vi "main_control_YJtoy_V3.vi"() -> ()   [LabVIEW 2021]
uses:
  Addons/DAQ_Pulse_Gen/DAQ_Control_2.ctl
  Addons/DAQ_Pulse_Gen/DAQ_Control_1.ctl
  Ver_2/Config_File_Paths_v2.ctl
  Ver_2/ZI_Data_v2.ctl
  Addons/DAQ_Pulse_Gen/DAQ_Control_3 .ctl
  <vilib>/Utility/file.llb/Write Delimited Spreadsheet (DBL).vi
  <vilib>/gmath/NumericalOptimization/Nonlinear Curve Fit LM formula string.vi
  <vilib>/Utility/error.llb/Error Cluster From Error Code.vi
  <vilib>/ErrorRing/Error Ring.xnode
  <vilib>/Utility/Data Type/NI_Data Type.lvlib
  <vilib>/Analysis/NI_AALPro.lvlib
  <vilib>/gmath/NI_Gmath.lvlib
panel:
  out "appended array":dbl[][](array[numeric])
  out "Initial State Numbers":i32
  out "Process name":string
  out "Initial_state_name":string
  out "tomography rotation memory (priv) 2":cluster{"Time":dbl[], dbl[]}[](array[cluster])
  out "MaxTime":dbl
  out "Process Array":cluster{"Timing 0":dbl[]}[](array[cluster])
  out "tomography rotation memory (priv)":cluster{"Time":dbl[], dbl[]}[](array[cluster])
  in  "pulses type (priv)":string[](array[string])=["None", "Y pi/2", "X pi/2"]
  in  "stop":bool
  in  "Tab Control":T1(tab)=enum."Design QPT"
  out "Config folder":string
  out "Chennel names\nare correct (?)":bool
  out "Channel map":map{string, i32}(c390)
  out "Pulses map [us]":map{string, dbl}(c390)
  out "Sampling data":T2={"Sample Numbers"=20000000, "Sample  Frequency (Hz)"=20000000}
  out "Resource Address":T3={"ZI Address"="DEV714", "VISA Keithley"="KEITHLEY"}
  in  "Save multi-process":bool
  in  "Period number":u32
  in  "Period [us]":dbl
  in  "Name of state (initial_state_)":string
  in  "Name of initial_state":u16(ring) items=["initial_state_01", "initial_state_02", "initial_state_03", "initial_state_04", "initial_state_05", "initial_state_06", "initial_state_07", "initial_state_08", "initial_state_09", "initial_state_10"]
  in  "Run tomography":bool
  in  "Run single FID":bool
  in  "Save for tomography":bool
  in  "Save single sequence":bool
  out "Pulses chart":cluster{dbl[], dbl[]}[](graph)
  in  "Reset sequence":bool
  in  "Channel":u16(ring) items=["LD pump", "LD repump", "LD probe", "pulse X", "pulse Y", "pulse Z", "Keithley ARM", "Keithley TRIG", "Accqusition TRIG", "Nonlinear coil", "None", "Tensor light shift", "pulse ZG", "AI_NI TRIG"]
  in  "Add pulse advanced":bool
  in  "Physical channels":string[](array[string])
  in  "Add pulse":bool
  in  "Time [us]":dbl
  in  "Z pi/2":bool
  in  "Z pi":bool
  in  "Y pi/2":bool
  in  "Y pi":bool
  in  "X pi/2":bool
  in  "X pi":bool
  in  "Add pumping":bool
  in  "Pumping":T4(ring)
  in  "AOC":bool
  in  "X pi/4":bool
  in  "Save initial state":bool
  in  "Save  process":bool
  in  "Name of process (process_)":string
  in  "Name of process":u16(ring) items=["process_01", "process_02", "process_03", "process_04", "process_05", "process_06", "process_07", "process_08", "process_09", "process_10"]
  in  "Y pi/4":bool
  in  "Z pi/4":bool
  in  "Save multi Sequence":bool
  in  "Clear All processes":bool
  in  "Show Process_List":bool
  in  "Delete the Process":bool
  in  "Run QPT":bool
  in  "initial_state_show":u16(ring) items=["initial_state_01.ini", "initial_state_02.ini", "initial_state_03.ini", "initial_state_04.ini", "initial_state_05.ini", "initial_state_06.ini", "initial_state_07.ini", "initial_state_08.ini", "initial_state_09.ini", "initial_state_10.ini", "initial_state_11.ini"]
  in  "Choose init states":bool
  in  "State_update":bool
  out "State_List":string[](array[string]) caption="The Choosen States"
  in  "Delete init states":bool
  in  "Show init state":bool
  in  "Process_update":bool
  in  "Process_show":u16(ring) caption="initial_state_show" items=["process_01.ini", "process_02.ini", "process_03.ini"]
  out "Pulses chart 2":cluster{dbl[], dbl[]}[](graph)
  out "Pulses chart 3":cluster{dbl[], dbl[]}[](graph)
  in  "Save QPT":bool
  in  "Clear All states":bool
  out "Process_List":string[](array[string]) caption="The Choosen Process"
  in  "Choose the Process":bool
  in  "Multi-FID":bool
  in  "save":bool
  out "Rotation signal 3":cluster{"Time":dbl[], "Array":dbl[]}[](graph)
  out "w":dbl format="%#_3f"
  out "q":dbl format="%#_3f"
  out "g2":dbl format="%#_3f"
  out "g1":dbl format="%#_3f"
  out "C":dbl format="%#_3f"
  out "B":dbl format="%#_3f"
  out "A":dbl format="%#_3f"
  in  "Enum":T5(ring)
  in  "Fit model":bool
  out "Rotation signal":cluster{"Time":dbl[], dbl[]}(graph)
  out "Rotation spectrum":waveform(dbl)[](graph)
  out "Differential signal":cluster{"Time":dbl[], "X":dbl[]}[](graph)
  out "Intensity signal":cluster{"Time":dbl[], dbl[]}(graph)
  out "Polarimeter":dbl(knob) scale=-10.0..10.0
  in  "Run single FID 2":bool
  out "Progress":dbl(slide) scale=0.0..100.0
  in  "Number of repetition":u32=1 min=1 step=1
  in  "Signal in X or Y (?)":bool
  in  "Plot type":u16(ring) items=["None + [ None ]", "None + [ Y pi ]", "None + [ Z(pi/2)+Y(pi) ]", "Y pi/2 + [ None ]", "Y pi/2 + [ Y pi ]", "Y pi/2 + [ Z(pi/2)+Y(pi) ]", "X pi/2 + [ None ]", "X pi/2 + [ Y pi ]", "X pi/2 + [ Z(pi/2)+Y(pi) ]"]
  in  "Save raw data (?)":bool
  in  "Save CYCLOPS data (?)":bool
  out "Rotation signal":cluster{"Time":dbl[], dbl[]}(graph)
  in  "Run tomography 2":bool
  in  "Averaging":u8=1 min=1 step=1
  out "Differential signal":cluster{"Time":dbl[], "X":dbl[]}[](graph)
  out "Intensity signal":cluster{"Time":dbl[], dbl[]}(graph)
  out "Progress":dbl(slide) scale=0.0..100.0
  out "Rotation spectrum":waveform(dbl)[](graph)
  out "Rotation":cluster{"Time":dbl[], dbl[]}(graph)
  in  "Save raw data  2":bool
  in  "Save CYCLOPS data 2":bool
  out "Rotation spectrum 2":waveform(dbl)[](graph)
  out "Rotation signal 2":cluster{"Time":dbl[], dbl[]}(graph)
  out "Differential signal 2":cluster{"Time":dbl[], "X":dbl[]}[](graph)
  out "Intensity signal 2":cluster{"Time":dbl[], dbl[]}(graph)
  out "Single Tomography Progress":dbl(slide) scale=0.0..100.0
  out "Rotation 2":cluster{"Time":dbl[], dbl[]}(graph)
  in  "Averaging 2":u8=1 min=1 step=1
  in  "Run QPT 2":bool
  out "Current_QPT_order":i32
  out "QPT Progress":dbl(slide) scale=0.0..100.0
  # "To change that tab you need to go to block diagram"
  # "Probing will be added during saving"
  # "X"
  # "Y"
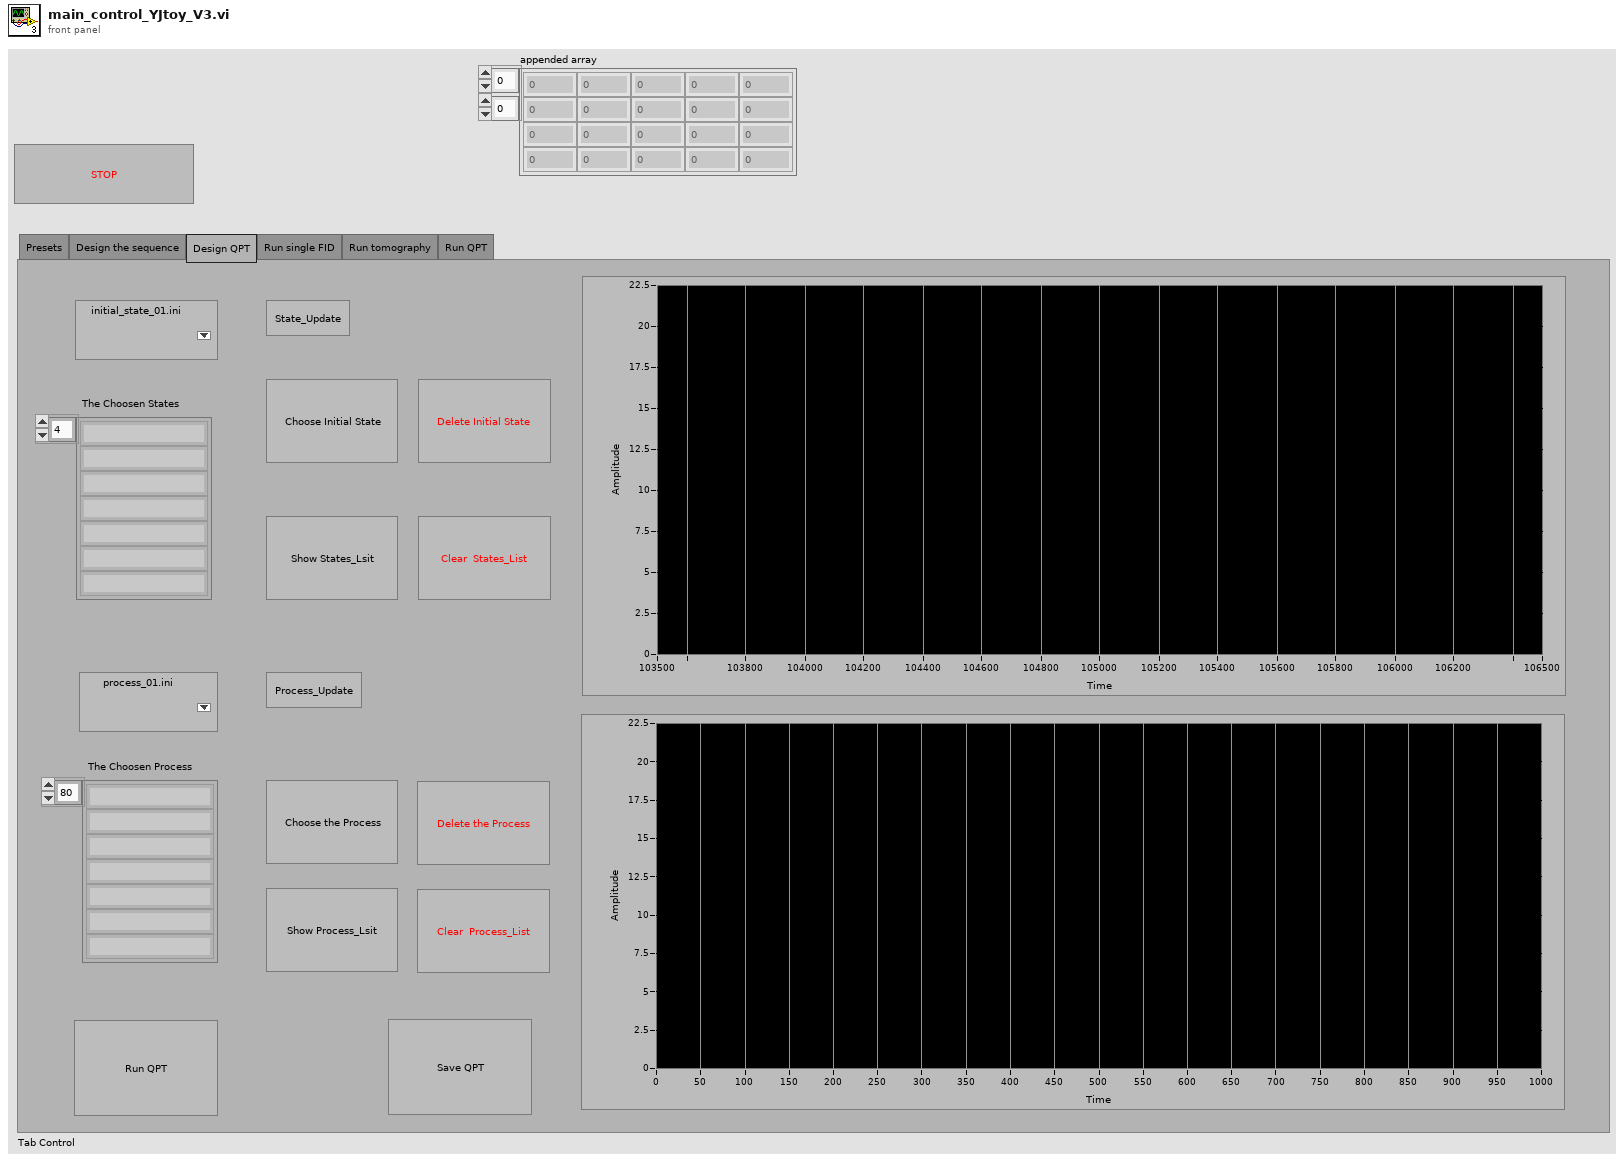
[diagram p1: front panel]
types:
  T1 = enum32{"Presets", "Design the sequence", "Design QPT", "Run single FID", "Run tomography", "Run QPT"}
  T2 = typedef "DAQ_Control_2.ctl" = cluster{"Sample Numbers":u32, "Sample  Frequency (Hz)":u32}
  T3 = cluster{"ZI Address":string, "VISA Keithley":refnum<visa-resource-name>}
  T4 = enum16{"Circular along X", "Linear in Y", "Linear in Z"}
  T5 = enum16{"Full", "A*Sin(w*t+q)*Exp(-g1*t)+C", "B*Exp(-q2*t)+C"}
  T6 = typedef "DAQ_Control_1.ctl" = cluster{"Port 2/line 6":cluster{"Timing 22":dbl[]}, "Port 2/line 5":cluster{"Timing 21":dbl[]}, "Port 2/line 4":cluster{"Timing 20":dbl[]}, "Port 2/line 3":cluster{"Timing 19":dbl[]}, "Port 2/line 2":cluster{"Timing 18":dbl[]}, "Port 2/line 1":cluster{"Timing 17":dbl[]}, "Port 2/line 0":cluster{"Timing 16":dbl[]}, "Port 1/line 7":cluster{"Timing 15":dbl[]}, "Port 1/line 6":cluster{"Timing 14":dbl[]}, "Port 1/line 5":cluster{"Timing 13":dbl[]}, "Port 1/line 4":cluster{"Timing 12":dbl[]}, "Port 1/line 3":cluster{"Timing 11":dbl[]}, "Port 1/line 2":cluster{"Timing 10":dbl[]}, "Port 1/line 1":cluster{"Timing 9":dbl[]}, "Port 1/line 0":cluster{"Timing 8":dbl[]}, "Port 0/line 7":cluster{"Timing 7\n":dbl[]}, "Port 0/line 6":cluster{"Timing 6\n":dbl[]}, "Port 0/line 5":cluster{"Timing 5\n":dbl[]}, "Port 0/line 4":cluster{"Timing 4\n":dbl[]}, "Port 0/line 3":cluster{"Timing 3\n":dbl[]}, "Port 0/line 2":cluster{"Timing 2":dbl[]}, "Port 0/line 1":cluster{"Timing 1\n":dbl[]}, "Port 0/line 0":cluster{"Timing 0":dbl[]}}
  T7 = typedef "Config_File_Paths_v2.ctl" = cluster{"ZI config file (.ini)":string, "Keithley config file (.ini)":string, "DAQ config file (.ini)":string}
  T8 = enum32{"Presets", "Design the sequence", "Design QPT", "Run single FID"}
  T9 = enum8{"Enabled", "Disabled", "Disabled and Grayed Out"}
  T10 = enum32{"Presets", "Design the sequence", "Design QPT", "Run single FID", "Run tomography"}
  T11 = cluster{"model":string, "Parameters":string[], "x":string}
  T12 = typedef "DAQ_Control_3 .ctl" = cluster{"Time Unit":enum16{"NanoSecond", "MicroSecond", "MilliSecond"}}
  T13 = typedef "ZI_Data_v2.ctl" = cluster{"R":dbl[], "Theta":dbl[], "X":dbl[], "Y":dbl[], "AuxIn0":dbl[], "AuxIn1":dbl[], "Frequency":dbl[], "DIO":dbl[], "Time":dbl[]}
  T14 = typedef "Resources_v2.ctl" = cluster{"ZI Handle":T15, "ZI ModHandle":T16, "VISA Keithley":refnum<visa-resource-name>}
  T15 = typedef "Zurich Instruments LabOne.lvlib/ziTypeHandle.ctl" = cluster{"handleValid":bool, "Conn":u64, "Path Prefix":string, "Handle":u64, "Clockbase(s)":dbl, "Connected":bool}
  T16 = typedef "Zurich Instruments LabOne.lvlib/ziTypeModHandle.ctl" = cluster{"handleValid":bool, "Conn":u64, "ModHandle":u64, "moduleID":string, "Path Prefix":string}
  T17 = typedef "Cutted_Data_v2.ctl" = cluster{"X":dbl[], "Y":dbl[], "Time":dbl[]}
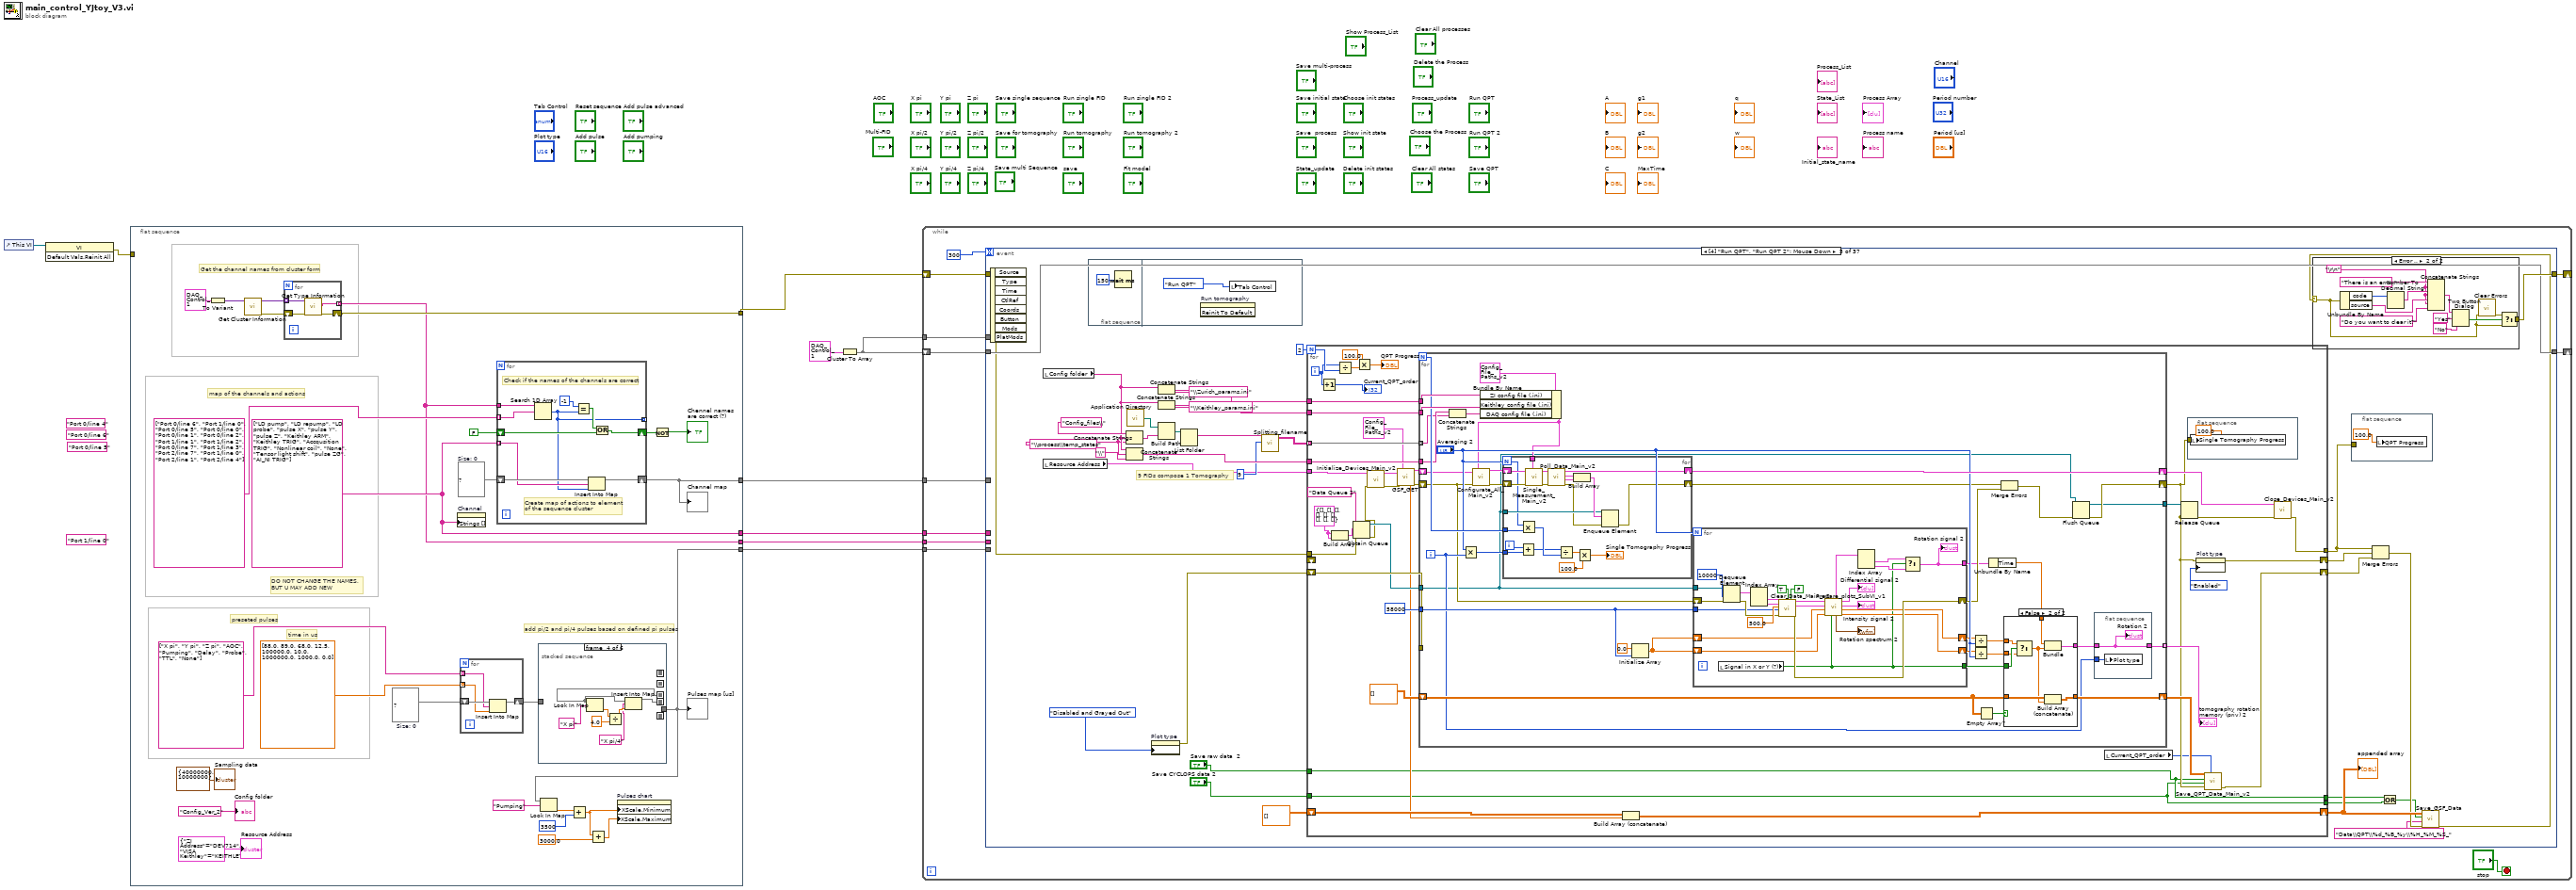
[diagram p0: block diagram]
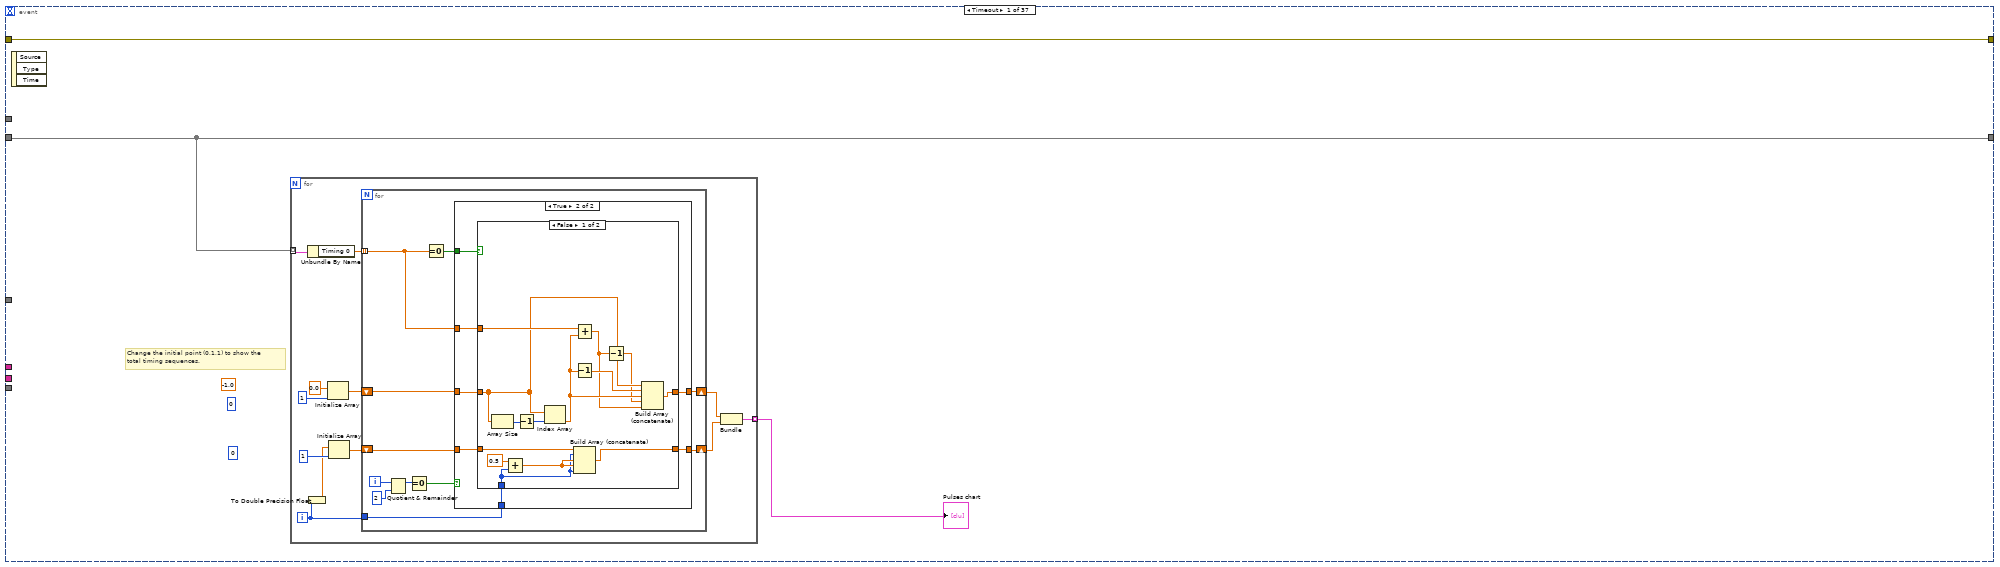
[diagram p2: hidden frame]
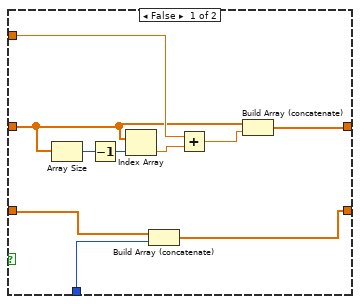
[diagram p3: hidden frame]
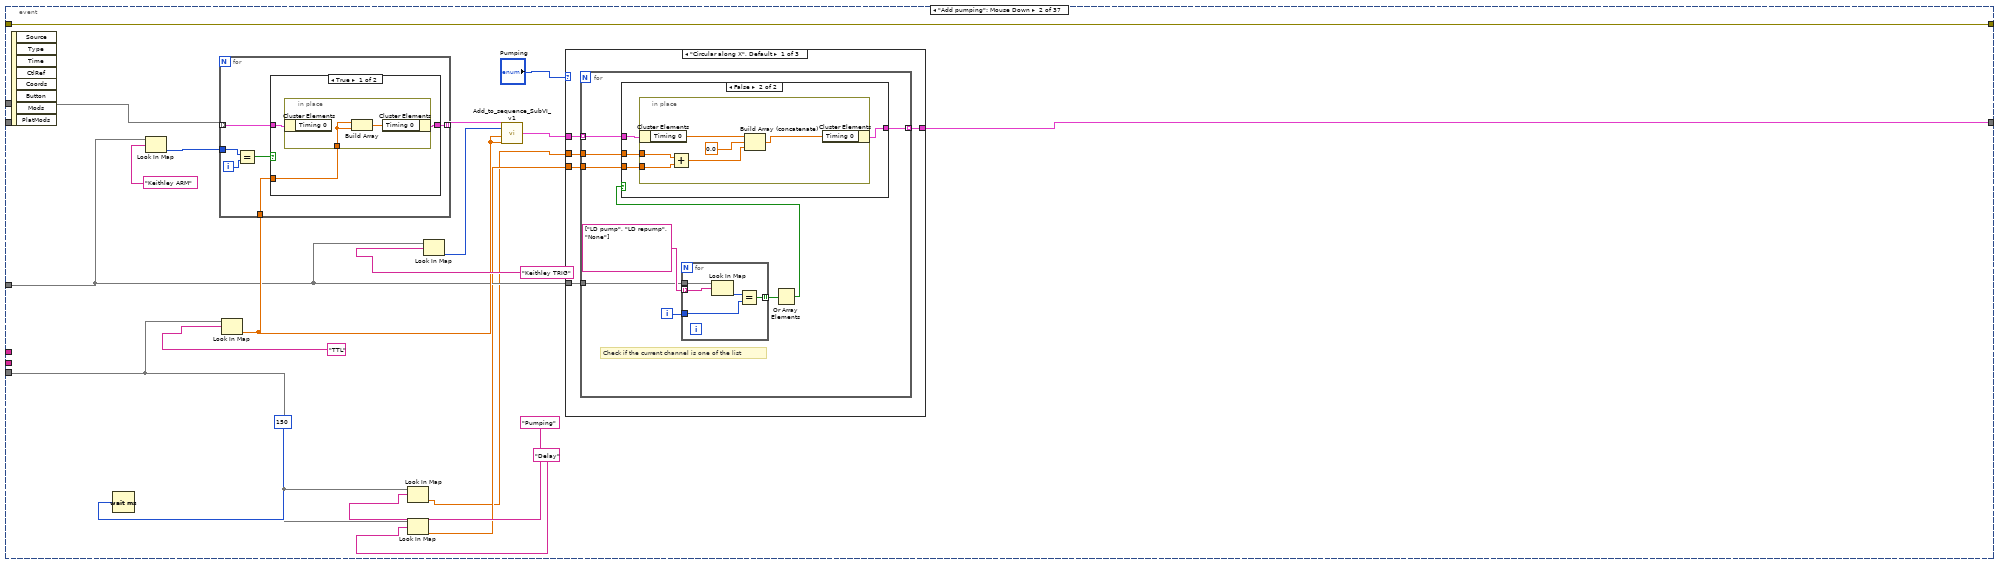
[diagram p5: hidden frame]
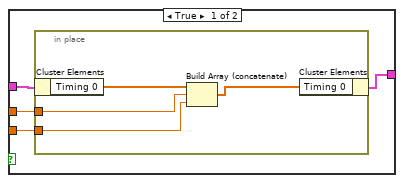
[diagram p6: hidden frame]
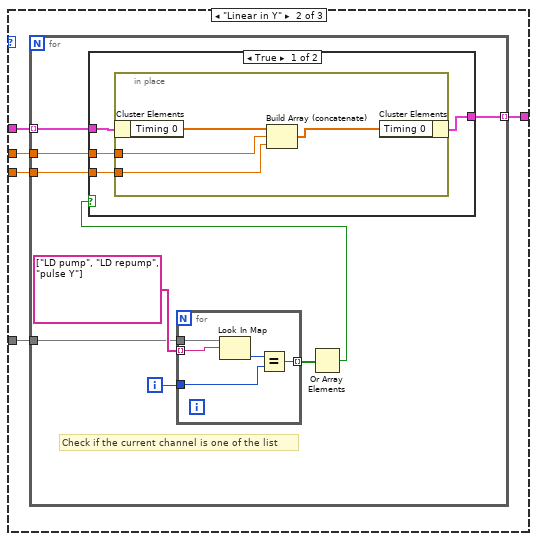
[diagram p7: hidden frame]
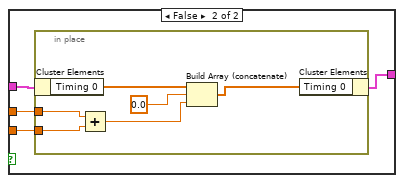
[diagram p8: hidden frame]
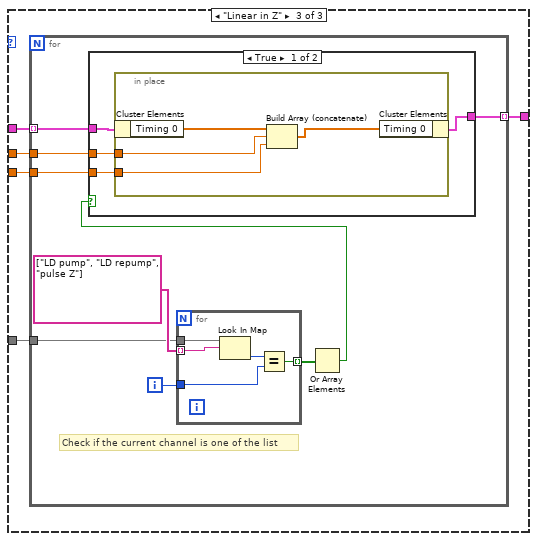
[diagram p9: hidden frame]
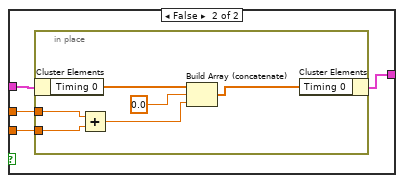
[diagram p10: hidden frame]
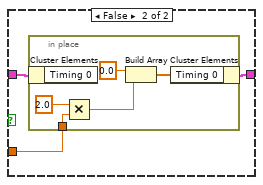
[diagram p11: hidden frame]
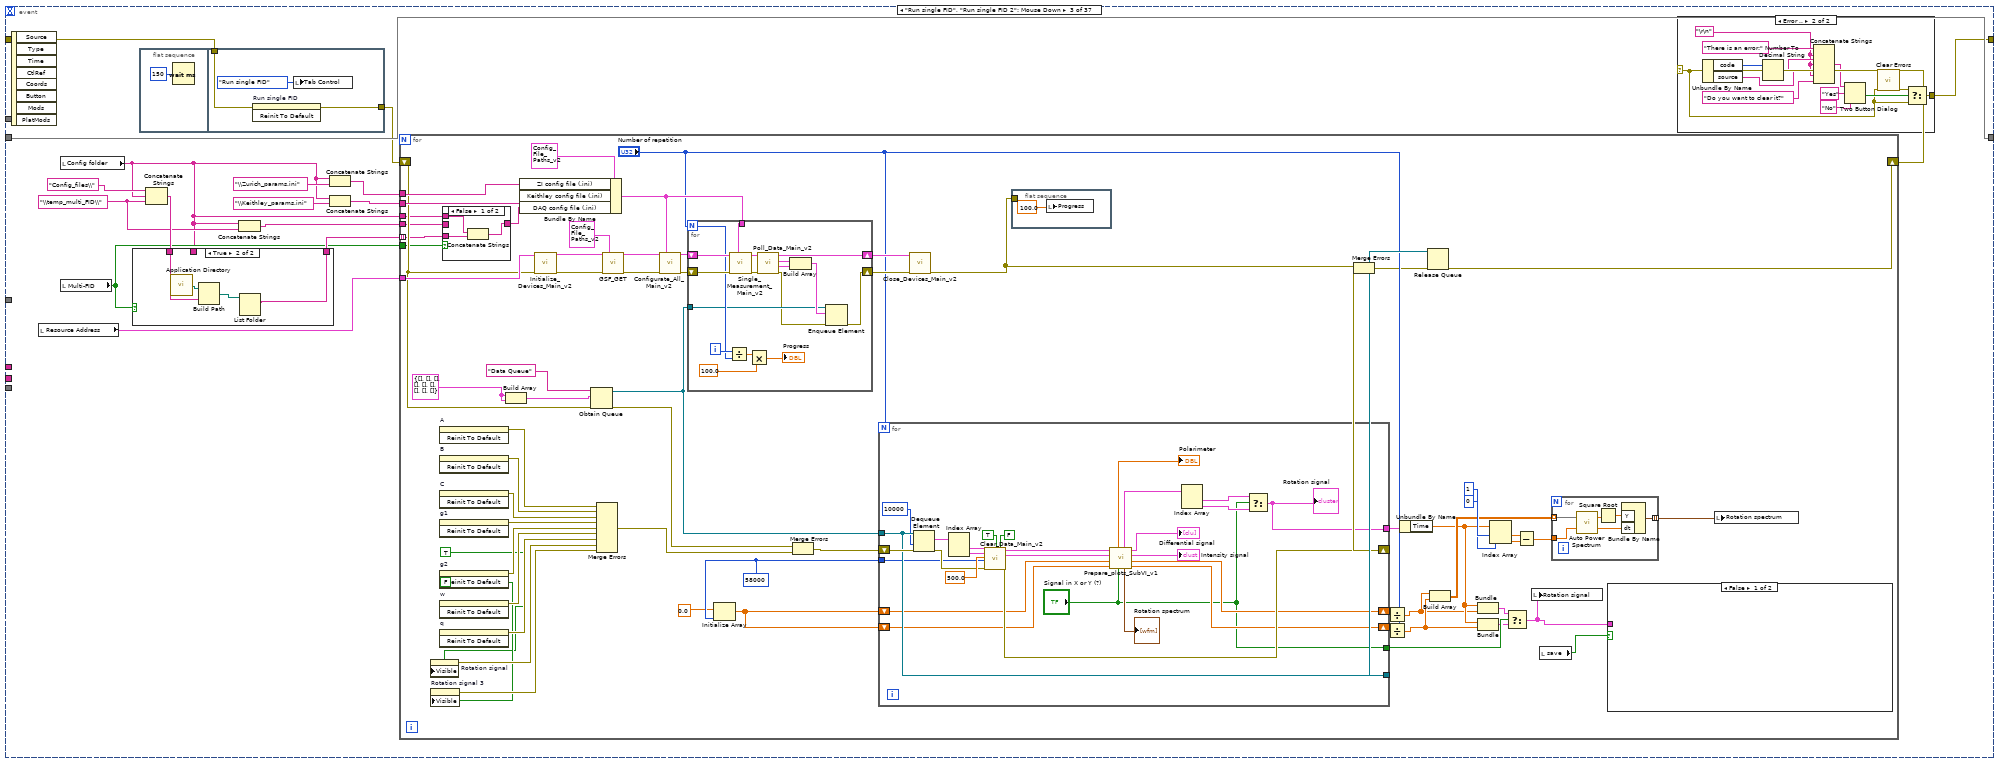
[diagram p12: hidden frame]
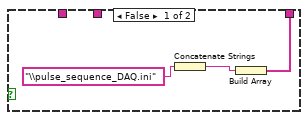
[diagram p13: hidden frame]
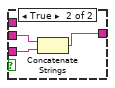
[diagram p14: hidden frame]
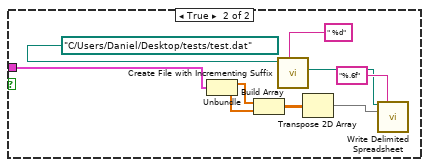
[diagram p15: hidden frame]
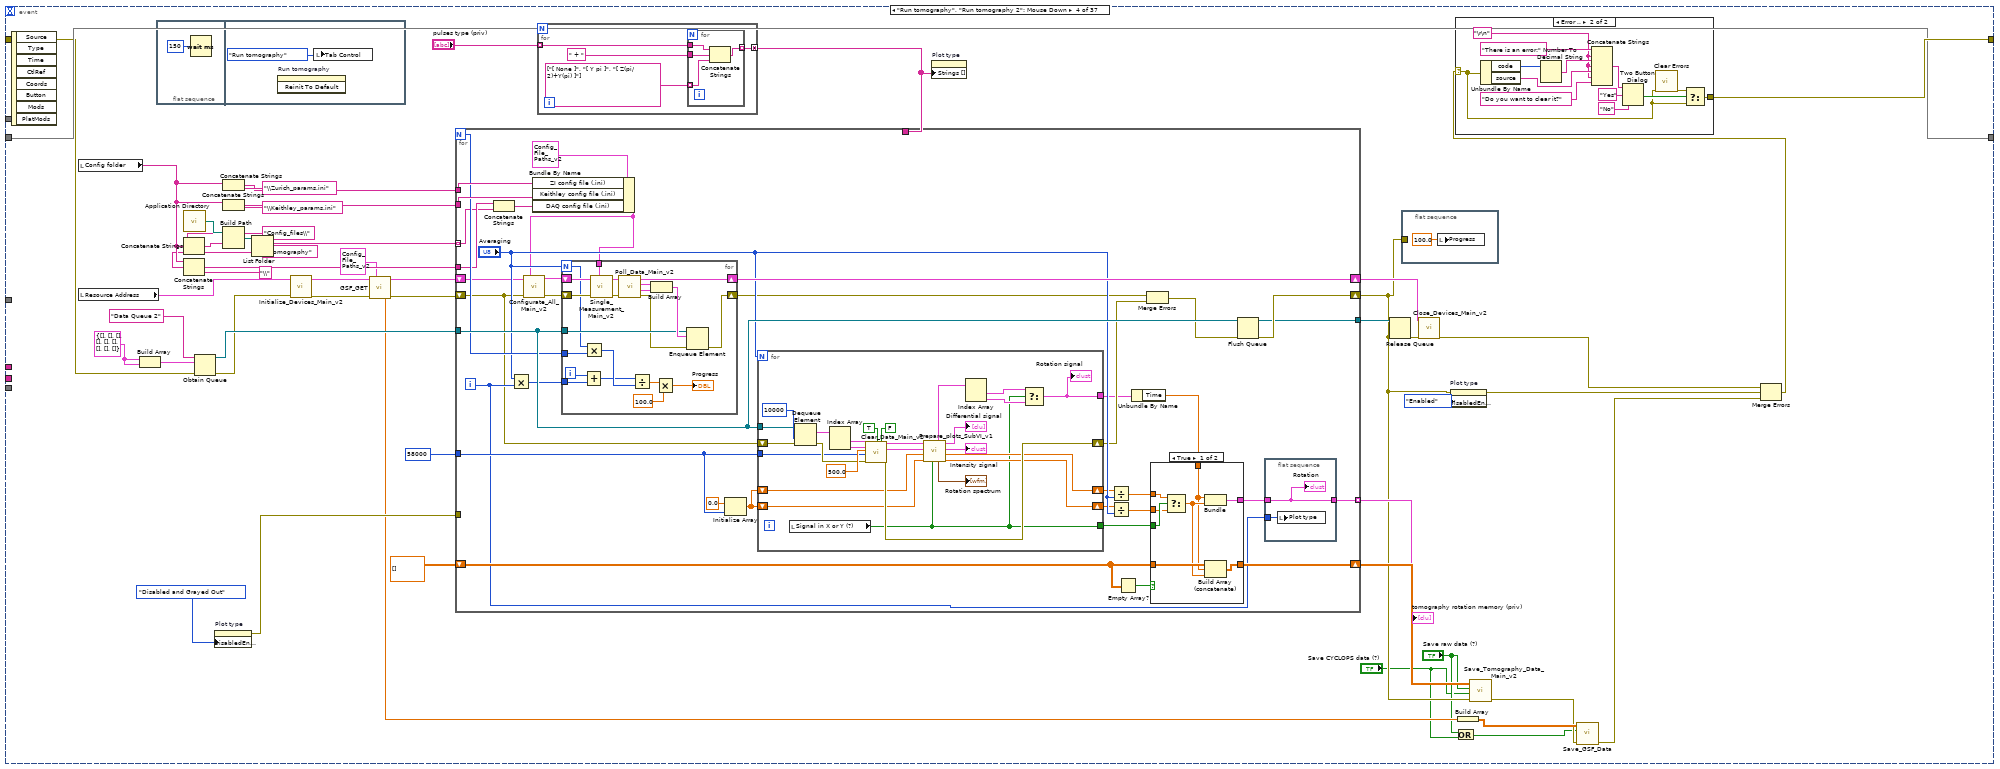
[diagram p17: hidden frame]
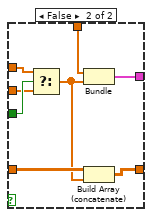
[diagram p18: hidden frame]
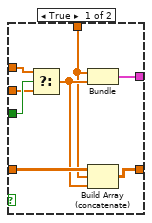
[diagram p20: hidden frame]
diagram:
  (unwired) "Port 0/line 5"
  (unwired) "Port 0/line 4"
  (unwired) "Port 1/line 0"
  (unwired) "Port 0/line 6"
  n1 = control-ref of="This VI"() -> (w2:refnum<vi>)
  n2 = invoke class="VI" method="Default Vals.Reinit All"(reference=w2) -> (error out=w1:errorcluster)  [unwired: 2 in, 2 out]
  n3 = flat-sequence {
    tunnel: [w23] -> w8
    tunnel: [w17] -> w7
    tunnel: [w22] -> w6
    tunnel: [w21] -> w5
    tunnel: [w20] -> w4
    tunnel: w1 -> [_]
    frame #0 {
      w27 = map{string, dbl} {}  # Size: 0
      w29 = map{string, i32} {}  # Size: 0
      w21 = string[] ["LD pump", "LD repump", "LD probe", "pulse X", "pulse Y", "pulse Z", "Keithley ARM", "Keithley TRIG", "Accqusition TRIG", "Nonlinear coil", "None", "Tensor light shift", "pulse ZG", "AI_NI TRIG"]
      # "DO NOT CHANGE THE NAMES,\nBUT U MAY ADD NEW"
      # "add pi/2 and pi/4 pulses based on defined pi pulses"
      # "preseted pulses"
      # "time in us"
      # "map of the channels and actions"
      # "Get the channel names from cluster form"
      n4 = To Variant(anything=T6 {"Port 2/line 6"={"Timing 22"=[]}, "Port 2/line 5"={"Timing 21"=[]}, "Port 2/line 4"={"Timing 20"=[]}, "Port 2/line 3"={"Timing 19"=[]}, "Port 2/line 2"={"Timing 18"=[]}, "Port 2/line 1"={"Timing 17"=[]}, "Port 2/line 0"={"Timing 16"=[]}, "Port 1/line 7"={"Timing 15"=[]}, "Port 1/line 6"={"Timing 14"=[]}, "Port 1/line 5"={"Timing 13"=[]}, "Port 1/line 4"={"Timing 12"=[]}, "Port 1/line 3"={"Timing 11"=[]}, "Port 1/line 2"={"Timing 10"=[]}, "Port 1/line 1"={"Timing 9"=[]}, "Port 1/line 0"={"Timing 8"=[]}, "Port 0/line 7"={"Timing 7\n"=[]}, "Port 0/line 6"={"Timing 6\n"=[]}, "Port 0/line 5"={"Timing 5\n"=[]}, "Port 0/line 4"={"Timing 4\n"=[]}, "Port 0/line 3"={"Timing 3\n"=[]}, "Port 0/line 2"={"Timing 2"=[]}, "Port 0/line 1"={"Timing 1\n"=[]}, "Port 0/line 0"={"Timing 0"=[]}} ("Sequence")) -> (Variant=w35:variant)
      n5 = call <vilib>:"Get Cluster Information.vi"("variant"=w35) -> ("error out"=w34:errorcluster, "cluster elements"=w33:variant[])  [unwired: 9 in]
      n6 = for {
        tunnel: w33 -> [w96] mode=indexing
        shift-right: [w94] -> w22
        shift-left: w34 -> [w95]
        tunnel: [w93] -> w20 mode=indexing
        n7 = call <vilib>:"Get Type Information.vi"("error in (no error)"=w95, "variant"=w96) -> ("error out"=w94:errorcluster, "name"=w93:string)  [unwired: 5 in, 3 out]
      }
      n8 = property on="Channel" class="Ring (strict)"("Strings []"=w21) -> ()  [unwired: 2 in, 2 out]
      n9 = for {
        shift-right: [w79] -> w24
        shift-left: w27 -> [w82]
        tunnel: string[] ["X pi", "Y pi", "Z pi", "AOC", "Pumping", "Delay", "Probe", "TTL", "None"] -> [w81] mode=indexing
        tunnel: dbl[] [88.0, 89.0, 68.0, 12.5, 100000.0, 10.0, 1000000.0, 1000.0, 0.0] -> [w80] mode=indexing
        n10 = Insert Into Map(map in=w82, key=w81, value=w80) -> (map out=w79:map{string, dbl})  [unwired: 2 out]
      }
      n11 = for {
        tunnel: w20 -> [w92]
        tunnel: string[] ["Port 0/line 6", "Port 1/line 0", "Port 0/line 5", "Port 0/line 0", "Port 0/line 1", "Port 0/line 2", "Port 1/line 1", "Port 1/line 2", "Port 0/line 7", "Port 1/line 3", "Port 2/line 7", "Port 1/line 0", "Port 2/line 1", "Port 2/line 4"] -> [w83] mode=indexing
        shift-right: [w88] -> w31
        shift-left: FALSE -> [w89]
        tunnel: [w85] -> _ mode=indexing
        shift-right: [w84] -> w23
        shift-left: w29 -> [w87]
        tunnel: w21 -> [w86] mode=indexing
        # "Create map of actions to element\nof the sequence cluster"
        # "Check if the names of the channels are correct"
        n12 = Search 1D Array(1D array=w92, element=w83) -> (index of element=w85:i32)  [unwired: 1 in]
        n13 = Equal?(x=-1, y=w85) -> (x = y?=w90:bool)
        n14 = Insert Into Map(map in=w87, key=w86, value=w85) -> (map out=w84:map{string, i32})  [unwired: 2 out]
        n15 = Or(x=w90, y=w89) -> (x .or. y?=w88:bool)
      }
      "Channel map" <- w23
      n16 = stacked-sequence {
        seq-local: [w37 _ _ _ _ _] -> [_ w44 _ _ _ _]
        seq-local: [_ w45 _ _ _ _] -> [_ _ w52 _ _ _]
        seq-local: [_ _ w51 _ _ _] -> [_ _ _ w63 _ _]
        seq-local: [_ _ _ w59 _ _] -> [_ _ _ _ w71 _]
        seq-local: [_ _ _ _ w70 _] -> [_ _ _ _ _ w78]
        tunnel: w24 -> [w41 _ _ _ _ _]
        tunnel: [_ _ _ _ _ w77] -> w17
        frame #0 {
          n17 = Look In Map(map=w41, key="X pi") -> (value=w39:dbl)  [unwired: 1 in, 1 out]
          n18 = Divide(x=w39, y=2.0) -> (x/y=w40:dbl)
          n19 = Insert Into Map(map in=w41, key="X pi/2", value=w40) -> (map out=w37:map{string, dbl})  [unwired: 2 out]
        }
        frame #1 {
          n20 = Look In Map(map=w44, key="Y pi") -> (value=w50:dbl)  [unwired: 1 in, 1 out]
          n21 = Divide(x=w50, y=2.0) -> (x/y=w49:dbl)
          n22 = Insert Into Map(map in=w44, key="Y pi/2", value=w49) -> (map out=w45:map{string, dbl})  [unwired: 2 out]
        }
        frame #2 {
          n23 = Look In Map(map=w52, key="Z pi") -> (value=w54:dbl)  [unwired: 1 in, 1 out]
          n24 = Divide(x=w54, y=2.0) -> (x/y=w55:dbl)
          n25 = Insert Into Map(map in=w52, key="Z pi/2", value=w55) -> (map out=w51:map{string, dbl})  [unwired: 2 out]
        }
        frame #3 {
          n26 = Look In Map(map=w63, key="X pi") -> (value=w62:dbl)  [unwired: 1 in, 1 out]
          n27 = Divide(x=w62, y=4.0) -> (x/y=w60:dbl)
          n28 = Insert Into Map(map in=w63, key="X pi/4", value=w60) -> (map out=w59:map{string, dbl})  [unwired: 2 out]
        }
        frame #4 {
          n29 = Look In Map(map=w71, key="Y pi") -> (value=w68:dbl)  [unwired: 1 in, 1 out]
          n30 = Divide(x=w68, y=4.0) -> (x/y=w66:dbl)
          n31 = Insert Into Map(map in=w71, key="Y pi/4", value=w66) -> (map out=w70:map{string, dbl})  [unwired: 2 out]
        }
        frame #5 {
          n32 = Look In Map(map=w78, key="Z pi") -> (value=w75:dbl)  [unwired: 1 in, 1 out]
          n33 = Divide(x=w75, y=4.0) -> (x/y=w73:dbl)
          n34 = Insert Into Map(map in=w78, key="Z pi/4", value=w73) -> (map out=w77:map{string, dbl})  [unwired: 2 out]
        }
      }
      "Pulses map [us]" <- w17
      n35 = Look In Map(map=w17, key="Pumping") -> (value=w19:dbl)  [unwired: 1 in, 1 out]
      n36 = Add(x=w19, y=3500) -> (x+y=w16:dbl)
      n37 = Add(x=w16, y=3000.0) -> (x+y=w14:dbl)
      n38 = property on="Pulses chart" class="XYGraph (strict)"("XScale.Minimum"=w16, "XScale.Maximum"=w14) -> ()  [unwired: 2 in, 2 out]
      n39 = Not(x=w31) -> (.not. x?=→"Chennel names\nare correct (?)":bool)
      "Sampling data" <- T2 {"Sample Numbers"=40000000, "Sample  Frequency (Hz)"=10000000} ("Sampling data")
      "Config folder" <- "Config_Ver_2" ("Filename (ini)")
      "Resource Address" <- T3 {"ZI Address"="DEV714", "VISA Keithley"="KEITHLEY"} ("Resource Address")
    }
  }
  n40 = Cluster To Array(cluster=T6 {"Port 2/line 6"={"Timing 22"=[]}, "Port 2/line 5"={"Timing 21"=[]}, "Port 2/line 4"={"Timing 20"=[]}, "Port 2/line 3"={"Timing 19"=[]}, "Port 2/line 2"={"Timing 18"=[]}, "Port 2/line 1"={"Timing 17"=[]}, "Port 2/line 0"={"Timing 16"=[]}, "Port 1/line 7"={"Timing 15"=[]}, "Port 1/line 6"={"Timing 14"=[]}, "Port 1/line 5"={"Timing 13"=[]}, "Port 1/line 4"={"Timing 12"=[]}, "Port 1/line 3"={"Timing 11"=[]}, "Port 1/line 2"={"Timing 10"=[]}, "Port 1/line 1"={"Timing 9"=[]}, "Port 1/line 0"={"Timing 8"=[]}, "Port 0/line 7"={"Timing 7\n"=[]}, "Port 0/line 6"={"Timing 6\n"=[]}, "Port 0/line 5"={"Timing 5\n"=[]}, "Port 0/line 4"={"Timing 4\n"=[]}, "Port 0/line 3"={"Timing 3\n"=[]}, "Port 0/line 2"={"Timing 2"=[]}, "Port 0/line 1"={"Timing 1\n"=[]}, "Port 0/line 0"={"Timing 0"=[]}} ("Sequence")) -> (array=w3:cluster{"Timing 0":dbl[]}[])
  n41 = while {
    shift-right: [w98] -> _
    shift-left: w3 -> [w107]
    tunnel: w8 -> [w106]
    tunnel: w7 -> [w97]
    shift-right: [w102] -> _
    shift-left: w6 -> [w103]
    tunnel: w5 -> [w101]
    tunnel: w4 -> [w100]
    tunnel: w3 -> [w99]
    stop <- "stop" stop-if-true
    n42 = event shown="[4] \"Run QPT\", \"Run QPT 2\": Mouse Down" {
      selector: _ -> [_ _ _ _ _ _ _ _ _ _ _ _ _ _ _ _ _ _ _ _ _ _ _ _ _ _ _ _ _ _ _ _ _ _ _ _ _]
      dyn-events: _ -> [_ _ _ _ _ _ _ _ _ _ _ _ _ _ _ _ _ _ _ _ _ _ _ _ _ _ _ _ _ _ _ _ _ _ _ _ _]
      timeout: 300 -> [_ _ _ _ _ _ _ _ _ _ _ _ _ _ _ _ _ _ _ _ _ _ _ _ _ _ _ _ _ _ _ _ _ _ _ _ _]
      tunnel: w107 -> [w110 _ w327 w530 w693 w862 _ w1025 w1030 w1042 w1053 w1065 w1077 w1089 w1101 w1113 w1125 w1142 w1170 w1209 w1290 w1421 w1475 w1617 w1664 _ _ _ _ _ _ _ _ _ _ _ _]
      tunnel: w106 -> [_ w172 _ _ _ _ _ w1009 w1037 w1049 w1060 w1072 w1084 w1096 w1108 w1120 w1132 w1147 _ w1222 w1292 w1423 w1480 _ _ w1737 _ _ _ _ _ _ _ _ _ _ _]
      tunnel: w97 -> [_ w171 _ _ _ _ _ w1007 w1031 w1043 w1058 w1066 w1078 w1090 w1102 w1114 w1126 w1143 w1162 w1219 w1291 w1422 w1479 _ _ w1736 _ _ _ _ _ _ _ _ _ _ _]
      tunnel: [w110 w169 w327 w530 w693 w862 _ w1002 w1029 w1041 w1052 w1064 w1076 w1088 w1100 w1112 w1124 w1141 w1159 w1209 _ _ w1475 w1617 w1664 _ _ _ _ _ _ _ _ _ _ _ w2190] -> w98
      tunnel: w103 -> [w109 w185 w326 w526 w678 w863 w905 w1013 w1033 w1045 _ w1068 w1080 w1092 w1104 w1116 w1128 w1145 w1166 w1204 w1282 w1413 w1473 w1618 w1665 w1720 w1852 w1947 w2045 w2068 w2083 w2104 w2125 w2153 w2181 w2187 w2191]
      tunnel: [w109 w185 w324 w534 w696 w863 _ w1013 w1033 w1045 _ w1068 w1080 w1092 w1104 w1116 w1128 w1145 w1166 w1203 w1289 w1420 w1472 w1619 w1666 w1743 w1851 w1940 w2040 w2063 w2090 w2111 w2122 w2150 w2180 w2186 w2191] -> w102
      tunnel: w101 -> [_ _ _ _ _ _ _ _ _ _ _ _ _ _ _ _ _ w1138 _ _ _ _ _ _ _ _ _ _ _ _ _ _ _ _ _ _ _]
      tunnel: w100 -> [_ _ _ _ _ _ _ _ _ _ _ _ _ _ _ _ _ _ w1168 _ _ _ _ _ _ _ _ _ _ _ _ _ _ _ _ _ _]
      tunnel: w99 -> [_ w168 _ _ _ _ _ _ _ _ _ _ _ _ _ _ _ _ _ _ _ _ _ _ _ _ _ _ _ _ _ _ _ _ _ _ w2190]
      event Timeout {
        (unwired) 0 ("dimension size")
        (unwired) 0 ("dimension size")
        (unwired) -1.0 ("element")
        # "Change the initial point (0,1,1) to show the \ntotal timing sequences."
        n43 = event-data() -> ()  [unwired: 1 in, 3 out]
        n44 = for {
          tunnel: w110 -> [w122] mode=indexing
          tunnel: [w111] -> w108 mode=indexing
          i -> [w114]
          n45 = To Double Precision Float(number=w114) -> (double precision float=w118:dbl)
          n46 = Unbundle By Name(w122) -> ("Timing 0"=w121:dbl[])
          n47 = Initialize Array(0.0 ("element"), 1 ("dimension size")) -> (w115:dbl[])
          n48 = Initialize Array(w118, 1 ("dimension size")) -> (w119:dbl[])
          n49 = for {
            tunnel: w121 -> [w124] mode=indexing
            shift-right: [w126] -> w112
            shift-left: w119 -> [w125]
            shift-right: [w128] -> w113
            shift-left: w115 -> [w127]
            tunnel: w114 -> [w123]
            i -> [w133]
            n50 = Quotient & Remainder(x=w133, y=2) -> (x-y*floor(x/y)=w131:i32)  [unwired: 1 out]
            n51 = Equal To 0?(x=w131) -> (x = 0?=w130:bool)
            n52 = Equal To 0?(x=w124) -> (x = 0?=w129:bool)
            n53 = case shown="True" w130 {
              tunnel: w129 -> [_ w150]
              tunnel: [w134 w149] -> w128
              tunnel: w127 -> [w136 w148]
              tunnel: [w141 w147] -> w126
              tunnel: w125 -> [w142 w146]
              tunnel: w124 -> [w137 w145]
              tunnel: w123 -> [w143 w144]
              frame False {
                n54 = Array Size(array=w136) -> (size(s)=w140:i32)
                n55 = Decrement(x=w140) -> (x-1=w139:i32)
                n56 = Index Array(array=w136, index=w139) -> (element=w138:dbl)
                n57 = Build Array (concatenate)(w142, w143) -> (w141:dbl[])
                n58 = Add(x=w137, y=w138) -> (x+y=w135:dbl)
                n59 = Build Array (concatenate)(w136, w135) -> (w134:dbl[])
              }
              frame True {
                n60 = case shown="False" w150 {
                  tunnel: [w161 w166] -> w149
                  tunnel: w148 -> [w155 w166]
                  tunnel: [w157 w165] -> w147
                  tunnel: w146 -> [w164 w165]
                  tunnel: w145 -> [w162 _]
                  tunnel: w144 -> [w158 _]
                  frame False {
                    n61 = Array Size(array=w155) -> (size(s)=w163:i32)
                    n62 = Add(x=0.5, y=w158) -> (x+y=w159:dbl)
                    n63 = Decrement(x=w163) -> (x-1=w156:i32)
                    n64 = Index Array(array=w155, index=w156) -> (element=w153:dbl)
                    n65 = Add(x=w162, y=w153) -> (x+y=w152:dbl)
                    n66 = Decrement(x=w153) -> (x-1=w154:dbl)
                    n67 = Build Array (concatenate)(w164, w158, w159, w159, w158) -> (w157:dbl[])
                    n68 = Decrement(x=w152) -> (x-1=w151:dbl)
                    n69 = Build Array (concatenate)(w155, w154, w153, w151, w152) -> (w161:dbl[])
                  }
                  frame True {
                  }
                }
              }
            }
          }
          n70 = Bundle(w113, w112) -> (w111:cluster{dbl[], dbl[]})  [unwired: 1 in]
        }
        "Pulses chart" <- w108
      }
      event "Add pumping": Mouse Down {
        n71 = event-data() -> ()  [unwired: 1 in, 8 out]
        n72 = Wait (ms)(milliseconds to wait=u32 150) -> ()  [unwired: 1 out]
        n73 = Look In Map(map=w172, key="Keithley ARM") -> (value=w182:i32)  [unwired: 1 in, 1 out]
        n74 = Look In Map(map=w171, key="TTL") -> (value=w177:dbl)  [unwired: 1 in, 1 out]
        n75 = for {
          tunnel: w168 -> [w299] mode=indexing
          tunnel: w182 -> [w301]
          tunnel: w177 -> [w298]
          tunnel: [w297] -> w180 mode=indexing
          i -> [w302]
          n76 = Equal?(x=w301, y=w302) -> (x = y?=w300:bool)
          n77 = case shown="True" w300 {
            tunnel: w299 -> [w305 w310]
            tunnel: w298 -> [w304 w309]
            tunnel: [w303 w308] -> w297
            frame True {
              n78 = in-place {
                in-place-border: w304 -> [w307]
                n79 = in-place-cluster #1(w305) -> ()  [unwired: 1 out]
                n80 = Build Array(w307, w307) -> (w306:dbl[])
                n81 = in-place-cluster #1("Timing 0"=w306) -> (w303:cluster{"Timing 0":dbl[]})
              }
            }
            frame False {
              n82 = in-place {
                in-place-border: w309 -> [w313]
                n83 = in-place-cluster #2(w310) -> ()  [unwired: 1 out]
                n84 = Multiply(x=2.0, y=w313) -> (x*y=w311:dbl)
                n85 = Build Array(0.0 ("element"), w311) -> (w315:dbl[])
                n86 = in-place-cluster #2("Timing 0"=w315) -> (w308:cluster{"Timing 0":dbl[]})
              }
            }
          }
        }
        n87 = Look In Map(map=w171, key="Pumping") -> (value=w167:dbl)  [unwired: 1 in, 1 out]
        n88 = Look In Map(map=w171, key="Delay") -> (value=w170:dbl)  [unwired: 1 in, 1 out]
        n89 = Look In Map(map=w172, key="Keithley TRIG") -> (value=w178:i32)  [unwired: 1 in, 1 out]
        n90 = call "Add_to_sequence_SubVI_v1.vi"("Delay [us]"=w177, "Pulse length [us]"=w177, "Channel number"=w178, "Array sequence in"=w180) -> ("Array sequence out"=w175:cluster{"Timing 0":dbl[]}[])
        n91 = case shown="\"Circular along X\", Default" "Pumping" {
          tunnel: w175 -> [w190 w227 w264]
          tunnel: w172 -> [w189 w226 w263]
          tunnel: w167 -> [w188 w225 w262]
          tunnel: w170 -> [w187 w224 w261]
          tunnel: [w186 w223 w260] -> w169
          frame "Circular along X", Default {
            n92 = for {
              tunnel: w190 -> [w194] mode=indexing
              tunnel: w189 -> [w196]
              tunnel: w188 -> [w193]
              tunnel: w187 -> [w192]
              tunnel: [w191] -> w186 mode=indexing
              i -> [w197]
              # "Check if the current channel is one of the list"
              n93 = for {
                tunnel: w196 -> [w221]
                tunnel: w197 -> [w220]
                tunnel: [w219] -> w199 mode=indexing
                tunnel: string[] ["LD pump", "LD repump", "None"] -> [w218] mode=indexing
                n94 = Look In Map(map=w221, key=w218) -> (value=w222:i32)  [unwired: 1 in, 1 out]
                n95 = Equal?(x=w222, y=w220) -> (x = y?=w219:bool)
              }
              n96 = Or Array Elements(Boolean array=w199) -> (logical OR=w195:bool)
              n97 = case shown="False" w195 {
                tunnel: w194 -> [w203 w211]
                tunnel: w193 -> [w202 w210]
                tunnel: w192 -> [w201 w209]
                tunnel: [w200 w208] -> w191
                frame True {
                  n98 = in-place {
                    in-place-border: w202 -> [w206]
                    in-place-border: w201 -> [w205]
                    n99 = in-place-cluster #3(w203) -> ("Timing 0"=w207:dbl[])
                    n100 = Build Array (concatenate)(w207, w206, w205) -> (w204:dbl[])
                    n101 = in-place-cluster #3("Timing 0"=w204) -> (w200:cluster{"Timing 0":dbl[]})
                  }
                }
                frame False {
                  n102 = in-place {
                    in-place-border: w210 -> [w215]
                    in-place-border: w209 -> [w214]
                    n103 = in-place-cluster #4(w211) -> ("Timing 0"=w217:dbl[])
                    n104 = Add(x=w215, y=w214) -> (x+y=w213:dbl)
                    n105 = Build Array (concatenate)(w217, 0.0 ("element"), w213) -> (w216:dbl[])
                    n106 = in-place-cluster #4("Timing 0"=w216) -> (w208:cluster{"Timing 0":dbl[]})
                  }
                }
              }
            }
          }
          frame "Linear in Y" {
            n107 = for {
              tunnel: w227 -> [w231] mode=indexing
              tunnel: w226 -> [w233]
              tunnel: w225 -> [w230]
              tunnel: w224 -> [w229]
              tunnel: [w228] -> w223 mode=indexing
              i -> [w234]
              # "Check if the current channel is one of the list"
              n108 = for {
                tunnel: w233 -> [w258]
                tunnel: w234 -> [w257]
                tunnel: [w256] -> w236 mode=indexing
                tunnel: string[] ["LD pump", "LD repump", "pulse Y"] -> [w255] mode=indexing
                n109 = Look In Map(map=w258, key=w255) -> (value=w259:i32)  [unwired: 1 in, 1 out]
                n110 = Equal?(x=w259, y=w257) -> (x = y?=w256:bool)
              }
              n111 = Or Array Elements(Boolean array=w236) -> (logical OR=w232:bool)
              n112 = case shown="True" w232 {
                tunnel: w231 -> [w240 w248]
                tunnel: w230 -> [w239 w247]
                tunnel: w229 -> [w238 w246]
                tunnel: [w237 w245] -> w228
                frame True {
                  n113 = in-place {
                    in-place-border: w239 -> [w243]
                    in-place-border: w238 -> [w242]
                    n114 = in-place-cluster #5(w240) -> ("Timing 0"=w244:dbl[])
                    n115 = Build Array (concatenate)(w244, w243, w242) -> (w241:dbl[])
                    n116 = in-place-cluster #5("Timing 0"=w241) -> (w237:cluster{"Timing 0":dbl[]})
                  }
                }
                frame False {
                  n117 = in-place {
                    in-place-border: w247 -> [w252]
                    in-place-border: w246 -> [w251]
                    n118 = in-place-cluster #6(w248) -> ("Timing 0"=w254:dbl[])
                    n119 = Add(x=w252, y=w251) -> (x+y=w250:dbl)
                    n120 = Build Array (concatenate)(w254, 0.0 ("element"), w250) -> (w253:dbl[])
                    n121 = in-place-cluster #6("Timing 0"=w253) -> (w245:cluster{"Timing 0":dbl[]})
                  }
                }
              }
            }
          }
          frame "Linear in Z" {
            n122 = for {
              tunnel: w264 -> [w268] mode=indexing
              tunnel: w263 -> [w270]
              tunnel: w262 -> [w267]
              tunnel: w261 -> [w266]
              tunnel: [w265] -> w260 mode=indexing
              i -> [w271]
              # "Check if the current channel is one of the list"
              n123 = for {
                tunnel: w270 -> [w295]
                tunnel: w271 -> [w294]
                tunnel: [w293] -> w273 mode=indexing
                tunnel: string[] ["LD pump", "LD repump", "pulse Z"] -> [w292] mode=indexing
                n124 = Look In Map(map=w295, key=w292) -> (value=w296:i32)  [unwired: 1 in, 1 out]
                n125 = Equal?(x=w296, y=w294) -> (x = y?=w293:bool)
              }
              n126 = Or Array Elements(Boolean array=w273) -> (logical OR=w269:bool)
              n127 = case shown="True" w269 {
                tunnel: w268 -> [w277 w285]
                tunnel: w267 -> [w276 w284]
                tunnel: w266 -> [w275 w283]
                tunnel: [w274 w282] -> w265
                frame True {
                  n128 = in-place {
                    in-place-border: w276 -> [w280]
                    in-place-border: w275 -> [w279]
                    n129 = in-place-cluster #7(w277) -> ("Timing 0"=w281:dbl[])
                    n130 = Build Array (concatenate)(w281, w280, w279) -> (w278:dbl[])
                    n131 = in-place-cluster #7("Timing 0"=w278) -> (w274:cluster{"Timing 0":dbl[]})
                  }
                }
                frame False {
                  n132 = in-place {
                    in-place-border: w284 -> [w289]
                    in-place-border: w283 -> [w288]
                    n133 = in-place-cluster #8(w285) -> ("Timing 0"=w291:dbl[])
                    n134 = Add(x=w289, y=w288) -> (x+y=w287:dbl)
                    n135 = Build Array (concatenate)(w291, 0.0 ("element"), w287) -> (w290:dbl[])
                    n136 = in-place-cluster #8("Timing 0"=w290) -> (w282:cluster{"Timing 0":dbl[]})
                  }
                }
              }
            }
          }
        }
      }
      event "Run single FID", "Run single FID 2": Mouse Down {
        w319 = "\\temp_multi_FID\\" ("string")
        n137 = event-data() -> ()  [unwired: 1 in, 8 out]
        n138 = local read "Resource Address"() -> (w332:T3)
        n139 = local read "Config folder"() -> (w316:string)
        n140 = local read "Multi-FID"() -> (w317:bool)
        n141 = flat-sequence {
          tunnel: w326 -> [w487]
          tunnel: [w486] -> w325
          frame #0 {
            n142 = Wait (ms)(milliseconds to wait=u32 150) -> ()  [unwired: 1 out]
          }
          frame #1 {
            n143 = invoke on="Run single FID" class="Bool (strict)" method="Reinit To Default"(error in=w487) -> (error out=w486:errorcluster)  [unwired: 2 in, 2 out]
            n144 = local write "Tab Control"(T8."Run single FID" ("Tab Control")) -> ()
          }
        }
        n145 = Concatenate Strings("Config_files\\" ("string"), w316, w319) -> (w320:string)
        n146 = case shown="True" w317 {
          tunnel: w320 -> [_ w337]
          tunnel: [w333 w336] -> w322
          tunnel: w316 -> [_ _]
          frame False {
            n147 = Concatenate Strings("\\pulse_sequence_DAQ.ini" ("string")) -> (w334:string)
            n148 = Build Array(w334) -> (w333:string[])
          }
          frame True {
            n149 = call <vilib>:"Application Directory.vi"() -> ("Application Directory"=w338:path)
            n150 = Build Path(base path=w338, name or relative path=w337) -> (appended path=w339:path)
            n151 = List Folder(path=w339) -> (filenames=w336:string[])  [unwired: 3 in, 3 out]
          }
        }
        n152 = Concatenate Strings(w316, w319) -> (w318:string)
        n153 = Concatenate Strings(w316, "\\Zurich_params.ini" ("string")) -> (w328:string)
        n154 = Concatenate Strings(w316, "\\Keithley_params.ini" ("string")) -> (w329:string)
        n155 = for {
          tunnel: w332 -> [w404]
          tunnel: w329 -> [w402]
          tunnel: w328 -> [w401]
          shift-right: [w364] -> w323
          shift-left: w325 -> [w394]
          tunnel: w322 -> [w349] mode=indexing
          tunnel: w318 -> [w347]
          tunnel: w317 -> [w346]
          tunnel: w316 -> [w345]
          w368 = T13 {"R"=[], "Theta"=[], "X"=[], "Y"=[], "AuxIn0"=[], "AuxIn1"=[], "Frequency"=[], "DIO"=[], "Time"=[]} ("ZI Data")
          w391 = u16 58000 ("Fixed Number Of Points")
          n156 = property on="Rotation signal" class="XYGraph (strict)"("Visible"=TRUE) -> (error out=w360:errorcluster)  [unwired: 2 in, 1 out]
          n157 = property on="Rotation signal 3" class="XYGraph (strict)"("Visible"=FALSE) -> (error out=w361:errorcluster)  [unwired: 2 in, 1 out]
          n158 = invoke on="A" class="DigNum (strict)" method="Reinit To Default"() -> (error out=w356:errorcluster)  [unwired: 3 in, 2 out]
          n159 = invoke on="B" class="DigNum (strict)" method="Reinit To Default"() -> (error out=w355:errorcluster)  [unwired: 3 in, 2 out]
          n160 = invoke on="C" class="DigNum (strict)" method="Reinit To Default"() -> (error out=w354:errorcluster)  [unwired: 3 in, 2 out]
          n161 = invoke on="g1" class="DigNum (strict)" method="Reinit To Default"() -> (error out=w353:errorcluster)  [unwired: 3 in, 2 out]
          n162 = invoke on="g2" class="DigNum (strict)" method="Reinit To Default"() -> (error out=w357:errorcluster)  [unwired: 3 in, 2 out]
          n163 = invoke on="w" class="DigNum (strict)" method="Reinit To Default"() -> (error out=w358:errorcluster)  [unwired: 3 in, 2 out]
          n164 = invoke on="q" class="DigNum (strict)" method="Reinit To Default"() -> (error out=w359:errorcluster)  [unwired: 3 in, 2 out]
          n165 = case shown="False" w346 {
            tunnel: w349 -> [w407 w410]
            tunnel: [w405 w409] -> w348
            tunnel: w347 -> [_ w408]
            tunnel: w345 -> [w406 _]
            frame False {
              n166 = Concatenate Strings(w406, w407) -> (w405:string)
            }
            frame True {
              n167 = Concatenate Strings(w408, w410) -> (w409:string)
            }
          }
          n168 = Build Array(w368, w368) -> (w367:T13[])
          n169 = Bundle By Name(cluster=T7 {"ZI config file (.ini)"="Config_Ver_2\\Zurich_params.ini", "Keithley config file (.ini)"="Config_Ver_2\\Keithley_params.ini", "DAQ config file (.ini)"="Config_Ver_2\\pulse_sequence_DAQ.ini"} ("Config files paths"), "ZI config file (.ini)"=w401, "Keithley config file (.ini)"=w402, "DAQ config file (.ini)"=w348) -> (w398:T7)
          n170 = call "Initialize_Devices_Main_v2.vi"("error in"=w394, "Resource Address"=w404) -> ("error out"=w342:errorcluster, "Resources"=w344:T14)  [unwired: 8 in]
          n171 = Obtain Queue(name (unnamed)="Data Queue", element data type=w367, error in (no error)=w394) -> (queue out=w393:refnum<queue>, error out=w370:errorcluster)  [unwired: 2 in, 1 out]
          n172 = Merge Errors(w356, w355, w354, w353, w357, w358, w359, w360, w361) -> (w350:errorcluster)
          n173 = call "GSF_GET.vi"("Resources in"=w344, "Config files paths"=T7 {"ZI config file (.ini)"="Config_Ver_2\\GSF_Zurich_params.ini", "Keithley config file (.ini)"="Config_Ver_2\\Keithley_params.ini", "DAQ config file (.ini)"="Config_Ver_2\\GSF_pulse_sequence_DAQ.ini"}, "error in"=w342) -> ("Resources out"=w343:T14, "error out"=w341:errorcluster)  [unwired: 7 in, 4 out]
          n174 = call "Configurate_All_Main_v2.vi"("Resources in"=w343, "Config files paths"=w398, "error in"=w341) -> ("Resources out"=w400:T14, "error out"=w399:errorcluster)  [unwired: 6 in, 5 out]
          n175 = for {
            N: "Number of repetition" -> [w463]
            tunnel: w398 -> [w468]
            shift-right: [w467] -> w397
            shift-left: w400 -> [w470]
            shift-right: [w455] -> w396
            shift-left: w399 -> [w469]
            tunnel: w393 -> [w458]
            i -> [w464]
            n176 = Divide(x=w464, y=w463) -> (x/y=w461:dbl)
            n177 = call "Single_Measurement_Main_v2.vi"("Config files paths"=w468, "error in"=w469, "Resources in"=w470) -> ("error out"=w465:errorcluster, "Resources out"=w466:T14)  [unwired: 6 in, 1 out]
            n178 = Multiply(x=w461, y=100.0) -> (x*y=→"Progress":dbl)
            n179 = call "Poll_Data_Main_v2.vi"("error in"=w465, "Resources in"=w466) -> ("error out"=w456:errorcluster, "ZI Data 3"=w457:T13, "ZI Data 0"=w454:T13, "Resources out"=w467:T14)  [unwired: 6 in]
            n180 = Build Array(w454, w457) -> (w459:T13[])
            n181 = Enqueue Element(queue=w458, element=w459, error in (no error)=w456) -> (error out=w455:errorcluster)  [unwired: 1 in, 2 out]
          }
          n182 = Initialize Array(0.0 ("element"), w391) -> (w389:dbl[])
          n183 = Merge Errors(w370, w350) -> (w369:errorcluster)
          n184 = for {
            N: "Number of repetition" -> [_]
            tunnel: w393 -> [w447]
            shift-right: [w444] -> w366
            shift-left: w369 -> [w449]
            tunnel: [w447] -> w392
            shift-right: [w437] -> w374
            shift-left: w389 -> [w440]
            tunnel: w391 -> [w443]
            shift-right: [w438] -> w375
            shift-left: w389 -> [w439]
            tunnel: [w426] -> w388
            tunnel: ["Signal in X or Y (?)"] -> w387
            n185 = Dequeue Element(queue=w447, timeout in ms (-1)=10000, error in (no error)=w449) -> (element=w448:T13[], error out=w445:errorcluster)  [unwired: 2 out]
            n186 = Index Array(array=w448) -> (element #1=w428:T13, element #2=w446:T13)  [unwired: 2 in]
            n187 = call "Clear_Data_Main_v2.vi"("ZI Data 0"=w428, "ZI Data 3"=w446, "Time Of Collected Data (ms)"=500.0, 3:"Fixed Number Of Points"=w443, "error in"=w445, 10:"Fixed Number Of Points"=TRUE ("Fixed Number Of Points"), "Check Phase Mismatch"=FALSE) -> ("Cutted Data 0"=w442:T17, "Cutted Data 3"=w441:T17, "error out"=w444:errorcluster)  [unwired: 7 in, 3 out]
            n188 = call "Prepare_plots_SubVI_v1.vi"("Signal in X or Y (?)"="Signal in X or Y (?)", "Y rot avg in"=w439, "X rot avg in"=w440, "Cutted Data 3"=w441, "Cutted Data 0"=w442) -> ("Y rot avg out"=w438:dbl[], "X rot avg out"=w437:dbl[], "Monitor"=→"Intensity signal":cluster{"Time":dbl[], dbl[]}, "RF out"=→"Differential signal":cluster{"Time":dbl[], "Y":dbl[]}[], "Rotation spectrum"=→"Rotation spectrum":waveform(dbl)[], "Rotation"=w433:cluster{"Time":dbl[], dbl[]}[], "Polarimeter"=→"Polarimeter":dbl)
            n189 = Index Array(array=w433) -> (element #1=w432:cluster{"Time":dbl[], dbl[]}, element #2=w431:cluster{"Time":dbl[], dbl[]})  [unwired: 2 in]
            n190 = Select(t=w432, s="Signal in X or Y (?)", f=w431) -> (s? t:f=w426:cluster{"Time":dbl[], dbl[]})
            "Rotation signal" <- w426
          }
          n191 = call "Close_Devices_Main_v2.vi"("error in"=w396, "Resources"=w397) -> ("error out"=w376:errorcluster)  [unwired: 9 in]
          n192 = flat-sequence {
            tunnel: w376 -> [_]
            frame #0 {
              n193 = local write "Progress"(100.0 ("Progress")) -> ()
            }
          }
          n194 = Merge Errors(w376, w366) -> (w365:errorcluster)
          n195 = Divide(x=w374, y="Number of repetition") -> (x/y=w372:dbl[])
          n196 = Divide(x=w375, y="Number of repetition") -> (x/y=w373:dbl[])
          n197 = Unbundle By Name(w388) -> ("Time"=w379:dbl[])
          n198 = Release Queue(queue=w392, error in (no error)=w365) -> (error out=w364:errorcluster)  [unwired: 1 in, 2 out]
          n199 = Build Array(w372, w373) -> (w380:dbl[][])
          n200 = Bundle("Time"=w379, w372) -> (w385:cluster{"Time":dbl[], dbl[]})  [unwired: 1 in]
          n201 = Bundle("Time"=w379, w373) -> (w386:cluster{"Time":dbl[], dbl[]})  [unwired: 1 in]
          n202 = Index Array(array=w379, index #1=1 ("index"), index #2=0 ("index")) -> (element #1=w383:dbl, element #2=w384:dbl)
          n203 = Select(t=w385, s=w387, f=w386) -> (s? t:f=w362:cluster{"Time":dbl[], dbl[]})
          n204 = Subtract(x=w383, y=w384) -> (x-y=w378:dbl)
          n205 = local write "Rotation signal"(w362) -> ()
          n206 = local read "save"() -> (w363:bool)
          n207 = for {
            tunnel: w380 -> [w425] mode=indexing
            tunnel: [w423] -> w377 mode=indexing
            tunnel: w378 -> [w420]
            n208 = call <vilib>:"Auto Power Spectrum.vi"("dt"=w420, "Signal (V)"=w425) -> ("df"=w424:dbl, "Power Spectrum (V^2 rms)"=w422:dbl[])
            n209 = Square Root(x=w422) -> (sqrt(x)=w421:dbl[])
            n210 = Bundle By Name("Y"=w421, "dt"=w424) -> (w423:waveform(dbl))  [unwired: 1 in]
          }
          n211 = case shown="False" w363 {
            tunnel: w362 -> [_ w419]
            frame False {
            }
            frame True {
              n212 = Unbundle(w419) -> ("Time"=w418:dbl[], w417:dbl[])
              n213 = Build Array(w418, w417) -> (w416:dbl[][])
              n214 = call <vilib>:"Create File with Incrementing Suffix.vi"("format string (\" (%d)\")"=" %d" ("format string (\" (%d)\")"), "file path"=path "C:/Users/Daniel/Desktop/tests/test.dat") -> ("actual path"=w413:path)  [unwired: 7 in, 2 out]
              n215 = Transpose 2D Array(2D array=w416) -> (transposed array=w415:dbl[][])
              n216 = call-poly <vilib>:"Write Delimited Spreadsheet.vi"("file path (dialog if empty)"=w413, "format (%.3f)"="%.6f", "2D data"=w415) -> ()  [unwired: 11 in, 2 out]
            }
          }
          n217 = local write "Rotation spectrum"(w377) -> ()
        }
        n218 = case shown="Error .." w323 {
          selector: w323 -> [w471 w472]
          tunnel: [w471 w475] -> w324
          frame No Error {
          }
          frame Error {
            w480 = "\r\n"
            n219 = Unbundle By Name(w472) -> ("code"=w483:i32, "source"=w481:string)
            n220 = Number To Decimal String(number=w483) -> (decimal integer string=w482:string)  [unwired: 1 in]
            n221 = Concatenate Strings("There is an error:" ("string"), w480, w482, w480, w481, w480, "Do you want to clear it?" ("string")) -> (w476:string)
            n222 = Two Button Dialog(message=w476, 1:"No" ("F button name (\"Cancel\")"), 2:"Yes" ("T button name (\"OK\")")) -> (T button?=w474:bool)
            n223 = call <vilib>:"Clear Errors.vi"("error in (no error)"=w472) -> ("error out"=w473:errorcluster)  [unwired: 5 in, 1 out]
            n224 = Select(t=w473, s=w474, f=w472) -> (s? t:f=w475:errorcluster)
          }
        }
      }
      event "Run tomography", "Run tomography 2": Mouse Down {
        w509 = T13 {"R"=[], "Theta"=[], "X"=[], "Y"=[], "AuxIn0"=[], "AuxIn1"=[], "Frequency"=[], "DIO"=[], "Time"=[]} ("ZI Data")
        w504 = "\\tomography" ("string")
        n225 = event-data() -> ()  [unwired: 1 in, 8 out]
        n226 = local read "Config folder"() -> (w505:string)
        n227 = local read "Resource Address"() -> (w529:T3)
        n228 = Build Array(w509, w509) -> (w508:T13[])
        n229 = flat-sequence {
          frame #0 {
            n230 = Wait (ms)(milliseconds to wait=u32 150) -> ()  [unwired: 1 out]
          }
          frame #1 {
            n231 = invoke on="Run tomography" class="Bool (strict)" method="Reinit To Default"() -> ()  [unwired: 3 in, 3 out]
            n232 = local write "Tab Control"(T10."Run tomography" ("Tab Control")) -> ()
          }
        }
        n233 = Concatenate Strings("Config_files\\" ("string"), w505, w504) -> (w507:string)
        n234 = Concatenate Strings(w505, w504, "\\" ("string")) -> (w503:string)
        n235 = call <vilib>:"Application Directory.vi"() -> ("Application Directory"=w532:path)
        n236 = Obtain Queue(name (unnamed)="Data Queue 2", element data type=w508, error in (no error)=w526) -> (queue out=w528:refnum<queue>, error out=w525:errorcluster)  [unwired: 2 in, 1 out]
        n237 = property on="Plot type" class="Ring (strict)"("DisabledEnum"=T9."Disabled and Grayed Out" ("Disabled")) -> (error out=w514:errorcluster)  [unwired: 2 in, 1 out]
        n238 = Concatenate Strings(w505, "\\Zurich_params.ini" ("string")) -> (w535:string)
        n239 = Concatenate Strings(w505, "\\Keithley_params.ini" ("string")) -> (w536:string)
        n240 = Build Path(base path=w532, name or relative path=w507) -> (appended path=w533:path)
        n241 = List Folder(path=w533) -> (filenames=w531:string[])  [unwired: 3 in, 3 out]
        n242 = call "Initialize_Devices_Main_v2.vi"("error in"=w525, "Resource Address"=w529) -> ("error out"=w499:errorcluster, "Resources"=w500:T14)  [unwired: 8 in]
        n243 = call "GSF_GET.vi"("Resources in"=w500, "Config files paths"=T7 {"ZI config file (.ini)"="Config_Ver_2\\GSF_Zurich_params.ini", "Keithley config file (.ini)"="Config_Ver_2\\Keithley_params.ini", "DAQ config file (.ini)"="Config_Ver_2\\GSF_pulse_sequence_DAQ.ini"}, "error in"=w499) -> ("Resources out"=w498:T14, "Back Front GSF (Mean B,Mean F, SD B,SD F)"=w495:dbl[], "error out"=w497:errorcluster)  [unwired: 7 in, 3 out]
        n244 = for {
          tunnel: "pulses type (priv)" -> [w542] mode=indexing
          tunnel: [w540] -> w517 mode=concatenating
          n245 = for {
            tunnel: " + " ("string") -> [w547]
            tunnel: w542 -> [w546]
            tunnel: string[] ["[ None ]", "[ Y pi ]", "[ Z(pi/2)+Y(pi) ]"] -> [w545] mode=indexing
            tunnel: [w544] -> w540 mode=indexing
            n246 = Concatenate Strings(w546, w547, w545) -> (w544:string)
          }
        }
        n247 = for {
          N -> [w576]
          tunnel: w536 -> [w584]
          tunnel: w535 -> [w583]
          tunnel: w531 -> [w548] mode=indexing
          shift-right: [w579] -> w501
          shift-left: w497 -> [w554]
          tunnel: w528 -> [w580]
          shift-right: [w581] -> w524
          shift-left: w498 -> [w553]
          tunnel: u16 58000 ("Fixed Number Of Points") -> [w577]
          tunnel: [w578] -> w522
          shift-right: [w572] -> w519
          shift-left: dbl[][] [] -> [w573]
          tunnel: w517 -> [_]
          tunnel: [w569] -> w516 mode=indexing
          tunnel: w514 -> [_]
          tunnel: w503 -> [w550]
          i -> [w570]
          n248 = Concatenate Strings(w550, w548) -> (w549:string)
          n249 = Multiply(x="Averaging", y=w570) -> (x*y=w575:i32)
          n250 = Bundle By Name(cluster=T7 {"ZI config file (.ini)"="Config_Ver_2\\Zurich_params.ini", "Keithley config file (.ini)"="Config_Ver_2\\Keithley_params.ini", "DAQ config file (.ini)"="Config_Ver_2\\pulse_sequence_DAQ.ini"} ("Config files paths"), "ZI config file (.ini)"=w583, "Keithley config file (.ini)"=w584, "DAQ config file (.ini)"=w549) -> (w551:T7)
          n251 = call "Configurate_All_Main_v2.vi"("Resources in"=w553, "Config files paths"=w551, "error in"=w554) -> ("Resources out"=w552:T14, "error out"=w555:errorcluster)  [unwired: 6 in, 5 out]
          n252 = for {
            N: "Averaging" -> [w633]
            shift-right: [w645] -> w581
            shift-left: w552 -> [w647]
            shift-right: [w636] -> w567
            shift-left: w555 -> [w646]
            tunnel: w580 -> [w638]
            tunnel: w551 -> [w635]
            tunnel: w576 -> [w634]
            tunnel: w575 -> [w630]
            i -> [w631]
            n253 = Add(x=w631, y=w630) -> (x+y=w629:i32)
            n254 = Multiply(x=w633, y=w634) -> (x*y=w632:i32)
            n255 = call "Single_Measurement_Main_v2.vi"("Config files paths"=w635, "error in"=w646, "Resources in"=w647) -> ("error out"=w643:errorcluster, "Resources out"=w644:T14)  [unwired: 6 in, 1 out]
            n256 = call "Poll_Data_Main_v2.vi"("error in"=w643, "Resources in"=w644) -> ("error out"=w637:errorcluster, "ZI Data 3"=w640:T13, "ZI Data 0"=w627:T13, "Resources out"=w645:T14)  [unwired: 6 in]
            n257 = Divide(x=w629, y=w632) -> (x/y=w641:dbl)
            n258 = Build Array(w627, w640) -> (w639:T13[])
            n259 = Multiply(x=w641, y=100.0) -> (x*y=→"Progress":dbl)
            n260 = Enqueue Element(queue=w638, element=w639, error in (no error)=w637) -> (error out=w636:errorcluster)  [unwired: 1 in, 2 out]
          }
          n261 = Initialize Array(0.0 ("element"), w577) -> (w564:dbl[])
          n262 = for {
            N: "Averaging" -> [_]
            shift-right: [w618] -> w568
            shift-left: w554 -> [w623]
            shift-right: [w612] -> w562
            shift-left: w564 -> [w615]
            shift-right: [w613] -> w563
            shift-left: w564 -> [w614]
            tunnel: [w605] -> w558
            tunnel: w580 -> [w604]
            tunnel: w577 -> [w603]
            tunnel: [w602] -> w560
            n263 = local read "Signal in X or Y (?)"() -> (w605:bool)
            n264 = Dequeue Element(queue=w604, timeout in ms (-1)=10000, error in (no error)=w623) -> (element=w622:T13[], error out=w619:errorcluster)  [unwired: 2 out]
            n265 = Index Array(array=w622) -> (element #1=w620:T13, element #2=w621:T13)  [unwired: 2 in]
            n266 = call "Clear_Data_Main_v2.vi"("ZI Data 0"=w620, "ZI Data 3"=w621, "Time Of Collected Data (ms)"=500.0, 3:"Fixed Number Of Points"=w603, "error in"=w619, 10:"Fixed Number Of Points"=TRUE ("Fixed Number Of Points"), "Check Phase Mismatch"=FALSE) -> ("Cutted Data 0"=w617:T17, "Cutted Data 3"=w616:T17, "error out"=w618:errorcluster)  [unwired: 7 in, 3 out]
            n267 = call "Prepare_plots_SubVI_v1.vi"("Signal in X or Y (?)"=w605, "Y rot avg in"=w614, "X rot avg in"=w615, "Cutted Data 3"=w616, "Cutted Data 0"=w617) -> ("Y rot avg out"=w613:dbl[], "X rot avg out"=w612:dbl[], "Monitor"=→"Intensity signal":cluster{"Time":dbl[], dbl[]}, "RF out"=→"Differential signal":cluster{"Time":dbl[], "Y":dbl[]}[], "Rotation spectrum"=→"Rotation spectrum":waveform(dbl)[], "Rotation"=w609:cluster{"Time":dbl[], dbl[]}[])  [unwired: 1 out]
            n268 = Index Array(array=w609) -> (element #1=w608:cluster{"Time":dbl[], dbl[]}, element #2=w607:cluster{"Time":dbl[], dbl[]})  [unwired: 2 in]
            n269 = Select(t=w608, s=w605, f=w607) -> (s? t:f=w602:cluster{"Time":dbl[], dbl[]})
            "Rotation signal" <- w602
          }
          n270 = Divide(x=w562, y="Averaging") -> (x/y=w556:dbl[])
          n271 = Divide(x=w563, y="Averaging") -> (x/y=w557:dbl[])
          n272 = Empty Array?(array=w573) -> (empty?=w561:bool)
          n273 = Unbundle By Name(w560) -> ("Time"=w559:dbl[])
          n274 = Merge Errors(w567, w568) -> (w566:errorcluster)
          n275 = case shown="True" w561 {
            tunnel: w559 -> [w586 w593]
            tunnel: w573 -> [w592 w600]
            tunnel: [w591 w599] -> w572
            tunnel: w558 -> [w590 w598]
            tunnel: w557 -> [w589 w597]
            tunnel: w556 -> [w588 w596]
            tunnel: [w585 w595] -> w571
            frame True {
              n276 = Select(t=w588, s=w590, f=w589) -> (s? t:f=w587:dbl[])
              n277 = Bundle("Time"=w586, w587) -> (w585:cluster{"Time":dbl[], dbl[]})  [unwired: 1 in]
              n278 = Build Array (concatenate)(w592, w586, w587) -> (w591:dbl[][])
            }
            frame False {
              n279 = Select(t=w596, s=w598, f=w597) -> (s? t:f=w594:dbl[])
              n280 = Bundle("Time"=w593, w594) -> (w595:cluster{"Time":dbl[], dbl[]})  [unwired: 1 in]
              n281 = Build Array (concatenate)(w600, w594) -> (w599:dbl[][])
            }
          }
          n282 = Flush Queue(queue=w580, error in (no error)=w566) -> (queue out=w578:refnum<queue>, error out=w579:errorcluster)  [unwired: 1 out]
          n283 = flat-sequence {
            tunnel: w571 -> [w648]
            tunnel: w570 -> [w649]
            tunnel: [w648] -> w569
            frame #0 {
              n284 = local write "Plot type"(w649) -> ()
              "Rotation" <- w648
            }
          }
        }
        "tomography rotation memory (priv)" <- w516
        n285 = property on="Plot type" class="Ring (strict)"("Strings []"=w517) -> ()  [unwired: 2 in, 2 out]
        n286 = Release Queue(queue=w522, error in (no error)=w501) -> (error out=w521:errorcluster)  [unwired: 1 in, 2 out]
        n287 = flat-sequence {
          tunnel: w501 -> [_]
          frame #0 {
            n288 = local write "Progress"(100.0 ("Progress")) -> ()
          }
        }
        n289 = call "Close_Devices_Main_v2.vi"("error in"=w521, "Resources"=w524) -> ("error out"=w512:errorcluster)  [unwired: 9 in]
        n290 = property on="Plot type" class="Ring (strict)"(error in=w501, "DisabledEnum"=T9."Enabled" ("Disabled")) -> (error out=w511:errorcluster)  [unwired: 1 in, 1 out]
        n291 = Or(x="Save raw data (?)", y="Save CYCLOPS data (?)") -> (x .or. y?=w489:bool)
        n292 = Build Array(w495) -> (w494:dbl[][])
        n293 = call "Save_Tomography_Data_Main_v2.vi"("error in"=w501, "Save CYCLOPS data (?)"="Save CYCLOPS data (?)", "Save raw data (?)"="Save raw data (?)", "Data Raw"=w519) -> ("error out"=w493:errorcluster)  [unwired: 6 in, 1 out]
        n294 = call "Save_GSF_Data.vi"("error in"=w493, "Save"=w489, "GSF_Data"=w494) -> ("error out"=w492:errorcluster)  [unwired: 8 in]
        n295 = Merge Errors(w512, w511, w492) -> (w510:errorcluster)
        n296 = case shown="Error .." w510 {
          selector: w510 -> [w650 w651]
          tunnel: [w650 w654] -> w534
          frame No Error {
          }
          frame Error {
            w659 = "\r\n"
            n297 = Unbundle By Name(w651) -> ("code"=w662:i32, "source"=w660:string)
            n298 = Number To Decimal String(number=w662) -> (decimal integer string=w661:string)  [unwired: 1 in]
            n299 = Concatenate Strings("There is an error:" ("string"), w659, w661, w659, w660, w659, "Do you want to clear it?" ("string")) -> (w655:string)
            n300 = Two Button Dialog(message=w655, 1:"No" ("F button name (\"Cancel\")"), 2:"Yes" ("T button name (\"OK\")")) -> (T button?=w653:bool)
            n301 = call <vilib>:"Clear Errors.vi"("error in (no error)"=w651) -> ("error out"=w652:errorcluster)  [unwired: 5 in, 1 out]
            n302 = Select(t=w652, s=w653, f=w651) -> (s? t:f=w654:errorcluster)
          }
        }
      }
      event "Run QPT", "Run QPT 2": Mouse Down {
        w686 = "\\process\\temp_states" ("string")
        # "9 FIDs compose 1 Tomography"
        n303 = event-data() -> ()  [unwired: 1 in, 8 out]
        n304 = local read "Config folder"() -> (w687:string)
        n305 = local read "Resource Address"() -> (w679:T3)
        n306 = flat-sequence {
          frame #0 {
            n307 = Wait (ms)(milliseconds to wait=u32 150) -> ()  [unwired: 1 out]
          }
          frame #1 {
            n308 = invoke on="Run tomography" class="Bool (strict)" method="Reinit To Default"() -> ()  [unwired: 3 in, 3 out]
            n309 = local write "Tab Control"(T1."Run QPT" ("Tab Control")) -> ()
          }
        }
        n310 = Concatenate Strings("Config_files\\" ("string"), w687, w686) -> (w689:string)
        n311 = Concatenate Strings(w687, w686, "\\" ("string")) -> (w685:string)
        n312 = call <vilib>:"Application Directory.vi"() -> ("Application Directory"=w694:path)
        n313 = property on="Plot type" class="Ring (strict)"("DisabledEnum"=T9."Disabled and Grayed Out" ("Disabled")) -> (error out=w683:errorcluster)  [unwired: 2 in, 1 out]
        n314 = Concatenate Strings(w687, "\\Zurich_params.ini" ("string")) -> (w697:string)
        n315 = Concatenate Strings(w687, "\\Keithley_params.ini" ("string")) -> (w698:string)
        n316 = Build Path(base path=w694, name or relative path=w689) -> (appended path=w695:path)
        n317 = List Folder(path=w695) -> (filenames=w682:string[])  [unwired: 3 in, 3 out]
        n318 = call "Splitting_filename.vi"("Splitting number"=u32 9, "Total filenames"=w682) -> ("Splitted filenames"=w681:string[][])  [unwired: 9 in]
        n319 = for {
          N: 2 -> [w731]
          tunnel: w698 -> [w742]
          tunnel: w697 -> [w741]
          tunnel: w685 -> [w738]
          tunnel: w681 -> [w737] mode=indexing
          shift-right: [w739] -> w691
          shift-left: _ -> [_]
          shift-right: [w716] -> w690
          shift-left: w683 -> [w736]
          tunnel: w679 -> [w727]
          tunnel: w678 -> [w726]
          tunnel: [w721] -> w677
          shift-right: [w707] -> w674
          shift-left: dbl[][] [] -> [w709]
          tunnel: [w706] -> w671
          tunnel: [w705] -> w670
          tunnel: "Save raw data  2" -> [w706]
          tunnel: "Save CYCLOPS data 2" -> [w705]
          i -> [w719]
          w702 = T13 {"R"=[], "Theta"=[], "X"=[], "Y"=[], "AuxIn0"=[], "AuxIn1"=[], "Frequency"=[], "DIO"=[], "Time"=[]} ("ZI Data")
          n320 = Increment(x=w719) -> (x+1=→"Current_QPT_order":i32)
          n321 = Build Array(w702, w702) -> (w703:T13[])
          n322 = Divide(x=w719, y=w731) -> (x/y=w730:dbl)
          n323 = Obtain Queue(name (unnamed)="Data Queue 2", element data type=w703, error in (no error)=w726) -> (queue out=w725:refnum<queue>, error out=w724:errorcluster)  [unwired: 2 in, 1 out]
          n324 = Multiply(x=100.0, y=w730) -> (x*y=→"QPT Progress":dbl)
          n325 = call "Initialize_Devices_Main_v2.vi"("error in"=w724, "Resource Address"=w727) -> ("error out"=w713:errorcluster, "Resources"=w714:T14)  [unwired: 8 in]
          n326 = call "GSF_GET.vi"("Resources in"=w714, "Config files paths"=T7 {"ZI config file (.ini)"="Config_Ver_2\\GSF_Zurich_params.ini", "Keithley config file (.ini)"="Config_Ver_2\\Keithley_params.ini", "DAQ config file (.ini)"="Config_Ver_2\\GSF_pulse_sequence_DAQ.ini"}, "error in"=w713) -> ("Resources out"=w712:T14, "Back Front GSF (Mean B,Mean F, SD B,SD F)"=w708:dbl[], "error out"=w711:errorcluster)  [unwired: 7 in, 3 out]
          n327 = for {
            N -> [w773]
            tunnel: w742 -> [w780]
            tunnel: w741 -> [w779]
            tunnel: w737 -> [w745] mode=indexing
            shift-right: [w776] -> w717
            shift-left: w711 -> [w751]
            shift-right: [w777] -> w722
            shift-left: w712 -> [w750]
            tunnel: u16 58000 ("Fixed Number Of Points") -> [w774]
            tunnel: [w775] -> w735
            shift-right: [w769] -> w718
            shift-left: dbl[][] [] -> [w770]
            tunnel: [w766] -> w732 mode=indexing
            tunnel: w738 -> [w747]
            tunnel: w736 -> [_]
            tunnel: w725 -> [w744]
            i -> [w767]
            n328 = Concatenate Strings(w747, w745) -> (w746:string)
            n329 = Multiply(x="Averaging 2", y=w767) -> (x*y=w772:i32)
            n330 = Bundle By Name(cluster=T7 {"ZI config file (.ini)"="Config_Ver_2\\Zurich_params.ini", "Keithley config file (.ini)"="Config_Ver_2\\Keithley_params.ini", "DAQ config file (.ini)"="Config_Ver_2\\pulse_sequence_DAQ.ini"} ("Config files paths"), "ZI config file (.ini)"=w779, "Keithley config file (.ini)"=w780, "DAQ config file (.ini)"=w746) -> (w748:T7)
            n331 = call "Configurate_All_Main_v2.vi"("Resources in"=w750, "Config files paths"=w748, "error in"=w751) -> ("Resources out"=w749:T14, "error out"=w752:errorcluster)  [unwired: 6 in, 5 out]
            n332 = for {
              N: "Averaging 2" -> [w829]
              shift-right: [w841] -> w777
              shift-left: w749 -> [w843]
              shift-right: [w832] -> w764
              shift-left: w752 -> [w842]
              tunnel: w744 -> [w834]
              tunnel: w748 -> [w831]
              tunnel: w773 -> [w830]
              tunnel: w772 -> [w826]
              i -> [w827]
              n333 = Add(x=w827, y=w826) -> (x+y=w825:i32)
              n334 = Multiply(x=w829, y=w830) -> (x*y=w828:i32)
              n335 = call "Single_Measurement_Main_v2.vi"("Config files paths"=w831, "error in"=w842, "Resources in"=w843) -> ("error out"=w839:errorcluster, "Resources out"=w840:T14)  [unwired: 6 in, 1 out]
              n336 = call "Poll_Data_Main_v2.vi"("error in"=w839, "Resources in"=w840) -> ("error out"=w833:errorcluster, "ZI Data 3"=w836:T13, "ZI Data 0"=w823:T13, "Resources out"=w841:T14)  [unwired: 6 in]
              n337 = Divide(x=w825, y=w828) -> (x/y=w837:dbl)
              n338 = Build Array(w823, w836) -> (w835:T13[])
              n339 = Multiply(x=w837, y=100.0) -> (x*y=→"Single Tomography Progress":dbl)
              n340 = Enqueue Element(queue=w834, element=w835, error in (no error)=w833) -> (error out=w832:errorcluster)  [unwired: 1 in, 2 out]
            }
            n341 = Initialize Array(0.0 ("element"), w774) -> (w761:dbl[])
            n342 = for {
              N: "Averaging 2" -> [_]
              shift-right: [w814] -> w765
              shift-left: w751 -> [w819]
              shift-right: [w808] -> w759
              shift-left: w761 -> [w811]
              shift-right: [w809] -> w760
              shift-left: w761 -> [w810]
              tunnel: [w801] -> w755
              tunnel: w744 -> [w800]
              tunnel: w774 -> [w799]
              tunnel: [w798] -> w757
              n343 = local read "Signal in X or Y (?)"() -> (w801:bool)
              n344 = Dequeue Element(queue=w800, timeout in ms (-1)=10000, error in (no error)=w819) -> (element=w818:T13[], error out=w815:errorcluster)  [unwired: 2 out]
              n345 = Index Array(array=w818) -> (element #1=w816:T13, element #2=w817:T13)  [unwired: 2 in]
              n346 = call "Clear_Data_Main_v2.vi"("ZI Data 0"=w816, "ZI Data 3"=w817, "Time Of Collected Data (ms)"=500.0, 3:"Fixed Number Of Points"=w799, "error in"=w815, 10:"Fixed Number Of Points"=TRUE ("Fixed Number Of Points"), "Check Phase Mismatch"=FALSE) -> ("Cutted Data 0"=w813:T17, "Cutted Data 3"=w812:T17, "error out"=w814:errorcluster)  [unwired: 7 in, 3 out]
              n347 = call "Prepare_plots_SubVI_v1.vi"("Signal in X or Y (?)"=w801, "Y rot avg in"=w810, "X rot avg in"=w811, "Cutted Data 3"=w812, "Cutted Data 0"=w813) -> ("Y rot avg out"=w809:dbl[], "X rot avg out"=w808:dbl[], "Monitor"=→"Intensity signal 2":cluster{"Time":dbl[], dbl[]}, "RF out"=→"Differential signal 2":cluster{"Time":dbl[], "Y":dbl[]}[], "Rotation spectrum"=→"Rotation spectrum 2":waveform(dbl)[], "Rotation"=w805:cluster{"Time":dbl[], dbl[]}[])  [unwired: 1 out]
              n348 = Index Array(array=w805) -> (element #1=w804:cluster{"Time":dbl[], dbl[]}, element #2=w803:cluster{"Time":dbl[], dbl[]})  [unwired: 2 in]
              n349 = Select(t=w804, s=w801, f=w803) -> (s? t:f=w798:cluster{"Time":dbl[], dbl[]})
              "Rotation signal 2" <- w798
            }
            n350 = Divide(x=w759, y="Averaging 2") -> (x/y=w753:dbl[])
            n351 = Divide(x=w760, y="Averaging 2") -> (x/y=w754:dbl[])
            n352 = Empty Array?(array=w770) -> (empty?=w758:bool)
            n353 = Unbundle By Name(w757) -> ("Time"=w756:dbl[])
            n354 = Merge Errors(w764, w765) -> (w763:errorcluster)
            n355 = case shown="False" w758 {
              tunnel: w756 -> [w782 w789]
              tunnel: w770 -> [w788 w796]
              tunnel: [w787 w795] -> w769
              tunnel: w755 -> [w786 w794]
              tunnel: w754 -> [w785 w793]
              tunnel: w753 -> [w784 w792]
              tunnel: [w781 w791] -> w768
              frame True {
                n356 = Select(t=w784, s=w786, f=w785) -> (s? t:f=w783:dbl[])
                n357 = Bundle("Time"=w782, w783) -> (w781:cluster{"Time":dbl[], dbl[]})  [unwired: 1 in]
                n358 = Build Array (concatenate)(w788, w782, w783) -> (w787:dbl[][])
              }
              frame False {
                n359 = Select(t=w792, s=w794, f=w793) -> (s? t:f=w790:dbl[])
                n360 = Bundle("Time"=w789, w790) -> (w791:cluster{"Time":dbl[], dbl[]})  [unwired: 1 in]
                n361 = Build Array (concatenate)(w796, w790) -> (w795:dbl[][])
              }
            }
            n362 = Flush Queue(queue=w744, error in (no error)=w763) -> (queue out=w775:refnum<queue>, error out=w776:errorcluster)  [unwired: 1 out]
            n363 = flat-sequence {
              tunnel: w768 -> [w844]
              tunnel: w767 -> [w845]
              tunnel: [w844] -> w766
              frame #0 {
                n364 = local write "Plot type"(w845) -> ()
                "Rotation 2" <- w844
              }
            }
          }
          "tomography rotation memory (priv) 2" <- w732
          n365 = Build Array (concatenate)(w709, w708) -> (w707:dbl[][])
          n366 = local read "Current_QPT_order"() -> (w715:i32)
          n367 = Release Queue(queue=w735, error in (no error)=w717) -> (error out=w723:errorcluster)  [unwired: 1 in, 2 out]
          n368 = flat-sequence {
            tunnel: w717 -> [_]
            frame #0 {
              n369 = local write "Single Tomography Progress"(100.0 ("Progress")) -> ()
            }
          }
          n370 = property on="Plot type" class="Ring (strict)"(error in=w717, "DisabledEnum"=T9."Enabled" ("Disabled")) -> (error out=w739:errorcluster)  [unwired: 1 in, 1 out]
          n371 = call "Save_QPT_Data_Main_v2.vi"("Numeric"=w715, "error in"=w717, "Save CYCLOPS data (?)"=w705, "Save raw data (?)"=w706, "Data Raw"=w718) -> ("error out"=w716:errorcluster)  [unwired: 5 in, 1 out]
          n372 = call "Close_Devices_Main_v2.vi"("error in"=w723, "Resources"=w722) -> ("error out"=w721:errorcluster)  [unwired: 9 in]
        }
        "appended array" <- w674
        n373 = flat-sequence {
          tunnel: w677 -> [_]
          frame #0 {
            n374 = local write "QPT Progress"(100.0 ("x")) -> ()
          }
        }
        n375 = Merge Errors(w677, w691, w690) -> (w673:errorcluster)
        n376 = Or(x=w671, y=w670) -> (x .or. y?=w669:bool)
        n377 = call "Save_GSF_Data.vi"("error in"=w673, "time format string (%c)"="Data\\QPT\\%d_%B_%y\\%H_%M_%S_", "Save"=w669, "GSF_Data"=w674) -> ("error out"=w672:errorcluster)  [unwired: 7 in]
        n378 = case shown="Error .." w672 {
          selector: w672 -> [w846 w847]
          tunnel: [w846 w850] -> w696
          frame No Error {
          }
          frame Error {
            w855 = "\r\n"
            n379 = Unbundle By Name(w847) -> ("code"=w858:i32, "source"=w856:string)
            n380 = Number To Decimal String(number=w858) -> (decimal integer string=w857:string)  [unwired: 1 in]
            n381 = Concatenate Strings("There is an error:" ("string"), w855, w857, w855, w856, w855, "Do you want to clear it?" ("string")) -> (w851:string)
            n382 = Two Button Dialog(message=w851, 1:"No" ("F button name (\"Cancel\")"), 2:"Yes" ("T button name (\"OK\")")) -> (T button?=w849:bool)
            n383 = call <vilib>:"Clear Errors.vi"("error in (no error)"=w847) -> ("error out"=w848:errorcluster)  [unwired: 5 in, 1 out]
            n384 = Select(t=w848, s=w849, f=w847) -> (s? t:f=w850:errorcluster)
          }
        }
      }
      event "Plot type": Value Change {
        n385 = event-data() -> ()  [unwired: 1 in, 6 out]
        n386 = local read "tomography rotation memory (priv)"() -> (w864:cluster{"Time":dbl[], dbl[]}[])
        n387 = local read "Plot type"() -> (w865:u16)
        n388 = Index Array(array=w864, index=w865) -> (element=w866:cluster{"Time":dbl[], dbl[]})
        n389 = local write "Rotation"(w866) -> ()
      }
      event "Fit model": Mouse Down {
        w872 = 2.0 ("x")
        w890 = 5 ("y")
        w897 = 1 ("index")
        # "q"
        # "w"
        # "g"
        # "C"
        # "B"
        # "A"
        # "initial values:"
        n390 = event-data() -> ()  [unwired: 1 in, 8 out]
        n391 = local read "Rotation signal"() -> (w891:cluster{"Time":dbl[], dbl[]})
        n392 = Decrement(x=w897) -> (x-1=w899:i32)
        n393 = Unbundle(w891) -> ("Time"=w898:dbl[], w895:dbl[])
        n394 = property on="Rotation signal" class="XYGraph (strict)"(error in=w905, "Visible"=FALSE) -> (error out=w903:errorcluster)  [unwired: 1 in, 1 out]
        n395 = property on="Rotation signal 3" class="XYGraph (strict)"(error in=w905, "Visible"=TRUE) -> (error out=w904:errorcluster)  [unwired: 1 in, 1 out]
        n396 = local read "Polarimeter"() -> (w880:dbl)
        n397 = Array Size(array=w895) -> (size(s)=w896:i32)
        n398 = Index Array(array=w898, index #1=w897, index #2=w899) -> (element #1=w900:dbl, element #2=w901:dbl)
        n399 = Multiply(x=1100.0, y=6.283185307179586) -> (x*y=w876:dbl)
        n400 = Subtract(x=w900, y=w901) -> (x-y=w889:dbl)
        n401 = Quotient & Remainder(x=w896, y=w890) -> (floor(x/y)=w894:i32)  [unwired: 1 out]
        n402 = Merge Errors(w903, w904) -> (w902:errorcluster)
        n403 = Reshape Array(w895, w894, w890) -> (w893:dbl[][])
        n404 = Multiply(x=w889, y=w890) -> (x*y=w887:dbl)
        n405 = Index Array(array=w893, index (col)=0 ("disabled index (col)")) -> (element=w869:dbl[])  [unwired: 1 in]
        n406 = Array Subset(array=w869, index=0, length=100) -> (w883:dbl[])
        n407 = Array Max & Min(array=w883) -> (max value=w882:dbl, min value=w881:dbl)  [unwired: 2 out]
        n408 = Subtract(x=w882, y=w881) -> (x-y=w873:dbl)
        n409 = Add(x=w882, y=w881) -> (x+y=w874:dbl)
        n410 = Divide(x=w874, y=w872) -> (x/y=w871:dbl)
        n411 = Divide(x=w873, y=w872) -> (x/y=w870:dbl)
        n412 = Array Size(array=w869) -> (size(s)=w888:i32)
        n413 = for {
          N: w888 -> [_]
          tunnel: w887 -> [w913]
          tunnel: [w912] -> w886 mode=indexing
          i -> [w914]
          n414 = Multiply(x=w913, y=w914) -> (x*y=w912:dbl)
        }
        n415 = Multiply(x=w869, y=1000) -> (x*y=w867:dbl[])
        n416 = case shown="\"Full\"" "Enum" {
          tunnel: [w946 w972 w999] -> w908
          tunnel: [w935 w962 w991] -> w906
          tunnel: w902 -> [w935 w962 w991]
          tunnel: w891 -> [w945 w971 w998]
          tunnel: w886 -> [w938 w965 w994]
          tunnel: w871 -> [w944 _ w977]
          tunnel: w880 -> [w943 w970 w976]
          tunnel: 20.0 -> [w942 w969 w975]
          tunnel: w876 -> [_ w956 w974]
          tunnel: 0.0 -> [_ w957 w973]
          tunnel: w870 -> [_ w958 w978]
          tunnel: w867 -> [w939 w966 w995]
          frame "B*Exp(-q2*t)+C" {
            w947 = nan
            n417 = Build Array(w944, w943, w942) -> (w936:dbl[])
            n418 = call-poly <vilib>:"Nonlinear Curve Fit.vi"("Y"=w939, "initial parameters"=w936, "X"=w938, "model description"=T11 {"model"="b*exp(-g2*t)+c", "Parameters"=["b", "c", "g2"], "x"="t"}, "error in (no error)"=w935) -> ("best nonlinear fit"=w937:dbl[], "best fit parameters"=w933:dbl[])  [unwired: 6 in, 3 out]
            n419 = Divide(x=w937, y=1000) -> (x/y=w941:dbl[])
            n420 = Index Array(array=w933) -> (element #1=w932:dbl, element #2=w931:dbl, element #3=w930:dbl)  [unwired: 3 in]
            n421 = Bundle(w938, w941) -> (w929:cluster{dbl[], dbl[]})  [unwired: 1 in]
            n422 = Build Array(w945, w929) -> (w946:cluster{"Time":dbl[], dbl[]}[])
            n423 = local write "A"(w947) -> ()
            n424 = local write "C"(w931) -> ()
            n425 = local write "g2"(w930) -> ()
            n426 = local write "q"(w947) -> ()
            n427 = local write "w"(w947) -> ()
            n428 = local write "g1"(w947) -> ()
            n429 = local write "B"(w932) -> ()
          }
          frame "A*Sin(w*t+q)*Exp(-g1*t)+C" {
            w955 = nan
            n430 = Build Array(w958, w970, w969, w957, w956) -> (w963:dbl[])
            n431 = call-poly <vilib>:"Nonlinear Curve Fit.vi"("Y"=w966, "initial parameters"=w963, "X"=w965, "model description"=T11 {"model"="a*sin(w*t+q)*exp(-g1*t)+c", "Parameters"=["a", "c", "g1", "q", "w"], "x"="t"}, "error in (no error)"=w962) -> ("best nonlinear fit"=w964:dbl[], "best fit parameters"=w960:dbl[])  [unwired: 6 in, 3 out]
            n432 = Divide(x=w964, y=1000) -> (x/y=w968:dbl[])
            n433 = Index Array(array=w960) -> (element #1=w954:dbl, element #2=w953:dbl, element #3=w952:dbl, element #4=w950:dbl, element #5=w951:dbl)  [unwired: 5 in]
            n434 = Bundle(w965, w968) -> (w959:cluster{dbl[], dbl[]})  [unwired: 1 in]
            n435 = Quotient & Remainder(x=w950, y=6.283185307179586) -> (x-y*floor(x/y)=w948:dbl)  [unwired: 1 out]
            n436 = Build Array(w971, w959) -> (w972:cluster{"Time":dbl[], dbl[]}[])
            n437 = local write "g1"(w952) -> ()
            n438 = local write "w"(w951) -> ()
            n439 = local write "A"(w954) -> ()
            n440 = local write "C"(w953) -> ()
            n441 = local write "q"(w948) -> ()
            n442 = local write "B"(w955) -> ()
            n443 = local write "g2"(w955) -> ()
          }
          frame "Full" {
            n444 = Build Array(w978, w977, w976, w975, w975, w974, w973) -> (w992:dbl[])
            n445 = call-poly <vilib>:"Nonlinear Curve Fit.vi"("Y"=w995, "initial parameters"=w992, "X"=w994, "model description"=T11 {"model"="a*sin(w*t+q)*exp(-g1*t)+b*exp(-g2*t)+c", "Parameters"=["a", "b", "c", "g1", "g2", "w", "q"], "x"="t"}, "error in (no error)"=w991) -> ("best nonlinear fit"=w993:dbl[], "best fit parameters"=w982:dbl[])  [unwired: 6 in, 3 out]
            n446 = Divide(x=w993, y=1000) -> (x/y=w997:dbl[])
            n447 = Index Array(array=w982) -> (element #1=w988:dbl, element #2=w984:dbl, element #3=w985:dbl, element #4=w986:dbl, element #5=w987:dbl, element #6=w983:dbl, element #7=w979:dbl)  [unwired: 7 in]
            n448 = Bundle(w994, w997) -> (w989:cluster{dbl[], dbl[]})  [unwired: 1 in]
            n449 = local write "w"(w983) -> ()
            n450 = local write "A"(w988) -> ()
            n451 = local write "B"(w984) -> ()
            n452 = local write "C"(w985) -> ()
            n453 = local write "g1"(w986) -> ()
            n454 = local write "g2"(w987) -> ()
            n455 = Quotient & Remainder(x=w979, y=6.283185307179586) -> (x-y*floor(x/y)=w980:dbl)  [unwired: 1 out]
            n456 = Build Array(w998, w989) -> (w999:cluster{"Time":dbl[], dbl[]}[])
            n457 = local write "q"(w980) -> ()
          }
        }
        n458 = Reverse 1D Array(array=w908) -> (reversed array=→"Rotation signal 3":cluster{"Time":dbl[], dbl[]}[])
        n459 = case shown="Error .." w906 {
          selector: w906 -> [w915 w916]
          tunnel: [w915 w919] -> _
          frame No Error {
          }
          frame Error {
            w924 = "\r\n"
            n460 = Unbundle By Name(w916) -> ("code"=w927:i32, "source"=w925:string)
            n461 = Number To Decimal String(number=w927) -> (decimal integer string=w926:string)  [unwired: 1 in]
            n462 = Concatenate Strings("There is an error:" ("string"), w924, w926, w924, w925, w924, "Do you want to clear it?" ("string")) -> (w920:string)
            n463 = Two Button Dialog(message=w920, 1:"No" ("F button name (\"Cancel\")"), 2:"Yes" ("T button name (\"OK\")")) -> (T button?=w918:bool)
            n464 = call <vilib>:"Clear Errors.vi"("error in (no error)"=w916) -> ("error out"=w917:errorcluster)  [unwired: 5 in, 1 out]
            n465 = Select(t=w917, s=w918, f=w916) -> (s? t:f=w919:errorcluster)
          }
        }
      }
      event "AOC": Mouse Down {
        n466 = event-data() -> ()  [unwired: 1 in, 8 out]
        n467 = Look In Map(map=w1009, key="pulse Y") -> (value=w1024:i32)  [unwired: 1 in, 1 out]
        n468 = Look In Map(map=w1007, key="Y pi/2") -> (value=w1022:dbl)  [unwired: 1 in, 1 out]
        n469 = Look In Map(map=w1007, key="Delay") -> (value=w1021:dbl)  [unwired: 1 in, 1 out]
        n470 = Look In Map(map=w1009, key="pulse Z") -> (value=w1018:i32)  [unwired: 1 in, 1 out]
        n471 = Look In Map(map=w1007, key="Z pi/4") -> (value=w1015:dbl)  [unwired: 1 in, 1 out]
        n472 = Look In Map(map=w1007, key="Delay") -> (value=w1016:dbl)  [unwired: 1 in, 1 out]
        n473 = call "Add_to_sequence_SubVI_v1.vi"("Delay [us]"=w1021, "Pulse length [us]"=w1022, "Channel number"=w1024, "Array sequence in"=w1025) -> ("Array sequence out"=w1020:cluster{"Timing 0":dbl[]}[])
        n474 = call "Add_to_sequence_SubVI_v1.vi"("Delay [us]"=w1016, "Pulse length [us]"=w1015, "Channel number"=w1018, "Array sequence in"=w1020) -> ("Array sequence out"=w1010:cluster{"Timing 0":dbl[]}[])
        n475 = Wait (ms)(milliseconds to wait=u32 150) -> ()  [unwired: 1 out]
        n476 = Look In Map(map=w1009, key="pulse Y") -> (value=w1005:i32)  [unwired: 1 in, 1 out]
        n477 = Look In Map(map=w1007, key="Y pi/2") -> (value=w1004:dbl)  [unwired: 1 in, 1 out]
        n478 = Look In Map(map=w1007, key="Delay") -> (value=w1003:dbl)  [unwired: 1 in, 1 out]
        n479 = call "Add_to_sequence_SubVI_v1.vi"("Delay [us]"=w1003, "Pulse length [us]"=w1004, "Channel number"=w1005, "Array sequence in"=w1010) -> ("Array sequence out"=w1002:cluster{"Timing 0":dbl[]}[])
      }
      event "X pi": Mouse Down {
        n480 = event-data() -> ()  [unwired: 1 in, 8 out]
        n481 = Look In Map(map=w1031, key="X pi") -> (value=w1027:dbl)  [unwired: 1 in, 1 out]
        n482 = Look In Map(map=w1031, key="Delay") -> (value=w1026:dbl)  [unwired: 1 in, 1 out]
        n483 = Look In Map(map=w1037, key="pulse X") -> (value=w1028:i32)  [unwired: 1 in, 1 out]
        n484 = Wait (ms)(milliseconds to wait=u32 150) -> ()  [unwired: 1 out]
        n485 = call "Add_to_sequence_SubVI_v1.vi"("Delay [us]"=w1026, "Pulse length [us]"=w1027, "Channel number"=w1028, "Array sequence in"=w1030) -> ("Array sequence out"=w1029:cluster{"Timing 0":dbl[]}[])
      }
      event "X pi/2": Mouse Down {
        n486 = event-data() -> ()  [unwired: 1 in, 8 out]
        n487 = Look In Map(map=w1043, key="X pi/2") -> (value=w1039:dbl)  [unwired: 1 in, 1 out]
        n488 = Look In Map(map=w1043, key="Delay") -> (value=w1038:dbl)  [unwired: 1 in, 1 out]
        n489 = Look In Map(map=w1049, key="pulse X") -> (value=w1040:i32)  [unwired: 1 in, 1 out]
        n490 = Wait (ms)(milliseconds to wait=u32 150) -> ()  [unwired: 1 out]
        n491 = call "Add_to_sequence_SubVI_v1.vi"("Delay [us]"=w1038, "Pulse length [us]"=w1039, "Channel number"=w1040, "Array sequence in"=w1042) -> ("Array sequence out"=w1041:cluster{"Timing 0":dbl[]}[])
      }
      event "X pi/4": Mouse Down {
        n492 = event-data() -> ()  [unwired: 1 in, 8 out]
        n493 = Look In Map(map=w1060, key="pulse X") -> (value=w1056:i32)  [unwired: 1 in, 1 out]
        n494 = Look In Map(map=w1058, key="X pi/4") -> (value=w1055:dbl)  [unwired: 1 in, 1 out]
        n495 = Look In Map(map=w1058, key="Delay") -> (value=w1054:dbl)  [unwired: 1 in, 1 out]
        n496 = Wait (ms)(milliseconds to wait=u32 150) -> ()  [unwired: 1 out]
        n497 = call "Add_to_sequence_SubVI_v1.vi"("Delay [us]"=w1054, "Pulse length [us]"=w1055, "Channel number"=w1056, "Array sequence in"=w1053) -> ("Array sequence out"=w1052:cluster{"Timing 0":dbl[]}[])
      }
      event "Y pi": Mouse Down {
        n498 = event-data() -> ()  [unwired: 1 in, 8 out]
        n499 = Look In Map(map=w1066, key="Y pi") -> (value=w1062:dbl)  [unwired: 1 in, 1 out]
        n500 = Look In Map(map=w1066, key="Delay") -> (value=w1061:dbl)  [unwired: 1 in, 1 out]
        n501 = Look In Map(map=w1072, key="pulse Y") -> (value=w1063:i32)  [unwired: 1 in, 1 out]
        n502 = Wait (ms)(milliseconds to wait=u32 150) -> ()  [unwired: 1 out]
        n503 = call "Add_to_sequence_SubVI_v1.vi"("Delay [us]"=w1061, "Pulse length [us]"=w1062, "Channel number"=w1063, "Array sequence in"=w1065) -> ("Array sequence out"=w1064:cluster{"Timing 0":dbl[]}[])
      }
      event "Y pi/2": Mouse Down {
        n504 = event-data() -> ()  [unwired: 1 in, 8 out]
        n505 = Look In Map(map=w1078, key="Y pi/2") -> (value=w1074:dbl)  [unwired: 1 in, 1 out]
        n506 = Look In Map(map=w1078, key="Delay") -> (value=w1073:dbl)  [unwired: 1 in, 1 out]
        n507 = Look In Map(map=w1084, key="pulse Y") -> (value=w1075:i32)  [unwired: 1 in, 1 out]
        n508 = Wait (ms)(milliseconds to wait=u32 150) -> ()  [unwired: 1 out]
        n509 = call "Add_to_sequence_SubVI_v1.vi"("Delay [us]"=w1073, "Pulse length [us]"=w1074, "Channel number"=w1075, "Array sequence in"=w1077) -> ("Array sequence out"=w1076:cluster{"Timing 0":dbl[]}[])
      }
      event "Y pi/4": Mouse Down {
        n510 = event-data() -> ()  [unwired: 1 in, 8 out]
        n511 = Look In Map(map=w1090, key="Y pi/4") -> (value=w1086:dbl)  [unwired: 1 in, 1 out]
        n512 = Look In Map(map=w1090, key="Delay") -> (value=w1085:dbl)  [unwired: 1 in, 1 out]
        n513 = Look In Map(map=w1096, key="pulse Y") -> (value=w1087:i32)  [unwired: 1 in, 1 out]
        n514 = Wait (ms)(milliseconds to wait=u32 150) -> ()  [unwired: 1 out]
        n515 = call "Add_to_sequence_SubVI_v1.vi"("Delay [us]"=w1085, "Pulse length [us]"=w1086, "Channel number"=w1087, "Array sequence in"=w1089) -> ("Array sequence out"=w1088:cluster{"Timing 0":dbl[]}[])
      }
      event "Z pi": Mouse Down {
        n516 = event-data() -> ()  [unwired: 1 in, 8 out]
        n517 = Look In Map(map=w1102, key="Z pi") -> (value=w1098:dbl)  [unwired: 1 in, 1 out]
        n518 = Look In Map(map=w1102, key="Delay") -> (value=w1097:dbl)  [unwired: 1 in, 1 out]
        n519 = Look In Map(map=w1108, key="pulse Z") -> (value=w1099:i32)  [unwired: 1 in, 1 out]
        n520 = Wait (ms)(milliseconds to wait=u32 150) -> ()  [unwired: 1 out]
        n521 = call "Add_to_sequence_SubVI_v1.vi"("Delay [us]"=w1097, "Pulse length [us]"=w1098, "Channel number"=w1099, "Array sequence in"=w1101) -> ("Array sequence out"=w1100:cluster{"Timing 0":dbl[]}[])
      }
      event "Z pi/2": Mouse Down {
        n522 = event-data() -> ()  [unwired: 1 in, 8 out]
        n523 = Look In Map(map=w1114, key="Z pi/2") -> (value=w1110:dbl)  [unwired: 1 in, 1 out]
        n524 = Look In Map(map=w1114, key="Delay") -> (value=w1109:dbl)  [unwired: 1 in, 1 out]
        n525 = Look In Map(map=w1120, key="pulse Z") -> (value=w1111:i32)  [unwired: 1 in, 1 out]
        n526 = Wait (ms)(milliseconds to wait=u32 150) -> ()  [unwired: 1 out]
        n527 = call "Add_to_sequence_SubVI_v1.vi"("Delay [us]"=w1109, "Pulse length [us]"=w1110, "Channel number"=w1111, "Array sequence in"=w1113) -> ("Array sequence out"=w1112:cluster{"Timing 0":dbl[]}[])
      }
      event "Z pi/4": Mouse Down {
        n528 = event-data() -> ()  [unwired: 1 in, 8 out]
        n529 = Look In Map(map=w1126, key="Z pi/4") -> (value=w1122:dbl)  [unwired: 1 in, 1 out]
        n530 = Look In Map(map=w1126, key="Delay") -> (value=w1121:dbl)  [unwired: 1 in, 1 out]
        n531 = Look In Map(map=w1132, key="pulse Z") -> (value=w1123:i32)  [unwired: 1 in, 1 out]
        n532 = Wait (ms)(milliseconds to wait=u32 150) -> ()  [unwired: 1 out]
        n533 = call "Add_to_sequence_SubVI_v1.vi"("Delay [us]"=w1121, "Pulse length [us]"=w1122, "Channel number"=w1123, "Array sequence in"=w1125) -> ("Array sequence out"=w1124:cluster{"Timing 0":dbl[]}[])
      }
      event "Add pulse": Mouse Down {
        # "If it is nonlinear coil, it should be waited for much more time.\nBecause the pulse shape of the nonlinear coil is not good. It still affects the atom  after the pulse pauses"
        # "The nonlinear coil value"
        n534 = event-data() -> ()  [unwired: 1 in, 8 out]
        n535 = local read "Channel"() -> (w1133:u16)
        n536 = property on="Channel" class="Ring (strict)"() -> ("Value"=w1135:u16)  [unwired: 2 in, 2 out]
        n537 = Equal?(x=w1135, y=u16 9) -> (x = y?=w1137:bool)
        n538 = Index Array(array=w1138, index=w1133) -> (element=w1146:string)
        n539 = Look In Map(map=w1147, key=w1146) -> (value=w1136:i32)  [unwired: 1 in, 1 out]
        n540 = case shown="True" w1137 {
          tunnel: w1143 -> [w1149 w1155]
          tunnel: [w1148 w1152] -> w1140
          frame False {
            n541 = Look In Map(map=w1149, key="Delay") -> (value=w1148:dbl)  [unwired: 1 in, 1 out]
          }
          frame True {
            n542 = Look In Map(map=w1155, key="Delay") -> (value=w1153:dbl)  [unwired: 1 in, 1 out]
            n543 = Add(x=50.0, y=w1153) -> (x+y=w1152:dbl)
          }
        }
        n544 = Wait (ms)(milliseconds to wait=u32 150) -> ()  [unwired: 1 out]
        n545 = call "Add_to_sequence_SubVI_v1.vi"("Delay [us]"=w1140, "Pulse length [us]"="Time [us]", "Channel number"=w1136, "Array sequence in"=w1142) -> ("Array sequence out"=w1141:cluster{"Timing 0":dbl[]}[])
      }
      event "Add pulse advanced": Mouse Down {
        # "Search for choosen channels"
        n546 = event-data() -> ()  [unwired: 1 in, 8 out]
        n547 = for {
          tunnel: "Physical channels" -> [w1175] mode=indexing
          tunnel: w1168 -> [w1176]
          tunnel: [w1174] -> w1167 mode=indexing
          tunnel: [w1172] -> w1164 mode=indexing
          n548 = Search 1D Array(1D array=w1176, element=w1175) -> (index of element=w1174:i32)  [unwired: 1 in]
          n549 = Equal?(x=w1174, y=-1) -> (x = y?=w1172:bool)
        }
        n550 = Or Array Elements(Boolean array=w1164) -> (logical OR=w1163:bool)
        n551 = case shown="True" w1163 {
          frame False {
          }
          frame True {
            n552 = One Button Dialog(message="Some port names are not correct!!!\nPulse sequance may not be correct!") -> ()  [unwired: 1 in, 1 out]
          }
        }
        n553 = for {
          tunnel: w1170 -> [w1178] mode=indexing
          tunnel: w1167 -> [w1182]
          tunnel: [w1177] -> w1160 mode=indexing
          i -> [w1181]
          n554 = for {
            tunnel: w1182 -> [w1198] mode=indexing
            tunnel: w1181 -> [w1199]
            tunnel: [w1197] -> w1180 mode=indexing
            n555 = Equal?(x=w1198, y=w1199) -> (x = y?=w1197:bool)
          }
          n556 = Or Array Elements(Boolean array=w1180) -> (logical OR=w1179:bool)
          n557 = case shown="True" w1179 {
            tunnel: w1178 -> [w1185 w1192]
            tunnel: [w1183 w1190] -> w1177
            frame True {
              n558 = local read "Time [us]"() -> (w1184:dbl)
              n559 = in-place {
                in-place-border: w1184 -> [w1188]
                n560 = in-place-cluster #9(w1185) -> ("Timing 0"=w1189:dbl[])
                n561 = Build Array (concatenate)(w1189, w1188, 0.0 ("element")) -> (w1186:dbl[])
                n562 = in-place-cluster #9("Timing 0"=w1186) -> (w1183:cluster{"Timing 0":dbl[]})
              }
            }
            frame False {
              n563 = local read "Time [us]"() -> (w1191:dbl)
              n564 = in-place {
                in-place-border: w1191 -> [w1194]
                n565 = in-place-cluster #10(w1192) -> ("Timing 0"=w1196:dbl[])
                n566 = Build Array (concatenate)(w1196, 0.0 ("element"), w1194) -> (w1195:dbl[])
                n567 = in-place-cluster #10("Timing 0"=w1195) -> (w1190:cluster{"Timing 0":dbl[]})
              }
            }
          }
        }
        n568 = Look In Map(map=w1162, key="Delay") -> (value=w1156:dbl)  [unwired: 1 in, 1 out]
        n569 = Wait (ms)(milliseconds to wait=u32 150) -> ()  [unwired: 1 out]
        n570 = call "Add_to_sequence_SubVI_v1.vi"("Delay [us]"=w1156, "Pulse length [us]"=0.0, "Channel number"=-1, "Array sequence in"=w1160) -> ("Array sequence out"=w1159:cluster{"Timing 0":dbl[]}[])
      }
      event "Save single sequence": Mouse Down {
        n571 = event-data() -> ()  [unwired: 1 in, 8 out]
        n572 = Look In Map(map=w1222, key="Accqusition TRIG") -> (value=w1212:i32)  [unwired: 1 in, 1 out]
        n573 = Look In Map(map=w1219, key="TTL") -> (value=w1211:dbl)  [unwired: 1 in, 1 out]
        n574 = Look In Map(map=w1219, key="Delay") -> (value=w1210:dbl)  [unwired: 1 in, 1 out]
        n575 = Look In Map(map=w1219, key="Probe") -> (value=w1214:dbl)  [unwired: 1 in, 1 out]
        n576 = for {
          tunnel: w1209 -> [w1231] mode=indexing
          tunnel: w1211 -> [w1230]
          tunnel: [w1229] -> w1213 mode=indexing
          tunnel: w1212 -> [w1228]
          i -> [w1227]
          n577 = Equal?(x=w1228, y=w1227) -> (x = y?=w1232:bool)
          n578 = case shown="True" w1232 {
            tunnel: w1231 -> [w1233 w1236]
            tunnel: w1230 -> [_ w1235]
            tunnel: [w1233 w1234] -> w1229
            frame False {
            }
            frame True {
              n579 = in-place {
                in-place-border: w1235 -> [w1237]
                n580 = in-place-cluster #11(w1236) -> ("Timing 0"=w1238:dbl[])
                n581 = Build Array (concatenate)(w1238, w1237) -> (w1239:dbl[])
                n582 = in-place-cluster #11("Timing 0"=w1239) -> (w1234:cluster{"Timing 0":dbl[]})
              }
            }
          }
        }
        n583 = Look In Map(map=w1222, key="Keithley TRIG") -> (value=w1217:i32)  [unwired: 1 in, 1 out]
        n584 = for {
          tunnel: w1213 -> [w1260] mode=indexing
          tunnel: w1217 -> [w1262]
          tunnel: w1211 -> [w1259]
          tunnel: w1210 -> [w1258]
          tunnel: [w1257] -> w1215 mode=indexing
          i -> [w1263]
          n585 = Equal?(x=w1263, y=w1262) -> (x = y?=w1261:bool)
          n586 = case shown="True" w1261 {
            tunnel: w1260 -> [w1264 w1268]
            tunnel: w1259 -> [_ w1267]
            tunnel: w1258 -> [_ w1266]
            tunnel: [w1264 w1265] -> w1257
            frame False {
            }
            frame True {
              n587 = in-place {
                in-place-border: w1267 -> [w1272]
                in-place-border: w1266 -> [w1271]
                n588 = in-place-cluster #12(w1268) -> ("Timing 0"=w1274:dbl[])
                n589 = Multiply(x=2.0, y=w1271) -> (x*y=w1269:dbl)
                n590 = Build Array (concatenate)(w1274, 0.0, w1269, w1272) -> (w1275:dbl[])
                n591 = in-place-cluster #12("Timing 0"=w1275) -> (w1265:cluster{"Timing 0":dbl[]})
              }
            }
          }
        }
        n592 = Look In Map(map=w1222, key="LD probe") -> (value=w1216:i32)  [unwired: 1 in, 1 out]
        n593 = flat-sequence {
          frame #0 {
            n594 = Wait (ms)(milliseconds to wait=u32 150) -> ()  [unwired: 1 out]
          }
          frame #1 {
            n595 = invoke on="Save single sequence" class="Bool (strict)" method="Reinit To Default"() -> ()  [unwired: 3 in, 3 out]
          }
        }
        n596 = for {
          tunnel: w1216 -> [w1245]
          tunnel: w1215 -> [w1243] mode=indexing
          tunnel: w1214 -> [w1242]
          tunnel: [w1241] -> w1208 mode=indexing
          tunnel: w1210 -> [w1240]
          i -> [w1246]
          n597 = Equal?(x=w1246, y=w1245) -> (x = y?=w1244:bool)
          n598 = case shown="True" w1244 {
            tunnel: w1243 -> [w1247 w1251]
            tunnel: [w1247 w1250] -> w1241
            tunnel: w1242 -> [_ w1249]
            tunnel: w1240 -> [_ w1248]
            frame False {
            }
            frame True {
              n599 = in-place {
                in-place-border: w1249 -> [w1252]
                in-place-border: w1248 -> [w1253]
                n600 = in-place-cluster #13(w1251) -> ("Timing 0"=w1255:dbl[])
                n601 = Build Array (concatenate)(w1255, 0.0, w1253, w1252) -> (w1256:dbl[])
                n602 = in-place-cluster #13("Timing 0"=w1256) -> (w1250:cluster{"Timing 0":dbl[]})
              }
            }
          }
        }
        n603 = call "Array_to_cluster_sequence_SubVI_v1.vi"("Array"=w1208) -> ("Sequence"=w1207:T6)
        n604 = local read "Sampling data"() -> (w1205:T2)
        n605 = local read "Config folder"() -> (w1202:string)
        n606 = Concatenate Strings(w1202, "\\pulse_sequence_DAQ.ini" ("string")) -> (w1200:string)
        n607 = call "Set_Pulse_Seq_DAQ.vi"("Time Unit"=T12 {"Time Unit"=enum."MicroSecond"}, "error in"=w1204, "Sampling data"=w1205, "Sequence"=w1207, "Filename (ini)"=w1200) -> ("error out"=w1203:errorcluster)  [unwired: 6 in]
      }
      event "Save multi Sequence": Mouse Down {
        n608 = event-data() -> ()  [unwired: 1 in, 8 out]
        n609 = local read "Config folder"() -> (w1279:string)
        n610 = call <vilib>:"Application Directory.vi"() -> ("Application Directory"=w1288:path)
        n611 = Concatenate Strings(w1279, "\\temp_multi_FID\\" ("string")) -> (w1278:string)
        n612 = Concatenate Strings("Config_Files\\" ("string"), w1278) -> (w1285:string)
        n613 = String To Path(string=w1285) -> (path=w1287:path)
        n614 = Build Path(base path=w1288, name or relative path=w1287) -> (appended path=w1286:path)
        n615 = call <userlib>:"List Directory__ogtk.vi"("directory path"=w1286) -> ("file names"=w1284:string[])  [unwired: 3 in, 3 out]
        n616 = for {
          tunnel: w1284 -> [w1294] mode=indexing
          shift-right: [w1295] -> w1283
          shift-left: w1282 -> [w1296]
          tunnel: w1278 -> [w1293]
          n617 = Concatenate Strings(w1293, w1294) -> (w1297:string)
          n618 = call "Delete_file.vi"("error in"=w1296, "Filename (ini)"=w1297) -> ("error out"=w1295:errorcluster)  [unwired: 9 in]
        }
        n619 = local read "Period number"() -> (w1277:u32)
        n620 = local read "Period [us]"() -> (w1276:dbl)
        n621 = for {
          N: w1277 -> [_]
          tunnel: w1292 -> [w1305]
          tunnel: w1291 -> [w1302]
          tunnel: w1290 -> [w1311]
          tunnel: w1276 -> [w1327]
          tunnel: w1283 -> [w1319]
          tunnel: [w1317] -> w1289
          i -> [w1313]
          # "Write the full number in the name to store the data\n 1-->001\n10-->010\n100-->100"
          n622 = Multiply(x=w1327, y=w1313) -> (x*y=w1309:dbl)
          n623 = Look In Map(map=w1302, key="Delay") -> (value=w1308:dbl)  [unwired: 1 in, 1 out]
          n624 = Look In Map(map=w1305, key="Nonlinear coil") -> (value=w1310:i32)  [unwired: 1 in, 1 out]
          n625 = Look In Map(map=w1302, key="Delay") -> (value=w1299:dbl)  [unwired: 1 in, 1 out]
          n626 = Look In Map(map=w1302, key="Probe") -> (value=w1331:dbl)  [unwired: 1 in, 1 out]
          n627 = Look In Map(map=w1302, key="TTL") -> (value=w1328:dbl)  [unwired: 1 in, 1 out]
          n628 = Look In Map(map=w1305, key="pulse X") -> (value=w1303:i32)  [unwired: 1 in, 1 out]
          n629 = call "Add_to_sequence_SubVI_Directly.vi"("Delay [us]"=w1308, "Pulse length [us]"=w1309, "Channel number"=w1310, "Array sequence in"=w1311) -> ("Array sequence out"=w1307:cluster{"Timing 0":dbl[]}[])
          n630 = Look In Map(map=w1302, key="X pi/4") -> (value=w1300:dbl)  [unwired: 1 in, 1 out]
          n631 = call "Add_to_sequence_SubVI_v1.vi"("Delay [us]"=w1299, "Pulse length [us]"=w1300, "Channel number"=w1303, "Array sequence in"=w1307) -> ("Array sequence out"=w1306:cluster{"Timing 0":dbl[]}[])
          n632 = Look In Map(map=w1305, key="Accqusition TRIG") -> (value=w1329:i32)  [unwired: 1 in, 1 out]
          n633 = for {
            tunnel: w1306 -> [w1361] mode=indexing
            tunnel: w1328 -> [w1360]
            tunnel: [w1359] -> w1330 mode=indexing
            tunnel: w1329 -> [w1358]
            i -> [w1357]
            n634 = Equal?(x=w1358, y=w1357) -> (x = y?=w1362:bool)
            n635 = case shown="True" w1362 {
              tunnel: w1361 -> [w1363 w1366]
              tunnel: w1360 -> [_ w1365]
              tunnel: [w1363 w1364] -> w1359
              frame False {
              }
              frame True {
                n636 = in-place {
                  in-place-border: w1365 -> [w1367]
                  n637 = in-place-cluster #14(w1366) -> ("Timing 0"=w1368:dbl[])
                  n638 = Build Array (concatenate)(w1368, w1367) -> (w1369:dbl[])
                  n639 = in-place-cluster #14("Timing 0"=w1369) -> (w1364:cluster{"Timing 0":dbl[]})
                }
              }
            }
          }
          n640 = Look In Map(map=w1305, key="LD probe") -> (value=w1333:i32)  [unwired: 1 in, 1 out]
          n641 = Look In Map(map=w1305, key="Keithley TRIG") -> (value=w1334:i32)  [unwired: 1 in, 1 out]
          n642 = for {
            tunnel: w1330 -> [w1390] mode=indexing
            tunnel: w1334 -> [w1392]
            tunnel: w1328 -> [w1389]
            tunnel: w1299 -> [w1388]
            tunnel: [w1387] -> w1332 mode=indexing
            i -> [w1393]
            n643 = Equal?(x=w1393, y=w1392) -> (x = y?=w1391:bool)
            n644 = case shown="True" w1391 {
              tunnel: w1390 -> [w1394 w1398]
              tunnel: w1389 -> [_ w1397]
              tunnel: w1388 -> [_ w1396]
              tunnel: [w1394 w1395] -> w1387
              frame False {
              }
              frame True {
                n645 = in-place {
                  in-place-border: w1397 -> [w1402]
                  in-place-border: w1396 -> [w1401]
                  n646 = in-place-cluster #15(w1398) -> ("Timing 0"=w1404:dbl[])
                  n647 = Multiply(x=2.0, y=w1401) -> (x*y=w1399:dbl)
                  n648 = Build Array (concatenate)(w1404, 0.0, w1399, w1402) -> (w1405:dbl[])
                  n649 = in-place-cluster #15("Timing 0"=w1405) -> (w1395:cluster{"Timing 0":dbl[]})
                }
              }
            }
          }
          n650 = for {
            tunnel: w1333 -> [w1375]
            tunnel: w1332 -> [w1373] mode=indexing
            tunnel: w1331 -> [w1372]
            tunnel: [w1371] -> w1325 mode=indexing
            tunnel: w1299 -> [w1370]
            i -> [w1376]
            n651 = Equal?(x=w1376, y=w1375) -> (x = y?=w1374:bool)
            n652 = case shown="True" w1374 {
              tunnel: w1373 -> [w1377 w1381]
              tunnel: [w1377 w1380] -> w1371
              tunnel: w1372 -> [_ w1379]
              tunnel: w1370 -> [_ w1378]
              frame False {
              }
              frame True {
                n653 = in-place {
                  in-place-border: w1379 -> [w1382]
                  in-place-border: w1378 -> [w1383]
                  n654 = in-place-cluster #16(w1381) -> ("Timing 0"=w1385:dbl[])
                  n655 = Build Array (concatenate)(w1385, 0.0, w1383, w1382) -> (w1386:dbl[])
                  n656 = in-place-cluster #16("Timing 0"=w1386) -> (w1380:cluster{"Timing 0":dbl[]})
                }
              }
            }
          }
          n657 = Less?(x=w1313, y=10) -> (x < y?=w1314:bool)
          n658 = case shown="False" w1314 {
            tunnel: [w1341 w1352] -> w1312
            tunnel: w1313 -> [w1342 w1355]
            frame False {
              n659 = Less?(x=w1342, y=100) -> (x < y?=w1343:bool)
              n660 = case shown="False" w1343 {
                tunnel: w1342 -> [w1346 w1350]
                tunnel: [w1345 w1347] -> w1341
                frame False {
                  (unwired) i16 1 ("width (-)")
                  n661 = Number To Decimal String(number=w1346) -> (decimal integer string=w1345:string)  [unwired: 1 in]
                }
                frame True {
                  n662 = Number To Decimal String(number=w1350, width (-)=i16 1) -> (decimal integer string=w1349:string)
                  n663 = Concatenate Strings("0" ("string"), w1349) -> (w1347:string)
                }
              }
            }
            frame True {
              n664 = Number To Decimal String(number=w1355, width (-)=i16 1) -> (decimal integer string=w1354:string)
              n665 = Concatenate Strings("00" ("string"), w1354) -> (w1352:string)
            }
          }
          n666 = call "Array_to_cluster_sequence_SubVI_v1.vi"("Array"=w1325) -> ("Sequence"=w1318:T6)
          n667 = local read "Sampling data"() -> (w1322:T2)
          n668 = local read "Config folder"() -> (w1323:string)
          n669 = Concatenate Strings(w1323, "\\temp_multi_FID\\Single_FID_" ("string"), w1312, ".ini" ("string")) -> (w1324:string)
          n670 = call "Set_Pulse_Seq_DAQ.vi"("Time Unit"=T12 {"Time Unit"=enum."MicroSecond"}, "error in"=w1319, "Sampling data"=w1322, "Sequence"=w1318, "Filename (ini)"=w1324) -> ("error out"=w1317:errorcluster)  [unwired: 6 in]
        }
        n671 = flat-sequence {
          frame #0 {
            n672 = Wait (ms)(milliseconds to wait=u32 150) -> ()  [unwired: 1 out]
          }
          frame #1 {
            n673 = invoke on="Save single sequence" class="Bool (strict)" method="Reinit To Default"() -> ()  [unwired: 3 in, 3 out]
          }
        }
      }
      event "Save multi-process": Mouse Down {
        # "Clear All processes files"
        n674 = event-data() -> ()  [unwired: 1 in, 8 out]
        n675 = local read "Config folder"() -> (w1410:string)
        n676 = call <vilib>:"Application Directory.vi"() -> ("Application Directory"=w1419:path)
        n677 = Concatenate Strings(w1410, "\\process\\processes_sets\\" ("string")) -> (w1409:string)
        n678 = Concatenate Strings("Config_Files\\" ("string"), w1409) -> (w1416:string)
        n679 = String To Path(string=w1416) -> (path=w1418:path)
        n680 = Build Path(base path=w1419, name or relative path=w1418) -> (appended path=w1417:path)
        n681 = call <userlib>:"List Directory__ogtk.vi"("directory path"=w1417) -> ("file names"=w1415:string[])  [unwired: 3 in, 3 out]
        n682 = for {
          tunnel: w1415 -> [w1425] mode=indexing
          shift-right: [w1426] -> w1414
          shift-left: w1413 -> [w1427]
          tunnel: w1409 -> [w1424]
          n683 = Concatenate Strings(w1424, w1425) -> (w1428:string)
          n684 = call "Delete_file.vi"("error in"=w1427, "Filename (ini)"=w1428) -> ("error out"=w1426:errorcluster)  [unwired: 9 in]
        }
        n685 = local read "Period number"() -> (w1408:u32)
        n686 = local read "Period [us]"() -> (w1407:dbl)
        n687 = for {
          N: w1408 -> [_]
          tunnel: w1423 -> [w1434]
          tunnel: w1422 -> [w1433]
          tunnel: w1421 -> [w1438]
          tunnel: w1407 -> [w1453]
          tunnel: w1414 -> [w1446]
          tunnel: [w1444] -> w1420
          i -> [w1440]
          # "Write the full number in the name to store the data\n 1-->001\n10-->010\n100-->100"
          n688 = property on="Channel" class="Ring (strict)"() -> ("Strings []"=w1429:string[])  [unwired: 2 in, 2 out]
          n689 = property on="Channel" class="Ring (strict)"() -> ("Value"=w1430:u16)  [unwired: 2 in, 2 out]
          n690 = Index Array(array=w1429, index=w1430) -> (element=w1431:string)
          n691 = Multiply(x=w1453, y=w1440) -> (x*y=w1436:dbl)
          n692 = Look In Map(map=w1434, key=w1431) -> (value=w1437:i32)  [unwired: 1 in, 1 out]
          n693 = Look In Map(map=w1433, key="Delay") -> (value=w1435:dbl)  [unwired: 1 in, 1 out]
          n694 = call "Add_to_sequence_SubVI_Directly.vi"("Delay [us]"=w1435, "Pulse length [us]"=w1436, "Channel number"=w1437, "Array sequence in"=w1438) -> ("Array sequence out"=w1432:cluster{"Timing 0":dbl[]}[])
          n695 = Less?(x=w1440, y=10) -> (x < y?=w1441:bool)
          n696 = case shown="False" w1441 {
            tunnel: [w1454 w1465] -> w1439
            tunnel: w1440 -> [w1455 w1468]
            frame False {
              n697 = Less?(x=w1455, y=100) -> (x < y?=w1456:bool)
              n698 = case shown="False" w1456 {
                tunnel: w1455 -> [w1459 w1463]
                tunnel: [w1458 w1460] -> w1454
                frame False {
                  (unwired) i16 1 ("width (-)")
                  n699 = Number To Decimal String(number=w1459) -> (decimal integer string=w1458:string)  [unwired: 1 in]
                }
                frame True {
                  n700 = Number To Decimal String(number=w1463, width (-)=i16 1) -> (decimal integer string=w1462:string)
                  n701 = Concatenate Strings("0" ("string"), w1462) -> (w1460:string)
                }
              }
            }
            frame True {
              n702 = Number To Decimal String(number=w1468, width (-)=i16 1) -> (decimal integer string=w1467:string)
              n703 = Concatenate Strings("00" ("string"), w1467) -> (w1465:string)
            }
          }
          n704 = call "Array_to_cluster_sequence_SubVI_v1.vi"("Array"=w1432) -> ("Sequence"=w1445:T6)
          n705 = local read "Sampling data"() -> (w1449:T2)
          n706 = local read "Config folder"() -> (w1450:string)
          n707 = Concatenate Strings(w1450, "\\process\\processes_sets\\Processes_" ("string"), w1439, ".ini" ("string")) -> (w1451:string)
          n708 = call "Set_Pulse_Seq_DAQ.vi"("Time Unit"=T12 {"Time Unit"=enum."MicroSecond"}, "error in"=w1446, "Sampling data"=w1449, "Sequence"=w1445, "Filename (ini)"=w1451) -> ("error out"=w1444:errorcluster)  [unwired: 6 in]
        }
        n709 = flat-sequence {
          frame #0 {
            n710 = Wait (ms)(milliseconds to wait=u32 150) -> ()  [unwired: 1 out]
          }
          frame #1 {
            n711 = invoke on="Save single sequence" class="Bool (strict)" method="Reinit To Default"() -> ()  [unwired: 3 in, 3 out]
          }
        }
      }
      event "Save for tomography": Mouse Down {
        w1477 = string[][] [["None", "None"], ["Y pi", "None"], ["Z pi/2", "Y pi"]]
        w1471 = string[] ["None", "Y pi/2", "X pi/2"]
        # "Additional delay to ensure that\nall measurement start at the\nsame moment"
        # "CYCLOPS"
        # "Control pulses"
        n712 = event-data() -> ()  [unwired: 1 in, 8 out]
        n713 = local write "pulses type (priv)"(w1471) -> ()
        n714 = for {
          tunnel: w1479 -> [w1607]
          tunnel: w1471 -> [w1606] mode=indexing
          tunnel: [w1605] -> w1486 mode=indexing
          # "Check longest control pulse"
          n715 = Look In Map(map=w1607, key=w1606) -> (value=w1605:dbl)  [unwired: 1 in, 1 out]
        }
        n716 = Look In Map(map=w1479, key="Delay") -> (value=w1484:dbl)  [unwired: 1 in, 1 out]
        n717 = for {
          tunnel: w1479 -> [w1613]
          tunnel: w1477 -> [w1612] mode=indexing
          tunnel: w1484 -> [w1609]
          tunnel: [w1608] -> w1485 mode=indexing
          # "Check longest CYCLOPS sequence"
          n718 = for {
            tunnel: w1613 -> [w1616]
            tunnel: [w1615] -> w1611 mode=indexing
            tunnel: w1612 -> [w1614] mode=indexing
            n719 = Look In Map(map=w1616, key=w1614) -> (value=w1615:dbl)  [unwired: 1 in, 1 out]
          }
          n720 = Add Array Elements(numeric array=w1611) -> (sum=w1610:dbl)
          n721 = Add(x=w1610, y=w1609) -> (x+y=w1608:dbl)
        }
        n722 = for {
          tunnel: w1486 -> [w1603] mode=indexing
          tunnel: w1485 -> [w1604]
          tunnel: w1484 -> [w1601]
          tunnel: [w1602] -> w1482 mode=indexing
          n723 = Compound Arithmetic op=unknown(w1604, w1601, w1603, w1601) -> (w1602:dbl[])
        }
        n724 = Array Max & Min(array=w1482) -> (max value=w1483:dbl)  [unwired: 3 out]
        n725 = Subtract(x=w1483, y=w1482) -> (x-y=w1476:dbl[][])
        n726 = for {
          tunnel: string[] ["None", "pulse Y", "pulse X"] -> [w1513] mode=indexing
          tunnel: w1471 -> [w1514] mode=indexing
          tunnel: w1475 -> [w1515]
          tunnel: w1480 -> [w1504]
          tunnel: w1479 -> [w1505]
          tunnel: string[][] [["None", "None"], ["pulse Y", "None"], ["pulse Z", "pulse Y"]] -> [w1508]
          tunnel: w1477 -> [w1507]
          tunnel: [w1503] -> w1474 mode=concatenating
          tunnel: w1476 -> [w1502] mode=indexing
          # "Iterate over control pulses"
          n727 = Look In Map(map=w1504, key=w1513) -> (value=w1511:i32)  [unwired: 1 in, 1 out]
          n728 = Look In Map(map=w1505, key=w1514) -> (value=w1510:dbl)  [unwired: 1 in, 1 out]
          n729 = Look In Map(map=w1505, key="Delay") -> (value=w1506:dbl)  [unwired: 1 in, 1 out]
          n730 = call "Add_to_sequence_SubVI_v1.vi"("Delay [us]"=w1506, "Pulse length [us]"=w1510, "Channel number"=w1511, "Array sequence in"=w1515) -> ("Array sequence out"=w1509:cluster{"Timing 0":dbl[]}[])
          n731 = for {
            tunnel: w1509 -> [w1542]
            tunnel: w1508 -> [w1539] mode=indexing
            tunnel: w1507 -> [w1540] mode=indexing
            tunnel: w1506 -> [w1541]
            tunnel: w1505 -> [w1524]
            tunnel: w1504 -> [w1520]
            tunnel: [w1523] -> w1503 mode=indexing
            tunnel: w1502 -> [w1518] mode=indexing
            # "Add equalization of the time interval"
            # "Iterate over CYCLOPS in 2 for loops because CYCLOPS consists of a few pulses"
            n732 = for {
              shift-right: [w1593] -> w1522
              shift-left: w1542 -> [w1596]
              tunnel: w1541 -> [w1592]
              tunnel: w1540 -> [w1599] mode=indexing
              tunnel: w1539 -> [w1600] mode=indexing
              tunnel: w1524 -> [w1598]
              tunnel: w1520 -> [w1597]
              tunnel: [w1592] -> w1517
              n733 = Look In Map(map=w1597, key=w1600) -> (value=w1595:i32)  [unwired: 1 in, 1 out]
              n734 = Look In Map(map=w1598, key=w1599) -> (value=w1594:dbl)  [unwired: 1 in, 1 out]
              n735 = call "Add_to_sequence_SubVI_v1.vi"("Delay [us]"=w1592, "Pulse length [us]"=w1594, "Channel number"=w1595, "Array sequence in"=w1596) -> ("Array sequence out"=w1593:cluster{"Timing 0":dbl[]}[])
            }
            n736 = Look In Map(map=w1520, key="None") -> (value=w1519:i32)  [unwired: 1 in, 1 out]
            n737 = call "Add_to_sequence_SubVI_v1.vi"("Delay [us]"=w1517, "Pulse length [us]"=w1518, "Channel number"=w1519, "Array sequence in"=w1522) -> ("Array sequence out"=w1516:cluster{"Timing 0":dbl[]}[])
            n738 = Look In Map(map=w1524, key="Probe") -> (value=w1534:dbl)  [unwired: 1 in, 1 out]
            n739 = Look In Map(map=w1524, key="Delay") -> (value=w1538:dbl)  [unwired: 1 in, 1 out]
            n740 = Look In Map(map=w1520, key="Accqusition TRIG") -> (value=w1536:i32)  [unwired: 1 in, 1 out]
            n741 = Look In Map(map=w1524, key="TTL") -> (value=w1537:dbl)  [unwired: 1 in, 1 out]
            n742 = for {
              tunnel: w1516 -> [w1547] mode=indexing
              tunnel: w1537 -> [w1546]
              tunnel: [w1545] -> w1535 mode=indexing
              tunnel: w1536 -> [w1544]
              i -> [w1543]
              n743 = Equal?(x=w1544, y=w1543) -> (x = y?=w1548:bool)
              n744 = case shown="True" w1548 {
                tunnel: w1547 -> [w1549 w1552]
                tunnel: w1546 -> [_ w1551]
                tunnel: [w1549 w1550] -> w1545
                frame False {
                }
                frame True {
                  n745 = in-place {
                    in-place-border: w1551 -> [w1553]
                    n746 = in-place-cluster #17(w1552) -> ("Timing 0"=w1554:dbl[])
                    n747 = Build Array (concatenate)(w1554, w1553) -> (w1555:dbl[])
                    n748 = in-place-cluster #17("Timing 0"=w1555) -> (w1550:cluster{"Timing 0":dbl[]})
                  }
                }
              }
            }
            n749 = Look In Map(map=w1520, key="Keithley TRIG") -> (value=w1531:i32)  [unwired: 1 in, 1 out]
            n750 = for {
              tunnel: w1535 -> [w1576] mode=indexing
              tunnel: w1531 -> [w1578]
              tunnel: w1537 -> [w1575]
              tunnel: w1538 -> [w1574]
              tunnel: [w1573] -> w1533 mode=indexing
              i -> [w1579]
              n751 = Equal?(x=w1579, y=w1578) -> (x = y?=w1577:bool)
              n752 = case shown="True" w1577 {
                tunnel: w1576 -> [w1580 w1584]
                tunnel: w1575 -> [_ w1583]
                tunnel: w1574 -> [_ w1582]
                tunnel: [w1580 w1581] -> w1573
                frame False {
                }
                frame True {
                  n753 = in-place {
                    in-place-border: w1583 -> [w1588]
                    in-place-border: w1582 -> [w1587]
                    n754 = in-place-cluster #18(w1584) -> ("Timing 0"=w1590:dbl[])
                    n755 = Multiply(x=2.0, y=w1587) -> (x*y=w1585:dbl)
                    n756 = Build Array (concatenate)(w1590, 0.0, w1585, w1588) -> (w1591:dbl[])
                    n757 = in-place-cluster #18("Timing 0"=w1591) -> (w1581:cluster{"Timing 0":dbl[]})
                  }
                }
              }
            }
            n758 = Look In Map(map=w1520, key="LD probe") -> (value=w1532:i32)  [unwired: 1 in, 1 out]
            n759 = for {
              tunnel: w1532 -> [w1561]
              tunnel: w1533 -> [w1559] mode=indexing
              tunnel: w1534 -> [w1558]
              tunnel: [w1557] -> w1523 mode=indexing
              tunnel: w1538 -> [w1556]
              i -> [w1562]
              n760 = Equal?(x=w1562, y=w1561) -> (x = y?=w1560:bool)
              n761 = case shown="True" w1560 {
                tunnel: w1559 -> [w1563 w1567]
                tunnel: [w1563 w1566] -> w1557
                tunnel: w1558 -> [_ w1565]
                tunnel: w1556 -> [_ w1564]
                frame False {
                }
                frame True {
                  n762 = in-place {
                    in-place-border: w1565 -> [w1568]
                    in-place-border: w1564 -> [w1569]
                    n763 = in-place-cluster #19(w1567) -> ("Timing 0"=w1571:dbl[])
                    n764 = Build Array (concatenate)(w1571, 0.0, w1569, w1568) -> (w1572:dbl[])
                    n765 = in-place-cluster #19("Timing 0"=w1572) -> (w1566:cluster{"Timing 0":dbl[]})
                  }
                }
              }
            }
          }
        }
        n766 = flat-sequence {
          frame #0 {
            n767 = Wait (ms)(milliseconds to wait=u32 150) -> ()  [unwired: 1 out]
          }
          frame #1 {
            n768 = invoke on="Save for tomography" class="Bool (strict)" method="Reinit To Default"() -> ()  [unwired: 3 in, 3 out]
          }
        }
        n769 = for {
          tunnel: w1474 -> [w1501] mode=indexing
          shift-right: [w1489] -> w1472
          shift-left: w1473 -> [w1499]
          i -> [w1494]
          n770 = local read "Config folder"() -> (w1496:string)
          n771 = Number To Decimal String(number=w1494, width (-)=i16 1) -> (decimal integer string=w1492:string)
          n772 = call "Array_to_cluster_sequence_SubVI_v1.vi"("Array"=w1501) -> ("Sequence"=w1500:T6)
          n773 = local read "Sampling data"() -> (w1498:T2)
          n774 = Concatenate Strings(w1496, "\\tomography\\pulse_seq_DAQ_" ("string"), w1492, ".ini" ("string")) -> (w1490:string)
          n775 = call "Set_Pulse_Seq_DAQ.vi"("Time Unit"=T12 {"Time Unit"=enum."MicroSecond"}, "error in"=w1499, "Sampling data"=w1498, "Sequence"=w1500, "Filename (ini)"=w1490) -> ("error out"=w1489:errorcluster)  [unwired: 6 in]
        }
      }
      event "Save initial state": Mouse Down {
        n776 = event-data() -> ()  [unwired: 1 in, 8 out]
        n777 = String Length(string="Name of state (initial_state_)") -> (length=w1622:i32)
        n778 = Greater Than 0?(x=w1622) -> (x > 0?=w1621:bool)
        n779 = case shown="False" w1621 {
          tunnel: "Name of state (initial_state_)" -> [_ w1643]
          tunnel: [w1630 w1636] -> w1619
          tunnel: w1618 -> [w1629 w1637]
          tunnel: w1617 -> [w1628 w1638]
          frame False {
            # "Select a Name from the Ring to Save the initial_state in the State_library"
            n780 = property on="Name of initial_state" class="Ring (strict)"() -> ("Strings []"=w1635:string[])  [unwired: 2 in, 2 out]
            n781 = Index Array(array=w1635, index="Name of initial_state") -> (element=w1632:string)
            n782 = call "Array_to_cluster_sequence_SubVI_v1.vi"("Array"=w1628) -> ("Sequence"=w1627:T6)
            n783 = local read "Config folder"() -> (w1623:string)
            n784 = local read "Sampling data"() -> (w1626:T2)
            n785 = Concatenate Strings(w1623, "\\state_library\\" ("string"), w1632, ".ini" ("string")) -> (w1625:string)
            n786 = call "Set_Pulse_Seq_DAQ.vi"("Time Unit"=T12 {"Time Unit"=enum."MicroSecond"}, "error in"=w1629, "Sampling data"=w1626, "Sequence"=w1627, "Filename (ini)"=w1625) -> ("error out"=w1630:errorcluster)  [unwired: 6 in]
          }
          frame True {
            w1640 = "initial_state_" ("true string")
            n787 = Match True/False String(2:"" ("false string"), 3:w1640, 4:w1643) -> (0:w1641:bool, 1:w1639:string)
            n788 = case shown="True" w1641 {
              tunnel: w1640 -> [_ w1663]
              tunnel: w1639 -> [_ w1662]
              tunnel: w1638 -> [_ w1661]
              tunnel: w1637 -> [w1644 w1654]
              tunnel: [w1644 w1653] -> w1636
              frame False {
                n789 = xnode "Error Ring"() -> ("error out"=w1645:errorcluster)
                n790 = call <vilib>:"Simple Error Handler.vi"("error in (no error)"=w1645) -> ()  [unwired: 4 in, 5 out]
              }
              frame True {
                # "input the name by yourself, but name pattern should be like initial_satae_"
                n791 = Concatenate Strings(w1663, w1662) -> (w1657:string)
                n792 = call "Array_to_cluster_sequence_SubVI_v1.vi"("Array"=w1661) -> ("Sequence"=w1660:T6)
                n793 = local read "Config folder"() -> (w1651:string)
                n794 = local read "Sampling data"() -> (w1655:T2)
                n795 = Concatenate Strings(w1651, "\\state_library\\" ("string"), w1657, ".ini" ("string")) -> (w1656:string)
                n796 = call "Set_Pulse_Seq_DAQ.vi"("Time Unit"=T12 {"Time Unit"=enum."MicroSecond"}, "error in"=w1654, "Sampling data"=w1655, "Sequence"=w1660, "Filename (ini)"=w1656) -> ("error out"=w1653:errorcluster)  [unwired: 6 in]
              }
            }
          }
        }
      }
      event "Save  process": Mouse Down {
        n797 = event-data() -> ()  [unwired: 1 in, 8 out]
        n798 = String Length(string="Name of process (process_)") -> (length=w1669:i32)
        n799 = Greater Than 0?(x=w1669) -> (x > 0?=w1668:bool)
        n800 = case shown="True" w1668 {
          tunnel: "Name of process (process_)" -> [_ w1690]
          tunnel: [w1677 w1683] -> w1666
          tunnel: w1665 -> [w1676 w1684]
          tunnel: w1664 -> [w1675 w1685]
          frame False {
            # "Select a Name from the Ring to Save the process in the processes"
            n801 = property on="Name of process" class="Ring (strict)"() -> ("Strings []"=w1682:string[])  [unwired: 2 in, 2 out]
            n802 = Index Array(array=w1682, index="Name of process") -> (element=w1679:string)
            n803 = call "Array_to_cluster_sequence_SubVI_v1.vi"("Array"=w1675) -> ("Sequence"=w1674:T6)
            n804 = local read "Config folder"() -> (w1670:string)
            n805 = local read "Sampling data"() -> (w1673:T2)
            n806 = Concatenate Strings(w1670, "\\process_library\\" ("string"), w1679, ".ini" ("string")) -> (w1672:string)
            n807 = call "Set_Pulse_Seq_DAQ.vi"("Time Unit"=T12 {"Time Unit"=enum."MicroSecond"}, "error in"=w1676, "Sampling data"=w1673, "Sequence"=w1674, "Filename (ini)"=w1672) -> ("error out"=w1677:errorcluster)  [unwired: 6 in]
          }
          frame True {
            w1687 = "process_" ("true string")
            n808 = Match True/False String(2:"" ("false string"), 3:w1687, 4:w1690) -> (0:w1688:bool, 1:w1686:string)
            n809 = case shown="True" w1688 {
              tunnel: w1687 -> [_ w1710]
              tunnel: w1686 -> [_ w1709]
              tunnel: w1685 -> [_ w1708]
              tunnel: w1684 -> [w1691 w1701]
              tunnel: [w1691 w1700] -> w1683
              frame False {
                n810 = xnode "Error Ring"() -> ("error out"=w1692:errorcluster)
                n811 = call <vilib>:"Simple Error Handler.vi"("error in (no error)"=w1692) -> ()  [unwired: 4 in, 5 out]
              }
              frame True {
                # "input the name by yourself, but name pattern should be like process_"
                n812 = Concatenate Strings(w1710, w1709) -> (w1704:string)
                n813 = call "Array_to_cluster_sequence_SubVI_v1.vi"("Array"=w1708) -> ("Sequence"=w1707:T6)
                n814 = local read "Config folder"() -> (w1698:string)
                n815 = local read "Sampling data"() -> (w1702:T2)
                n816 = Concatenate Strings(w1698, "\\process_library\\" ("string"), w1704, ".ini" ("string")) -> (w1703:string)
                n817 = call "Set_Pulse_Seq_DAQ.vi"("Time Unit"=T12 {"Time Unit"=enum."MicroSecond"}, "error in"=w1701, "Sampling data"=w1702, "Sequence"=w1707, "Filename (ini)"=w1703) -> ("error out"=w1700:errorcluster)  [unwired: 6 in]
              }
            }
          }
        }
      }
      event "Save QPT": Mouse Down {
        w1733 = "\\process\\init_states_sets\\" ("string")
        # "1. Clear all files in the temp_states"
        n818 = event-data() -> ()  [unwired: 1 in, 8 out]
        n819 = local read "Config folder"() -> (w1717:string)
        n820 = Concatenate Strings(w1717, "\\process\\temp_states\\" ("string")) -> (w1722:string)
        n821 = Concatenate Strings(w1717, "\\process\\processes_sets\\" ("string")) -> (w1716:string)
        n822 = Concatenate Strings("Config_Files\\" ("string"), w1722) -> (w1726:string)
        n823 = call "Read_filename.vi"("error in"=w1720, "Filename (ini)"=w1716) -> ("error out"=w1715:errorcluster, "Strings []"=w1718:string[])  [unwired: 8 in]
        n824 = call <vilib>:"Application Directory.vi"() -> ("Application Directory"=w1729:path)
        n825 = String To Path(string=w1726) -> (path=w1728:path)
        n826 = Build Path(base path=w1729, name or relative path=w1728) -> (appended path=w1727:path)
        n827 = Array Size(array=w1718) -> (size(s)=w1719:i32)
        n828 = Concatenate Strings(w1717, w1733) -> (w1735:string)
        n829 = call <userlib>:"List Directory__ogtk.vi"("directory path"=w1727) -> ("file names"=w1724:string[])  [unwired: 3 in, 3 out]
        n830 = for {
          tunnel: w1724 -> [w1809] mode=indexing
          shift-right: [w1810] -> w1723
          shift-left: w1720 -> [w1811]
          tunnel: w1722 -> [w1808]
          n831 = Concatenate Strings(w1808, w1809) -> (w1812:string)
          n832 = call "Delete_file.vi"("error in"=w1811, "Filename (ini)"=w1812) -> ("error out"=w1810:errorcluster)  [unwired: 9 in]
        }
        n833 = call "Read_filename.vi"("error in"=w1723, "Filename (ini)"=w1735) -> ("error out"=w1731:errorcluster, "Strings []"=w1732:string[])  [unwired: 8 in]
        n834 = for {
          N: w1719 -> [_]
          tunnel: w1718 -> [w1806] mode=indexing
          tunnel: w1716 -> [w1807]
          shift-right: [w1803] -> w1712
          shift-left: w1715 -> [w1804]
          tunnel: [w1801] -> w1711 mode=indexing
          n835 = Concatenate Strings(w1807, w1806) -> (w1805:string)
          n836 = call "Get_Pulse_Seq_DAQ.vi"("error in"=w1804, "Filename (ini)"=w1805) -> ("error out"=w1803:errorcluster, "data"=w1802:T6)  [unwired: 8 in]
          n837 = call "Squence_to_Array_SubVI.vi"("Sequence"=w1802) -> ("Array"=w1801:cluster{"Timing 0":dbl[]}[])  [unwired: 10 in]
        }
        n838 = Array Size(array=w1732) -> (size(s)=w1734:i32)
        "Initial State Numbers" <- w1734
        n839 = Initialize Array(0.0 ("element"), w1734) -> (w1741:dbl[])
        n840 = for {
          N: w1734 -> [_]
          shift-right: [w1839] -> w1714
          shift-left: w1731 -> [w1841]
          shift-right: [w1831] -> w1739
          shift-left: w1741 -> [w1833]
          tunnel: [w1828] -> w1740 mode=indexing
          tunnel: w1717 -> [w1826]
          tunnel: w1733 -> [w1825]
          tunnel: w1732 -> [w1824] mode=indexing
          i -> [w1832]
          # "3.Look for the longest Time Sequence from the initial_State"
          # "2.Read the initial_state data from the files"
          n841 = Concatenate Strings(w1826, w1825, w1824) -> (w1840:string)
          n842 = call "Get_Pulse_Seq_DAQ.vi"("error in"=w1841, "Filename (ini)"=w1840) -> ("error out"=w1839:errorcluster, "data"=w1838:T6)  [unwired: 8 in]
          n843 = call "Squence_to_Array_SubVI.vi"("Sequence"=w1838) -> ("Array"=w1828:cluster{"Timing 0":dbl[]}[])  [unwired: 10 in]
          n844 = Index Array(array=w1828, index=0) -> (element=w1835:cluster{"Timing 0":dbl[]})
          n845 = Unbundle(w1835) -> ("Timing 0"=w1836:dbl[])
          n846 = for {
            tunnel: w1836 -> [w1843] mode=indexing
            shift-right: [w1842] -> w1829
            shift-left: 0 -> [w1844]
            n847 = Add(x=w1843, y=w1844) -> (x+y=w1842:dbl)
          }
          n848 = local read "MaxTime"() -> (w1830:dbl)
          n849 = Max & Min(x=w1830, y=w1829) -> (max(x,y)=w1834:dbl)  [unwired: 1 out]
          n850 = Replace Array Subset(array=w1833, new element=w1829, index=w1832) -> (w1831:dbl[])
          n851 = local write "MaxTime"(w1834) -> ()
        }
        n852 = for {
          tunnel: w1740 -> [w1823] mode=indexing
          tunnel: w1739 -> [w1813] mode=indexing
          tunnel: [w1821] -> w1738 mode=indexing
          tunnel: w1737 -> [w1820]
          tunnel: w1736 -> [w1817]
          # "4. Add the delay time according to the longest Time sequence"
          n853 = local read "MaxTime"() -> (w1814:dbl)
          n854 = Subtract(x=w1814, y=w1813) -> (x-y=w1822:dbl)
          n855 = Look In Map(map=w1820, key="None") -> (value=w1818:i32)  [unwired: 1 in, 1 out]
          n856 = Look In Map(map=w1817, key="Delay") -> (value=w1815:dbl)  [unwired: 1 in, 1 out]
          n857 = call "Add_to_sequence_SubVI_v1.vi"("Delay [us]"=w1815, "Pulse length [us]"=w1822, "Channel number"=w1818, "Array sequence in"=w1823) -> ("Array sequence out"=w1821:cluster{"Timing 0":dbl[]}[])
        }
        n858 = Merge Errors(w1714, w1712) -> (w1713:errorcluster)
        n859 = for {
          tunnel: w1738 -> [w1749]
          tunnel: w1737 -> [w1748]
          tunnel: w1736 -> [w1747]
          shift-right: [w1750] -> w1743
          shift-left: w1713 -> [w1746]
          tunnel: w1711 -> [w1745] mode=indexing
          i -> [w1744]
          n860 = for {
            shift-right: [w1768] -> w1750
            shift-left: w1746 -> [w1763]
            tunnel: w1749 -> [w1762] mode=indexing
            tunnel: w1748 -> [w1759]
            tunnel: w1747 -> [w1760]
            tunnel: w1745 -> [w1758]
            tunnel: w1744 -> [w1757]
            i -> [w1761]
            # "5. Detect the initial_state"
            # "6. Add the Process data to detect the output_state"
            n861 = call "Add_Time_Seq.vi"("Process Array"=w1758, "Initial State Array"=w1762) -> ("Total Array"=w1764:cluster{"Timing 0":dbl[]}[])  [unwired: 9 in]
            n862 = property on="Initial State Numbers" class="DigNum (strict)"() -> ("Value"=w1751:i32)  [unwired: 2 in, 2 out]
            n863 = call "Create_Time_Seq.vi"("pulses"=w1760, "Channels and actions"=w1759, "Array sequence in"=w1762) -> ("Array out"=w1766:cluster{"Timing 0":dbl[]}[][])  [unwired: 8 in]
            n864 = Multiply(x=9, y=2) -> (x*y=w1753:i32)
            n865 = Multiply(x=w1753, y=w1751) -> (x*y=w1756:i32)
            n866 = call "Create_Time_Seq.vi"("pulses"=w1760, "Channels and actions"=w1759, "Array sequence in"=w1764) -> ("Array out"=w1765:cluster{"Timing 0":dbl[]}[][])  [unwired: 8 in]
            n867 = Multiply(x=w1756, y=w1757) -> (x*y=w1755:i32)
            n868 = Insert Into Array(array=w1766, new element=w1765) -> (w1767:cluster{"Timing 0":dbl[]}[][])  [unwired: 2 in]
            n869 = for {
              tunnel: w1767 -> [w1786] mode=indexing
              shift-right: [w1779] -> w1768
              shift-left: w1763 -> [w1780]
              tunnel: w1761 -> [w1777]
              tunnel: w1755 -> [w1770]
              tunnel: w1753 -> [w1772]
              i -> [w1769]
              # "Write the full number in the name to store the data\n 1-->00001     10-->00010      100-->00100\n1000 ---> 01000   10000  -->  10000"
              n870 = local read "Config folder"() -> (w1776:string)
              n871 = Multiply(x=w1772, y=w1777) -> (x*y=w1771:i32)
              n872 = Compound Arithmetic op=ADD(w1769, w1771, w1770) -> (w1773:i32)
              n873 = Equal To 0?(x=w1773) -> (x = 0?=w1775:bool)
              n874 = case shown="False" w1775 {
                tunnel: [w1787 "00000"] -> w1774
                tunnel: w1773 -> [w1791 _]
                frame False {
                  n875 = Logarithm Base 10(1:w1791) -> (0:w1796:dbl)
                  n876 = Number To Decimal String(number=w1791, width (-)=i16 1) -> (decimal integer string=w1789:string)
                  n877 = Round Toward -Infinity(1:w1796) -> (0:w1795:dbl)
                  n878 = Subtract(x=4.0, y=w1795) -> (x-y=w1793:dbl)
                  n879 = for {
                    N: w1793 -> [_]
                    shift-right: [w1797] -> w1788
                    shift-left: "" -> [w1799]
                    n880 = Concatenate Strings(w1799, "0" ("string")) -> (w1797:string)
                  }
                  n881 = Concatenate Strings(w1788, w1789) -> (w1787:string)
                }
                frame True {
                }
              }
              n882 = call "Array_to_cluster_sequence_SubVI_v1.vi"("Array"=w1786) -> ("Sequence"=w1783:T6)
              n883 = local read "Sampling data"() -> (w1778:T2)
              n884 = Concatenate Strings(w1776, "\\process\\temp_states\\QPT_" ("string"), w1774, ".ini" ("string")) -> (w1782:string)
              n885 = call "Set_Pulse_Seq_DAQ.vi"("Time Unit"=T12 {"Time Unit"=enum."MicroSecond"}, "error in"=w1780, "Sampling data"=w1778, "Sequence"=w1783, "Filename (ini)"=w1782) -> ("error out"=w1779:errorcluster)  [unwired: 6 in]
            }
          }
        }
      }
      event "State_update": Mouse Down; "initial_state_show": Value Change {
        w1845 = "Config_Ver_2\\state_library\\"
        n886 = event-data() -> ()  [unwired: 1 in, 4 out]
        n887 = flat-sequence {
          tunnel: w1852 -> [w1860]
          tunnel: [w1859] -> w1854
          tunnel: w1845 -> [w1858]
          tunnel: [w1855] -> w1848
          tunnel: "Config_Files\\" ("string") -> [w1856]
          tunnel: w1845 -> [w1855]
          tunnel: w1854 -> [w1868]
          tunnel: "initial_state_show" -> [w1867]
          tunnel: [w1868] -> w1850
          tunnel: [w1866] -> w1849
          tunnel: w1848 -> [w1866]
          tunnel: [w1865] -> w1847
          tunnel: [w1871] -> w1851
          tunnel: w1850 -> [w1872]
          tunnel: w1849 -> [w1876]
          tunnel: w1847 -> [w1873]
          frame #0 {
            # "Open the state_library to the show the files"
            n888 = Concatenate Strings(w1856, w1858) -> (w1857:string)
            n889 = String To Path(string=w1857) -> (path=w1863:path)
            n890 = call <vilib>:"Application Directory.vi"() -> ("Application Directory"=w1864:path)
            n891 = Build Path(base path=w1864, name or relative path=w1863) -> (appended path=w1862:path)
            n892 = call <userlib>:"List Directory__ogtk.vi"("error in (no error)"=w1860, "directory path"=w1862) -> ("error out"=w1859:errorcluster, "file names"=w1861:string[])  [unwired: 2 in, 2 out]
            n893 = property on="initial_state_show" class="Ring (strict)"("Strings []"=w1861) -> ()  [unwired: 2 in, 2 out]
          }
          frame #1 {
            # "Check the initial_states in the Library"
            n894 = property on="initial_state_show" class="Ring (strict)"() -> ("Strings []"=w1869:string[])  [unwired: 2 in, 2 out]
            n895 = Index Array(array=w1869, index=w1867) -> (element=w1865:string)
            n896 = local write "Initial_state_name"(w1865) -> ()
          }
          frame #2 {
            # "Show the Pulse_Sequence"
            n897 = String Length(string=w1873) -> (length=w1875:i32)
            n898 = Concatenate Strings(w1876, w1873) -> (w1870:string)
            n899 = Greater Than 0?(x=w1875) -> (x > 0?=w1874:bool)
            n900 = case shown="True" w1874 {
              tunnel: w1870 -> [_ w1883]
              tunnel: w1872 -> [w1877 w1880]
              tunnel: [w1877 w1879] -> w1871
              frame False {
              }
              frame True {
                n901 = call "Get_Pulse_Seq_DAQ.vi"("error in"=w1880, "Filename (ini)"=w1883) -> ("error out"=w1879:errorcluster, "data"=w1882:T6)  [unwired: 8 in]
                n902 = Cluster To Array(cluster=w1882) -> (array=w1881:cluster{"Timing 0":dbl[]}[])
                n903 = for {
                  tunnel: w1881 -> [w1895] mode=indexing
                  tunnel: [w1884] -> w1878 mode=indexing
                  i -> [w1887]
                  n904 = To Double Precision Float(number=w1887) -> (double precision float=w1891:dbl)
                  n905 = Unbundle By Name(w1895) -> ("Timing 0"=w1894:dbl[])
                  n906 = Initialize Array(0.0 ("element"), 1 ("dimension size")) -> (w1888:dbl[])
                  n907 = Initialize Array(w1891, 1 ("dimension size")) -> (w1892:dbl[])
                  n908 = for {
                    tunnel: w1894 -> [w1897] mode=indexing
                    shift-right: [w1899] -> w1885
                    shift-left: w1892 -> [w1898]
                    shift-right: [w1901] -> w1886
                    shift-left: w1888 -> [w1900]
                    tunnel: w1887 -> [w1896]
                    i -> [w1906]
                    n909 = Quotient & Remainder(x=w1906, y=2) -> (x-y*floor(x/y)=w1904:i32)  [unwired: 1 out]
                    n910 = Equal To 0?(x=w1904) -> (x = 0?=w1903:bool)
                    n911 = Equal To 0?(x=w1897) -> (x = 0?=w1902:bool)
                    n912 = case shown="True" w1903 {
                      tunnel: w1902 -> [_ w1923]
                      tunnel: [w1907 w1922] -> w1901
                      tunnel: w1900 -> [w1909 w1921]
                      tunnel: [w1914 w1920] -> w1899
                      tunnel: w1898 -> [w1915 w1919]
                      tunnel: w1897 -> [w1910 w1918]
                      tunnel: w1896 -> [w1916 w1917]
                      frame False {
                        n913 = Array Size(array=w1909) -> (size(s)=w1913:i32)
                        n914 = Decrement(x=w1913) -> (x-1=w1912:i32)
                        n915 = Index Array(array=w1909, index=w1912) -> (element=w1911:dbl)
                        n916 = Build Array (concatenate)(w1915, w1916) -> (w1914:dbl[])
                        n917 = Add(x=w1910, y=w1911) -> (x+y=w1908:dbl)
                        n918 = Build Array (concatenate)(w1909, w1908) -> (w1907:dbl[])
                      }
                      frame True {
                        n919 = case shown="False" w1923 {
                          tunnel: [w1934 w1939] -> w1922
                          tunnel: w1921 -> [w1928 w1939]
                          tunnel: [w1930 w1938] -> w1920
                          tunnel: w1919 -> [w1937 w1938]
                          tunnel: w1918 -> [w1935 _]
                          tunnel: w1917 -> [w1931 _]
                          frame False {
                            n920 = Array Size(array=w1928) -> (size(s)=w1936:i32)
                            n921 = Add(x=0.5, y=w1931) -> (x+y=w1932:dbl)
                            n922 = Decrement(x=w1936) -> (x-1=w1929:i32)
                            n923 = Index Array(array=w1928, index=w1929) -> (element=w1926:dbl)
                            n924 = Add(x=w1935, y=w1926) -> (x+y=w1925:dbl)
                            n925 = Decrement(x=w1926) -> (x-1=w1927:dbl)
                            n926 = Build Array (concatenate)(w1937, w1931, w1932, w1932, w1931) -> (w1930:dbl[])
                            n927 = Decrement(x=w1925) -> (x-1=w1924:dbl)
                            n928 = Build Array (concatenate)(w1928, w1927, w1926, w1924, w1925) -> (w1934:dbl[])
                          }
                          frame True {
                          }
                        }
                      }
                    }
                  }
                  n929 = Bundle(w1886, w1885) -> (w1884:cluster{dbl[], dbl[]})  [unwired: 1 in]
                }
                "Pulses chart 2" <- w1878
              }
            }
          }
        }
      }
      event "Process_update": Mouse Down; "Process_show": Value Change {
        n930 = event-data() -> ()  [unwired: 1 in, 4 out]
        n931 = flat-sequence {
          tunnel: w1947 -> [w1954]
          tunnel: [w1953] -> w1949
          tunnel: "Config_Ver_2\\process_library\\" -> [w1950]
          tunnel: [w1950] -> w1943
          tunnel: "Config_Files\\" ("string") -> [w1951]
          tunnel: w1949 -> [w1962]
          tunnel: "Process_show" -> [w1961]
          tunnel: [w1962] -> w1945
          tunnel: [w1960] -> w1944
          tunnel: w1943 -> [w1960]
          tunnel: [w1959] -> w1942
          tunnel: w1945 -> [w1970]
          tunnel: w1944 -> [w1967]
          tunnel: w1942 -> [w1966]
          tunnel: [w1969] -> w1940
          frame #0 {
            # "Open the processes to the show the files"
            n932 = Concatenate Strings(w1951, w1950) -> (w1952:string)
            n933 = String To Path(string=w1952) -> (path=w1957:path)
            n934 = call <vilib>:"Application Directory.vi"() -> ("Application Directory"=w1958:path)
            n935 = Build Path(base path=w1958, name or relative path=w1957) -> (appended path=w1956:path)
            n936 = call <userlib>:"List Directory__ogtk.vi"("error in (no error)"=w1954, "directory path"=w1956) -> ("error out"=w1953:errorcluster, "file names"=w1955:string[])  [unwired: 2 in, 2 out]
            n937 = property on="Process_show" class="Ring (strict)"("Strings []"=w1955) -> ()  [unwired: 2 in, 2 out]
          }
          frame #1 {
            n938 = property on="Process_show" class="Ring (strict)"() -> ("Strings []"=w1963:string[])  [unwired: 2 in, 2 out]
            n939 = Index Array(array=w1963, index=w1961) -> (element=w1959:string)
            n940 = local write "Process name"(w1959) -> ()
          }
          frame #2 {
            n941 = String Length(string=w1966) -> (length=w1968:i32)
            n942 = Concatenate Strings(w1967, w1966) -> (w1964:string)
            n943 = Greater Than 0?(x=w1968) -> (x > 0?=w1965:bool)
            n944 = case shown="False" w1965 {
              tunnel: w1964 -> [_ w1977]
              tunnel: w1970 -> [w1971 w1974]
              tunnel: [w1971 w1973] -> w1969
              frame False {
              }
              frame True {
                n945 = call "Get_Pulse_Seq_DAQ.vi"("error in"=w1974, "Filename (ini)"=w1977) -> ("error out"=w1973:errorcluster, "data"=w1976:T6)  [unwired: 8 in]
                n946 = Cluster To Array(cluster=w1976) -> (array=w1975:cluster{"Timing 0":dbl[]}[])
                n947 = for {
                  tunnel: w1975 -> [w1989] mode=indexing
                  tunnel: [w1978] -> w1972 mode=indexing
                  i -> [w1981]
                  n948 = To Double Precision Float(number=w1981) -> (double precision float=w1985:dbl)
                  n949 = Unbundle By Name(w1989) -> ("Timing 0"=w1988:dbl[])
                  n950 = Initialize Array(0.0 ("element"), 1 ("dimension size")) -> (w1982:dbl[])
                  n951 = Initialize Array(w1985, 1 ("dimension size")) -> (w1986:dbl[])
                  n952 = for {
                    tunnel: w1988 -> [w1991] mode=indexing
                    shift-right: [w1993] -> w1979
                    shift-left: w1986 -> [w1992]
                    shift-right: [w1995] -> w1980
                    shift-left: w1982 -> [w1994]
                    tunnel: w1981 -> [w1990]
                    i -> [w2000]
                    n953 = Quotient & Remainder(x=w2000, y=2) -> (x-y*floor(x/y)=w1998:i32)  [unwired: 1 out]
                    n954 = Equal To 0?(x=w1998) -> (x = 0?=w1997:bool)
                    n955 = Equal To 0?(x=w1991) -> (x = 0?=w1996:bool)
                    n956 = case shown="False" w1997 {
                      tunnel: w1996 -> [_ w2017]
                      tunnel: [w2001 w2016] -> w1995
                      tunnel: w1994 -> [w2003 w2015]
                      tunnel: [w2008 w2014] -> w1993
                      tunnel: w1992 -> [w2009 w2013]
                      tunnel: w1991 -> [w2004 w2012]
                      tunnel: w1990 -> [w2010 w2011]
                      frame False {
                        n957 = Array Size(array=w2003) -> (size(s)=w2007:i32)
                        n958 = Decrement(x=w2007) -> (x-1=w2006:i32)
                        n959 = Index Array(array=w2003, index=w2006) -> (element=w2005:dbl)
                        n960 = Build Array (concatenate)(w2009, w2010) -> (w2008:dbl[])
                        n961 = Add(x=w2004, y=w2005) -> (x+y=w2002:dbl)
                        n962 = Build Array (concatenate)(w2003, w2002) -> (w2001:dbl[])
                      }
                      frame True {
                        n963 = case shown="True" w2017 {
                          tunnel: [w2028 w2033] -> w2016
                          tunnel: w2015 -> [w2022 w2033]
                          tunnel: [w2024 w2032] -> w2014
                          tunnel: w2013 -> [w2031 w2032]
                          tunnel: w2012 -> [w2029 _]
                          tunnel: w2011 -> [w2025 _]
                          frame False {
                            n964 = Array Size(array=w2022) -> (size(s)=w2030:i32)
                            n965 = Add(x=0.5, y=w2025) -> (x+y=w2026:dbl)
                            n966 = Decrement(x=w2030) -> (x-1=w2023:i32)
                            n967 = Index Array(array=w2022, index=w2023) -> (element=w2020:dbl)
                            n968 = Add(x=w2029, y=w2020) -> (x+y=w2019:dbl)
                            n969 = Decrement(x=w2020) -> (x-1=w2021:dbl)
                            n970 = Build Array (concatenate)(w2031, w2025, w2026, w2026, w2025) -> (w2024:dbl[])
                            n971 = Decrement(x=w2019) -> (x-1=w2018:dbl)
                            n972 = Build Array (concatenate)(w2022, w2021, w2020, w2018, w2019) -> (w2028:dbl[])
                          }
                          frame True {
                          }
                        }
                      }
                    }
                  }
                  n973 = Bundle(w1980, w1979) -> (w1978:cluster{dbl[], dbl[]})  [unwired: 1 in]
                }
                "Pulses chart 3" <- w1972
              }
            }
          }
        }
      }
      event "Choose init states": Mouse Down {
        n974 = event-data() -> ()  [unwired: 1 in, 8 out]
        n975 = local read "Initial_state_name"() -> (w2043:string)
        n976 = local read "Config folder"() -> (w2034:string)
        n977 = String Length(string=w2043) -> (length=w2044:i32)
        n978 = Greater Than 0?(x=w2044) -> (x > 0?=w2035:bool)
        n979 = Concatenate Strings(w2034, "\\state_library\\", w2043) -> (w2037:string)
        n980 = Concatenate Strings(w2034, "\\process\\init_states_sets\\") -> (w2041:string)
        n981 = case shown="True" w2035 {
          tunnel: w2045 -> [w2046 w2056]
          tunnel: w2043 -> [_ w2055]
          tunnel: w2041 -> [_ w2054]
          tunnel: [w2046 w2053] -> w2039
          tunnel: w2037 -> [_ w2052]
          frame False {
          }
          frame True {
            n982 = call "Get_Pulse_Seq_DAQ.vi"("error in"=w2056, "Filename (ini)"=w2052) -> ("error out"=w2050:errorcluster, "data"=w2051:T6)  [unwired: 8 in]
            n983 = local read "Sampling data"() -> (w2049:T2)
            n984 = Concatenate Strings(w2054, w2055) -> (w2047:string)
            n985 = call "Set_Pulse_Seq_DAQ.vi"("Time Unit"=T12 {"Time Unit"=enum."MicroSecond"}, "error in"=w2050, "Sampling data"=w2049, "Sequence"=w2051, "Filename (ini)"=w2047) -> ("error out"=w2053:errorcluster)  [unwired: 6 in]
          }
        }
        n986 = call "Read_filename.vi"("error in"=w2039, "Filename (ini)"=w2041) -> ("error out"=w2040:errorcluster, "Strings []"=w2042:string[])  [unwired: 8 in]
        n987 = local write "State_List"(w2042) -> ()
      }
      event "Choose the Process": Mouse Down {
        n988 = event-data() -> ()  [unwired: 1 in, 8 out]
        n989 = local read "Process name"() -> (w2066:string)
        n990 = local read "Config folder"() -> (w2057:string)
        n991 = String Length(string=w2066) -> (length=w2067:i32)
        n992 = Greater Than 0?(x=w2067) -> (x > 0?=w2058:bool)
        n993 = Concatenate Strings(w2057, "\\process_library\\", w2066) -> (w2060:string)
        n994 = Concatenate Strings(w2057, "\\process\\processes_sets\\") -> (w2064:string)
        n995 = case shown="True" w2058 {
          tunnel: w2068 -> [w2069 w2079]
          tunnel: w2066 -> [_ w2078]
          tunnel: w2064 -> [_ w2077]
          tunnel: [w2069 w2076] -> w2062
          tunnel: w2060 -> [_ w2075]
          frame False {
          }
          frame True {
            n996 = call "Get_Pulse_Seq_DAQ.vi"("error in"=w2079, "Filename (ini)"=w2075) -> ("error out"=w2073:errorcluster, "data"=w2074:T6)  [unwired: 8 in]
            n997 = local read "Sampling data"() -> (w2072:T2)
            n998 = Concatenate Strings(w2077, w2078) -> (w2070:string)
            n999 = call "Set_Pulse_Seq_DAQ.vi"("Time Unit"=T12 {"Time Unit"=enum."MicroSecond"}, "error in"=w2073, "Sampling data"=w2072, "Sequence"=w2074, "Filename (ini)"=w2070) -> ("error out"=w2076:errorcluster)  [unwired: 6 in]
          }
        }
        n1000 = call "Read_filename.vi"("error in"=w2062, "Filename (ini)"=w2064) -> ("error out"=w2063:errorcluster, "Strings []"=w2065:string[])  [unwired: 8 in]
        n1001 = local write "Process_List"(w2065) -> ()
      }
      event "Delete init states": Mouse Down {
        # "Check the name if it's in the State_list, if yes, the name will be deleted, otherwise, return"
        n1002 = event-data() -> ()  [unwired: 1 in, 8 out]
        n1003 = local read "Initial_state_name"() -> (w2085:string)
        n1004 = local read "Config folder"() -> (w2080:string)
        n1005 = local read "State_List"() -> (w2087:string[])
        n1006 = Concatenate Strings(w2080, "\\process\\init_states_sets\\") -> (w2088:string)
        n1007 = for {
          tunnel: w2087 -> [w2100] mode=indexing
          shift-right: [w2096] -> w2084
          shift-left: FALSE -> [w2097]
          tunnel: w2085 -> [w2099]
          n1008 = Equal?(x=w2099, y=w2100) -> (x = y?=w2098:bool)
          n1009 = Or(x=w2097, y=w2098) -> (x .or. y?=w2096:bool)
        }
        n1010 = Concatenate Strings(w2088, w2085) -> (w2081:string)
        n1011 = case shown="True" w2084 {
          tunnel: w2083 -> [w2092 w2093]
          tunnel: [w2092 w2095] -> w2082
          tunnel: w2081 -> [_ w2094]
          frame False {
          }
          frame True {
            n1012 = call "Delete_file.vi"("error in"=w2093, "Filename (ini)"=w2094) -> ("error out"=w2095:errorcluster)  [unwired: 9 in]
          }
        }
        n1013 = call "Read_filename.vi"("error in"=w2082, "Filename (ini)"=w2088) -> ("error out"=w2090:errorcluster, "Strings []"=w2091:string[])  [unwired: 8 in]
        n1014 = local write "State_List"(w2091) -> ()
      }
      event "Delete the Process": Mouse Down {
        # "Check the name if it's in the State_list, if yes, the name will be deleted, otherwise, return"
        n1015 = event-data() -> ()  [unwired: 1 in, 8 out]
        n1016 = local read "Process name"() -> (w2106:string)
        n1017 = local read "Config folder"() -> (w2101:string)
        n1018 = local read "Process_List"() -> (w2108:string[])
        n1019 = Concatenate Strings(w2101, "\\process\\processes_sets\\") -> (w2109:string)
        n1020 = for {
          tunnel: w2108 -> [w2121] mode=indexing
          shift-right: [w2117] -> w2105
          shift-left: FALSE -> [w2118]
          tunnel: w2106 -> [w2120]
          n1021 = Equal?(x=w2120, y=w2121) -> (x = y?=w2119:bool)
          n1022 = Or(x=w2118, y=w2119) -> (x .or. y?=w2117:bool)
        }
        n1023 = Concatenate Strings(w2109, w2106) -> (w2102:string)
        n1024 = case shown="True" w2105 {
          tunnel: w2104 -> [w2113 w2114]
          tunnel: [w2113 w2116] -> w2103
          tunnel: w2102 -> [_ w2115]
          frame False {
          }
          frame True {
            n1025 = call "Delete_file.vi"("error in"=w2114, "Filename (ini)"=w2115) -> ("error out"=w2116:errorcluster)  [unwired: 9 in]
          }
        }
        n1026 = call "Read_filename.vi"("error in"=w2103, "Filename (ini)"=w2109) -> ("error out"=w2111:errorcluster, "Strings []"=w2112:string[])  [unwired: 8 in]
        n1027 = local write "Process_List"(w2112) -> ()
      }
      event "Clear All states": Mouse Down {
        n1028 = event-data() -> ()  [unwired: 1 in, 8 out]
        n1029 = local read "Config folder"() -> (w2129:string)
        n1030 = local read "State_List"() -> (w2128:string[])
        n1031 = Concatenate Strings(w2129, "\\process\\init_states_sets\\") -> (w2123:string)
        n1032 = Array Size(array=w2128) -> (size(s)=w2127:i32)
        n1033 = Greater Than 0?(x=w2127) -> (x > 0?=w2126:bool)
        n1034 = flat-sequence {
          tunnel: w2123 -> [w2135]
          tunnel: w2128 -> [w2134]
          tunnel: w2126 -> [w2133]
          tunnel: w2125 -> [w2132]
          tunnel: [w2131] -> w2124
          tunnel: w2124 -> [w2148]
          tunnel: w2123 -> [w2147]
          tunnel: [w2146] -> w2122
          frame #0 {
            n1035 = case shown="True" w2133 {
              tunnel: w2135 -> [_ w2140]
              tunnel: w2134 -> [_ w2139]
              tunnel: w2132 -> [w2136 w2138]
              tunnel: [w2136 w2137] -> w2131
              frame False {
              }
              frame True {
                n1036 = for {
                  tunnel: w2139 -> [w2144] mode=indexing
                  tunnel: w2140 -> [w2145]
                  shift-right: [w2141] -> w2137
                  shift-left: w2138 -> [w2142]
                  n1037 = Concatenate Strings(w2145, w2144) -> (w2143:string)
                  n1038 = call "Delete_file.vi"("error in"=w2142, "Filename (ini)"=w2143) -> ("error out"=w2141:errorcluster)  [unwired: 9 in]
                }
              }
            }
          }
          frame #1 {
            n1039 = call "Read_filename.vi"("error in"=w2148, "Filename (ini)"=w2147) -> ("error out"=w2146:errorcluster, "Strings []"=w2149:string[])  [unwired: 8 in]
            n1040 = local write "State_List"(w2149) -> ()
          }
        }
      }
      event "Clear All processes": Mouse Down {
        n1041 = event-data() -> ()  [unwired: 1 in, 8 out]
        n1042 = local read "Config folder"() -> (w2157:string)
        n1043 = local read "Process_List"() -> (w2156:string[])
        n1044 = Concatenate Strings(w2157, "\\process\\processes_sets\\") -> (w2151:string)
        n1045 = Array Size(array=w2156) -> (size(s)=w2155:i32)
        n1046 = Greater Than 0?(x=w2155) -> (x > 0?=w2154:bool)
        n1047 = flat-sequence {
          tunnel: w2151 -> [w2163]
          tunnel: w2156 -> [w2162]
          tunnel: w2154 -> [w2161]
          tunnel: w2153 -> [w2160]
          tunnel: [w2159] -> w2152
          tunnel: w2152 -> [w2176]
          tunnel: w2151 -> [w2175]
          tunnel: [w2174] -> w2150
          frame #0 {
            n1048 = case shown="True" w2161 {
              tunnel: w2163 -> [_ w2168]
              tunnel: w2162 -> [_ w2167]
              tunnel: w2160 -> [w2164 w2166]
              tunnel: [w2164 w2165] -> w2159
              frame False {
              }
              frame True {
                n1049 = for {
                  tunnel: w2167 -> [w2172] mode=indexing
                  tunnel: w2168 -> [w2173]
                  shift-right: [w2169] -> w2165
                  shift-left: w2166 -> [w2170]
                  n1050 = Concatenate Strings(w2173, w2172) -> (w2171:string)
                  n1051 = call "Delete_file.vi"("error in"=w2170, "Filename (ini)"=w2171) -> ("error out"=w2169:errorcluster)  [unwired: 9 in]
                }
              }
            }
          }
          frame #1 {
            n1052 = call "Read_filename.vi"("error in"=w2176, "Filename (ini)"=w2175) -> ("error out"=w2174:errorcluster, "Strings []"=w2177:string[])  [unwired: 8 in]
            n1053 = local write "Process_List"(w2177) -> ()
          }
        }
      }
      event "Show init state": Mouse Down {
        n1054 = event-data() -> ()  [unwired: 1 in, 8 out]
        n1055 = local read "Config folder"() -> (w2178:string)
        n1056 = Concatenate Strings(w2178, "\\process\\init_states_sets\\") -> (w2182:string)
        n1057 = call "Read_filename.vi"("error in"=w2181, "Filename (ini)"=w2182) -> ("error out"=w2180:errorcluster, "Strings []"=w2179:string[])  [unwired: 8 in]
        n1058 = local write "State_List"(w2179) -> ()
      }
      event "Show Process_List": Mouse Down {
        n1059 = event-data() -> ()  [unwired: 1 in, 8 out]
        n1060 = local read "Config folder"() -> (w2184:string)
        n1061 = Concatenate Strings(w2184, "\\process\\processes_sets\\") -> (w2188:string)
        n1062 = call "Read_filename.vi"("error in"=w2187, "Filename (ini)"=w2188) -> ("error out"=w2186:errorcluster, "Strings []"=w2185:string[])  [unwired: 8 in]
        n1063 = local write "Process_List"(w2185) -> ()
      }
      event "Reset sequence": Mouse Down {
        n1064 = event-data() -> ()  [unwired: 1 in, 8 out]
        n1065 = Wait (ms)(milliseconds to wait=u32 150) -> ()  [unwired: 1 out]
      }
    }
  }
